vi "SR Service.vi"() -> ()   [LabVIEW 2012]
uses:
  user.lib/SpectralRadar.llb/Probe.lvclass
  user.lib/SpectralRadar.llb/Processing.lvclass
  user.lib/SpectralRadar.llb/Colored Data.lvclass
  user.lib/SpectralRadar.llb/Data.lvclass
  user.lib/SpectralRadar.llb/Scan Pattern.lvclass
  <vilib>/Math Plots/3D Math Plots/3D Surface/3D Surface XCtrl/3D Surface.xctl
  user.lib/SpectralRadar.llb/Device Property Int Selection.ctl
  user.lib/SpectralRadar.llb/Device Property Float Selection.ctl
  user.lib/SpectralRadar.llb/Colorscheme Selection.ctl
  user.lib/SpectralRadar.llb/Processing Flag Selection.ctl
  user.lib/SpectralRadar.llb/Coloring Byteorder.ctl
  <vilib>/Utility/error.llb/DialogType.ctl
  user.lib/SpectralRadar.llb/Probe Parameter Float Selection.ctl
  user.lib/SpectralRadar.llb/Calibration Selection.ctl
  user.lib/SpectralRadar.llb/Processing Parameter Int Selection.ctl
  user.lib/SpectralRadar.llb/Normal Direction Selection.ctl
  user.lib/SpectralRadar.llb/Data Analyzation Selection.ctl
  user.lib/SpectralRadar.llb/A-Scan Analysis Selection.ctl
  user.lib/SpectralRadar.llb/display Data 1D.vi
  user.lib/SpectralRadar.llb/set Scan Output.vi
  user.lib/SpectralRadar.llb/set Apodized Spectrum Output.vi
  user.lib/SpectralRadar.llb/display Data 2D as Surface.vi
  <vilib>/Utility/config.llb/Write Key (Double).vi
  user.lib/SpectralRadar.llb/set Spectrum Output.vi
  user.lib/SpectralRadar.llb/set Offset Corrected Spectrum Output.vi
  <vilib>/Analysis/baseanly.llb/Mean (DBL).vi
  <vilib>/Analysis/5stat.llb/RMS (DBL).vi
  user.lib/SpectralRadar.llb/LabVIEW Helper.lvlib
  user.lib/SpectralRadar.llb/OCT Device.lvclass
  user.lib/SpectralRadar.llb/Raw Data.lvclass
  <vilib>/Utility/config.llb/NI_LVConfig.lvlib
  user.lib/SpectralRadar.llb/ImageField.lvclass
  <vilib>/Analysis/NI_AALPro.lvlib
  user.lib/SpectralRadar.llb/Coloring.lvclass
  user.lib/SpectralRadar.llb/FullRange.lvclass
  <vilib>/Analysis/NI_AALBase.lvlib
panel:
  out "Scan Pattern":refnum<class "Scan Pattern.lvclass">
  out "Camera Image":refnum<class "Colored Data.lvclass">
  out "En face":refnum<class "Data.lvclass">
  out "Volume":refnum<class "Data.lvclass">
  out "Tmp":bool
  out "Colored Data":refnum<class "Colored Data.lvclass">
  out "Processing":refnum<class "Processing.lvclass">
  out "Probe":refnum<class "Probe.lvclass">
  in  "QuitApp":bool
  in  "SLD":bool
  out "SLDIndicator":bool
  in  "Tab Control":T1(tab)
  in  "Camera #":i32 min=0 max=1 step=1
  out "Selected Wavelength [nm]":dbl format="%#.1f"
  in  "Remove DC Spectrum":enum8{"False", "True", "Mixed"}(c332)=enum."True"
  in  "Filter Undersampl.":bool
  in  "Save Dispersion":bool
  in  "Dispersion Comp.":bool
  in  "Dispersion":bool
  in  "Options":bool
  in  "Zero Padding":i32=1 min=1 max=5000
  in  "Binning":i32=1 min=1 max=5000
  in  "SaveSpacingZ":bool
  out "Spacing Z [mm]":dbl format="%#_4g"
  out "Max Intensity":sgl=54929.0 format="%_3p"
  out "Min Intensity":sgl=54929.0 format="%_3p"
  in  "Extended":bool=TRUE
  in  "Dechirp":bool=TRUE
  in  "Apodization":bool=TRUE
  in  "Offset Error":bool=TRUE
  out "-40 dB [µm]":dbl=1600.0880126953125 format="%_3f"
  out "-20 dB [µm]":dbl=1569.837158203125 format="%_3f"
  out "-6 dB [µm]":dbl=1465.10693359375 format="%_3f"
  in  "Thickness Sample":dbl=1.0
  in  "z-Calibration":bool
  out "Noise [dB]":dbl=49.84672927856445 format="%_3f"
  out "Noise [e]":dbl=4474.02978515625 format="%_3p"
  out "Peak Pos. [Pixel]":dbl=474.0 format="%#_5g"
  out "Peak [dB]":dbl=61.309532165527344 format="%#_3g"
  in  "Power in Spectrometer [µW]":dbl=4.6 format="%.2p"
  out "Quantum eff. [%]":dbl=69.93751525878906 format="%.1f"
  out "RMS":dbl=1982809.125 format="%_3p"
  out "Min Contrast [%]":sgl=0.02587428 format="%.1g"
  out "Mean Contrast [%]":dbl=0.08312544226646423 format="%.1g"
  in  "LambdaToKLab":bool
  in  "Apodization":bool
  in  "OffsetErrors":bool
  out "Contrast":sgl[](graph)
  in  "Start Measurement":bool
  out "Meas. Indicator":bool
  out "SpectrumWithOffsetRemoved":dbl[](graph) caption="Spectrum with Offsets Removed"
  out "Apodized Spectrum":dbl[](graph)
  out "Spectrum":dbl[](graph)
  out "AScan":dbl[](graph) caption="A-Scan"
  in  "Window":T2(ring)
  in  "Save Dechirp":bool
  in  "Averaging":i32=1 min=1 max=5000
  in  "Center Wavelength [nm]":dbl=930.0 format="%.2p"
  in  "FullRange":bool
  in  "Log Button":bool
  in  "Clear All":bool
  in  "Select ADC 3":u16(ring) caption="Select ADC" items=["SLD 1 Current", "SLD 1 Peltier", "SLD 1 Power", "SLD 2 Current", "SLD 2 Peltier", "SLD 2 Power"]
  in  "Select ADC 2":u16(ring) caption="Select ADC" items=["SLD 1 Current", "SLD 1 Peltier", "SLD 1 Power", "SLD 2 Current", "SLD 2 Peltier", "SLD 2 Power"]
  in  "Select ADC 1":u16(ring) caption="Select ADC" items=["SLD 1 Current", "SLD 1 Peltier", "SLD 1 Power", "SLD 2 Current", "SLD 2 Peltier", "SLD 2 Power"]
  out "ADC 1":dbl(graph)
  out "ADC 3":dbl(graph)
  out "ADC 2":dbl(graph) caption="SLD1 Power"
  in  "Expansion Time [s]":dbl format="%#_6p"
  in  "Rotation Time [s]":dbl format="%#_6p"
  in  "Flyback Time [s]":dbl format="%#_6p"
  out "Y":dbl[][](graph)=[[-0.12456591788733773, -0.12456591788733773, -0.12456591788733773, -0.12488812549431395, -0.12392150267402412, -0.12424371028057446, -0.12424371028057446, -0.12424371028057446, -0.12456591788733773, -0.12488812549431395, -0.12392150267402412, -0.12359929506768669, -0.12488812549431395, -0.12456591788733773, -0.12392150267402412, -0.12456591788733773, -0.12424371028057446, -0.12392150267402412, -0.12488812549431395, -0.12424371028057446, -0.12424371028057446, -0.12521033310150315, -0.12424371028057446, -0.12392150267402412, -0.12488812549431395, -0.12295487985565048, -0.12424371028057446, -0.12392150267402412, -0.12424371028057446, -0.12488812549431395, -0.12392150267402412, -0.12392150267402412, -0.12456591788733773, -0.12424371028057446, -0.12424371028057446, -0.12392150267402412, -0.12424371028057446, -0.12521033310150315, -0.12392150267402412, -0.12359929506768669, -0.12392150267402412, -0.12424371028057446, -0.12424371028057446, -0.12424371028057446, -0.12392150267402412, -0.12488812549431395, -0.12392150267402412, -0.12424371028057446, -0.12392150267402412, -0.12456591788733773, -0.12456591788733773, -0.12359929506768669, -0.12424371028057446, -0.12456591788733773, -0.12424371028057446, -0.12424371028057446, -0.12488812549431395, -0.12424371028057446, -0.12392150267402412, -0.12392150267402412, -0.12424371028057446, -0.12392150267402412, -0.12553254070890535, -0.12392150267402412, -0.12392150267402412, -0.12488812549431395, -0.12392150267402412, -0.12392150267402412, -0.12392150267402412, -0.12424371028057446, -0.12359929506768669, -0.12392150267402412, -0.12392150267402412, -0.12521033310150315, -0.12359929506768669, -0.12424371028057446, -0.12456591788733773, -0.12424371028057446, -0.12392150267402412, -0.12359929506768669, -0.12424371028057446, -0.12456591788733773, -0.12456591788733773, -0.12392150267402412, -0.12456591788733773, -0.12392150267402412, -0.12392150267402412, -0.12392150267402412, -0.12456591788733773, -0.12456591788733773, -0.12424371028057446, -0.12392150267402412, -0.12456591788733773, -0.12424371028057446, -0.12456591788733773, -0.12359929506768669, -0.12456591788733773, -0.12456591788733773, -0.12392150267402412, -0.12488812549431395, -0.12456591788733773, -0.12456591788733773, -0.12392150267402412, -0.12456591788733773, -0.12456591788733773, -0.12359929506768669, -0.12424371028057446, -0.12359929506768669, -0.12424371028057446, -0.12424371028057446, -0.12424371028057446, -0.12392150267402412, -0.12456591788733773, -0.12488812549431395, -0.12295487985565048, -0.12392150267402412, -0.12456591788733773, -0.12456591788733773, -0.12392150267402412, -0.12424371028057446, -0.12488812549431395, -0.12327708746156214, -0.12456591788733773, -0.12424371028057446, -0.12424371028057446, -0.12424371028057446, -0.12424371028057446, -0.12392150267402412, -0.12392150267402412, -0.12392150267402412, -0.12392150267402412, -0.12392150267402412, -0.12456591788733773, -0.12456591788733773, -0.12392150267402412, -0.12392150267402412, -0.12456591788733773, -0.12359929506768669, -0.12488812549431395, -0.12456591788733773, -0.12295487985565048, -0.12359929506768669, -0.12424371028057446, -0.12392150267402412, -0.12488812549431395, -0.12456591788733773, -0.12392150267402412, -0.12424371028057446, -0.12424371028057446, -0.12392150267402412, -0.12456591788733773, -0.12392150267402412, -0.12488812549431395, -0.12392150267402412, -0.12521033310150315, -0.12424371028057446, -0.12521033310150315, -0.12456591788733773, -0.12392150267402412, -0.12521033310150315, -0.12424371028057446, -0.12424371028057446, -0.12456591788733773, -0.12424371028057446, -0.12456591788733773, -0.12456591788733773, -0.12359929506768669, -0.12488812549431395, -0.12456591788733773, -0.12456591788733773, -0.12424371028057446, -0.12456591788733773, -0.12359929506768669, -0.12424371028057446, -0.12424371028057446, -0.12392150267402412, -0.12456591788733773, -0.12359929506768669, -0.12392150267402412, -0.12521033310150315, -0.12424371028057446, -0.12521033310150315, -0.12456591788733773, -0.12521033310150315, -0.12392150267402412, -0.12488812549431395, -0.12392150267402412, -0.12488812549431395, -0.12456591788733773, -0.12359929506768669, -0.12424371028057446, -0.12456591788733773, -0.12488812549431395, -0.12392150267402412, -0.12456591788733773, -0.12521033310150315, -0.12327708746156214, -0.12456591788733773, -0.12359929506768669, -0.12488812549431395, -0.12392150267402412, -0.12456591788733773, -0.12392150267402412, -0.12456591788733773, -0.12424371028057446, -0.12424371028057446, -0.12424371028057446, -0.12456591788733773, -0.12392150267402412, -0.12392150267402412, -0.12359929506768669, -0.12488812549431395, -0.12456591788733773, -0.12359929506768669, -0.12424371028057446, -0.12392150267402412, -0.12359929506768669, -0.12424371028057446, -0.12392150267402412, -0.12424371028057446, -0.12424371028057446, -0.12424371028057446, -0.12488812549431395, -0.12456591788733773, -0.12424371028057446, -0.12392150267402412, -0.12392150267402412, -0.12456591788733773, -0.12456591788733773, -0.12456591788733773, -0.12456591788733773, -0.12424371028057446, -0.12424371028057446, -0.12359929506768669, -0.12424371028057446, -0.12456591788733773, -0.12327708746156214, -0.12456591788733773, -0.12424371028057446, -0.12456591788733773, -0.12456591788733773, -0.12392150267402412, -0.12424371028057446, -0.12488812549431395, -0.12456591788733773, -0.12359929506768669, -0.12521033310150315, -0.12424371028057446, -0.12327708746156214, -0.12424371028057446, -0.12456591788733773, -0.12392150267402412, -0.12488812549431395, -0.12392150267402412, -0.12392150267402412, -0.12488812549431395, -0.12424371028057446, -0.12392150267402412, -0.12488812549431395, -0.12521033310150315, -0.12456591788733773, -0.12424371028057446, -0.12456591788733773, -0.12424371028057446, -0.12392150267402412, -0.12424371028057446, -0.12359929506768669, -0.12456591788733773, -0.12424371028057446, -0.12424371028057446, -0.12456591788733773, -0.12424371028057446, -0.12392150267402412, -0.12488812549431395, -0.12392150267402412, -0.12392150267402412, -0.12424371028057446, -0.12359929506768669, -0.12521033310150315, -0.12424371028057446, -0.12392150267402412, -0.12424371028057446, -0.12456591788733773, -0.12424371028057446, -0.12521033310150315, -0.12392150267402412, -0.12488812549431395, -0.12521033310150315, -0.12359929506768669, -0.12424371028057446, -0.12488812549431395, -0.12456591788733773, -0.12424371028057446, -0.12424371028057446, -0.12488812549431395, -0.12359929506768669, -0.12327708746156214, -0.12488812549431395, -0.12456591788733773, -0.12424371028057446, -0.12456591788733773, -0.12456591788733773, -0.12456591788733773, -0.12392150267402412, -0.12392150267402412, -0.12392150267402412, -0.12488812549431395, -0.12392150267402412, -0.12424371028057446, -0.12424371028057446, -0.12424371028057446, -0.12424371028057446, -0.12424371028057446, -0.12488812549431395, -0.12392150267402412, -0.12424371028057446, -0.12392150267402412, -0.12424371028057446, -0.12392150267402412, -0.12424371028057446, -0.12392150267402412, -0.12392150267402412, -0.12456591788733773, -0.12424371028057446, -0.12327708746156214, -0.12521033310150315, -0.12392150267402412, -0.12392150267402412, -0.12392150267402412, -0.12456591788733773, -0.12359929506768669, -0.12456591788733773, -0.12424371028057446, -0.12424371028057446, -0.12456591788733773, -0.12392150267402412, -0.12424371028057446, -0.12359929506768669, -0.12456591788733773, -0.12456591788733773, -0.12392150267402412, -0.12424371028057446, -0.12456591788733773, -0.12359929506768669, -0.12488812549431395, -0.12456591788733773, -0.12424371028057446, -0.12424371028057446, -0.12456591788733773, -0.12424371028057446, -0.12424371028057446, -0.12456591788733773, -0.12327708746156214, -0.12392150267402412, -0.12392150267402412, -0.12424371028057446, -0.12359929506768669, -0.12488812549431395, -0.12424371028057446, -0.12424371028057446, -0.12392150267402412, -0.12456591788733773, -0.12424371028057446, -0.12359929506768669, -0.12359929506768669, -0.12456591788733773, -0.12456591788733773, -0.12456591788733773, -0.12392150267402412, -0.12488812549431395, -0.12392150267402412, -0.12424371028057446, -0.12359929506768669, -0.12456591788733773, -0.12424371028057446, -0.12424371028057446, -0.12456591788733773, -0.12424371028057446, -0.12359929506768669, -0.12392150267402412, -0.12456591788733773, -0.12521033310150315, -0.12327708746156214, -0.12392150267402412, -0.12424371028057446, -0.12488812549431395, -0.12424371028057446, -0.12359929506768669, -0.12392150267402412, -0.12488812549431395, -0.12392150267402412, -0.12424371028057446, -0.12392150267402412, -0.12456591788733773, -0.12359929506768669, -0.12424371028057446, -0.12392150267402412, -0.12424371028057446, -0.12456591788733773, -0.12456591788733773, -0.12424371028057446, -0.12456591788733773, -0.12392150267402412, -0.12392150267402412, -0.12424371028057446, -0.12392150267402412, -0.12392150267402412, -0.12424371028057446, -0.12424371028057446, -0.12424371028057446, -0.12424371028057446, -0.12488812549431395, -0.12424371028057446, -0.12392150267402412, -0.12456591788733773, -0.12359929506768669, -0.12488812549431395, -0.12424371028057446, -0.12424371028057446, -0.12521033310150315, -0.12488812549431395, -0.12424371028057446, -0.12456591788733773, -0.12488812549431395, -0.12456591788733773, -0.12488812549431395, -0.12488812549431395, -0.12424371028057446, -0.12424371028057446, -0.12392150267402412, -0.12392150267402412, -0.12392150267402412, -0.12488812549431395, -0.12327708746156214, -0.12553254070890535, -0.12359929506768669, -0.12456591788733773, -0.12456591788733773, -0.12327708746156214, -0.12424371028057446, -0.12456591788733773, -0.12359929506768669, -0.12392150267402412, -0.12424371028057446, -0.12488812549431395, -0.12585474831652058, -0.12359929506768669, -0.12424371028057446, -0.12521033310150315, -0.12327708746156214, -0.12424371028057446, -0.12424371028057446, -0.12392150267402412, -0.12488812549431395, -0.12359929506768669, -0.12456591788733773, -0.12424371028057446, -0.12359929506768669, -0.12456591788733773, -0.12488812549431395, -0.12488812549431395, -0.12456591788733773, -0.12392150267402412, -0.12424371028057446, -0.12392150267402412, -0.12488812549431395, -0.12456591788733773, -0.12392150267402412, -0.12456591788733773, -0.12424371028057446, -0.12392150267402412, -0.12456591788733773, -0.12392150267402412, -0.12327708746156214, -0.12521033310150315, -0.12424371028057446, -0.12424371028057446, -0.12392150267402412, -0.12456591788733773, -0.12392150267402412, -0.12456591788733773, -0.12456591788733773, -0.12327708746156214, -0.12456591788733773, -0.12424371028057446, -0.12392150267402412, -0.12424371028057446, -0.12424371028057446, -0.12424371028057446, -0.12392150267402412, -0.12327708746156214, -0.12456591788733773, -0.12456591788733773, -0.12359929506768669, -0.12456591788733773, -0.12392150267402412, -0.12392150267402412, -0.12488812549431395, -0.12456591788733773, -0.12424371028057446, -0.12488812549431395, -0.12327708746156214, -0.12456591788733773, -0.12456591788733773, -0.12424371028057446, -0.12359929506768669, -0.12392150267402412, -0.12456591788733773, -0.12424371028057446, -0.12392150267402412, -0.12392150267402412, -0.12424371028057446, -0.12456591788733773, -0.12359929506768669, -0.12424371028057446, -0.12521033310150315, -0.12359929506768669, -0.12424371028057446, -0.12359929506768669, -0.12359929506768669, -0.12424371028057446, -0.12424371028057446, -0.12456591788733773, -0.12456591788733773, -0.12456591788733773, -0.12424371028057446, -0.12392150267402412, -0.12488812549431395, -0.12424371028057446, -0.12456591788733773, -0.12424371028057446, -0.12521033310150315, -0.12456591788733773, -0.12456591788733773, -0.12521033310150315, -0.12488812549431395, -0.12456591788733773, -0.12359929506768669, -0.12521033310150315, -0.12456591788733773, -0.12392150267402412, -0.12456591788733773, -0.12359929506768669, -0.12424371028057446, -0.12488812549431395, -0.12392150267402412, -0.12392150267402412, -0.12456591788733773, -0.12456591788733773, -0.12488812549431395, -0.12392150267402412, -0.12424371028057446, -0.12424371028057446, -0.12359929506768669, -0.12392150267402412, -0.12424371028057446, -0.12424371028057446, -0.12456591788733773, -0.12488812549431395, -0.12488812549431395, -0.12456591788733773, -0.12424371028057446, -0.12392150267402412, -0.12456591788733773, -0.12392150267402412, -0.12392150267402412, -0.12488812549431395, -0.12488812549431395, -0.12359929506768669, -0.12424371028057446, -0.12424371028057446, -0.12392150267402412, -0.12456591788733773, -0.12424371028057446, -0.12488812549431395, -0.12521033310150315, -0.12424371028057446, -0.12359929506768669, -0.12456591788733773, -0.12456591788733773, -0.12424371028057446, -0.12424371028057446, -0.12456591788733773, -0.12359929506768669, -0.12424371028057446, -0.12424371028057446, -0.12424371028057446, -0.12456591788733773, -0.12456591788733773, -0.12392150267402412, -0.12456591788733773, -0.12456591788733773, -0.12424371028057446, -0.12359929506768669, -0.12553254070890535, -0.12456591788733773, -0.12456591788733773, -0.12456591788733773, -0.12456591788733773, -0.12392150267402412, -0.12424371028057446, -0.12424371028057446, -0.12488812549431395, -0.12424371028057446, -0.12488812549431395, -0.12392150267402412, -0.12456591788733773, -0.12456591788733773, -0.12456591788733773, -0.12392150267402412, -0.12488812549431395, -0.12392150267402412, -0.12392150267402412, -0.12456591788733773, -0.12424371028057446, -0.12456591788733773, -0.12327708746156214, -0.12488812549431395, -0.12392150267402412, -0.12359929506768669, -0.12488812549431395, -0.12392150267402412, -0.12424371028057446, -0.12456591788733773, -0.12456591788733773, -0.12359929506768669, -0.12488812549431395, -0.12424371028057446, -0.12359929506768669, -0.12456591788733773, -0.12521033310150315, -0.12359929506768669, -0.12456591788733773, -0.12392150267402412, -0.12488812549431395, -0.12327708746156214, -0.12456591788733773, -0.12456591788733773, -0.12392150267402412, -0.12488812549431395, -0.12392150267402412, -0.12456591788733773, -0.12424371028057446, -0.12392150267402412, -0.12359929506768669, -0.12553254070890535, -0.12392150267402412, -0.12424371028057446, -0.12392150267402412, -0.12456591788733773, -0.12424371028057446, -0.12424371028057446, -0.12424371028057446, -0.12456591788733773, -0.12424371028057446, -0.12456591788733773, -0.12424371028057446, -0.12424371028057446, -0.12359929506768669, -0.12392150267402412, -0.12456591788733773, -0.12456591788733773, -0.12488812549431395, -0.12359929506768669, -0.12424371028057446, -0.12456591788733773, -0.12424371028057446, -0.12359929506768669, -0.12327708746156214, -0.12392150267402412, -0.12456591788733773, -0.12392150267402412, -0.12488812549431395, -0.12456591788733773, -0.12392150267402412, -0.12424371028057446, -0.12359929506768669, -0.12456591788733773, -0.12424371028057446, -0.12456591788733773, -0.12392150267402412, -0.12456591788733773, -0.12456591788733773, -0.12424371028057446, -0.12392150267402412, -0.12424371028057446, -0.12359929506768669, -0.12456591788733773, -0.12424371028057446, -0.12488812549431395, -0.12488812549431395, -0.12392150267402412, -0.12424371028057446, -0.12521033310150315, -0.12359929506768669, -0.12327708746156214, -0.12424371028057446, -0.12456591788733773, -0.12456591788733773, -0.12424371028057446, -0.12392150267402412, -0.12521033310150315, -0.12392150267402412, -0.12456591788733773, -0.12424371028057446, -0.12392150267402412, -0.12424371028057446, -0.12488812549431395, -0.12295487985565048, -0.12521033310150315, -0.12424371028057446, -0.12424371028057446, -0.12456591788733773, -0.12456591788733773, -0.12359929506768669, -0.12456591788733773, -0.12424371028057446, -0.12456591788733773, -0.12424371028057446, -0.12327708746156214, -0.12488812549431395, -0.12424371028057446, -0.12392150267402412, -0.12456591788733773, -0.12424371028057446, -0.12424371028057446, -0.12424371028057446, -0.12456591788733773, -0.12424371028057446, -0.12456591788733773, -0.12424371028057446, -0.12359929506768669, -0.12424371028057446, -0.12392150267402412, -0.12392150267402412, -0.12424371028057446, -0.12456591788733773, -0.12392150267402412, -0.12424371028057446, -0.12392150267402412, -0.12424371028057446, -0.12456591788733773, -0.12424371028057446, -0.12456591788733773, -0.12392150267402412, -0.12456591788733773, -0.12521033310150315, -0.12392150267402412, -0.12456591788733773, -0.12488812549431395, -0.12424371028057446, -0.12424371028057446, -0.12392150267402412, -0.12424371028057446, -0.12392150267402412, -0.12424371028057446, -0.12392150267402412, -0.12424371028057446, -0.12424371028057446, -0.12456591788733773, -0.12424371028057446, -0.12359929506768669, -0.12456591788733773, -0.12359929506768669, -0.12456591788733773, -0.12424371028057446, -0.12424371028057446, -0.12359929506768669, -0.12456591788733773, -0.12424371028057446, -0.12392150267402412, -0.12424371028057446, -0.12392150267402412, -0.12392150267402412, -0.12359929506768669, -0.12424371028057446, -0.12456591788733773, -0.12392150267402412, -0.12456591788733773, -0.12392150267402412, -0.12392150267402412, -0.12424371028057446, -0.12456591788733773, -0.12424371028057446, -0.12456591788733773, -0.12392150267402412, -0.12521033310150315, -0.12359929506768669, -0.12456591788733773, -0.12359929506768669, -0.12392150267402412, -0.12488812549431395, -0.12488812549431395, -0.12424371028057446, -0.12456591788733773, -0.12424371028057446, -0.12424371028057446, -0.12424371028057446, -0.12359929506768669, -0.12424371028057446, -0.12456591788733773, -0.12456591788733773, -0.12327708746156214, -0.12424371028057446, -0.12456591788733773, -0.12521033310150315, -0.12424371028057446, -0.12424371028057446, -0.12424371028057446, -0.12456591788733773, -0.12424371028057446, -0.12456591788733773, -0.12456591788733773, -0.12521033310150315, -0.12456591788733773, -0.12392150267402412, -0.12392150267402412, -0.12424371028057446, -0.12327708746156214, -0.12424371028057446, -0.12456591788733773, -0.12424371028057446, -0.12392150267402412, -0.12392150267402412, -0.12424371028057446, -0.12392150267402412, -0.12456591788733773, -0.12488812549431395, -0.12359929506768669, -0.12456591788733773, -0.12424371028057446, -0.12456591788733773, -0.12392150267402412, -0.12456591788733773, -0.12359929506768669, -0.12392150267402412, -0.12456591788733773, -0.12424371028057446, -0.12392150267402412, -0.12456591788733773, -0.12488812549431395, -0.12424371028057446, -0.12359929506768669, -0.12488812549431395, -0.12392150267402412, -0.12424371028057446, -0.12424371028057446, -0.12359929506768669, -0.12456591788733773, -0.12392150267402412, -0.12424371028057446, -0.12488812549431395, -0.12456591788733773, -0.12392150267402412, -0.12488812549431395, -0.12488812549431395, -0.12392150267402412, -0.12424371028057446, -0.12392150267402412, -0.12488812549431395, -0.12392150267402412, -0.12424371028057446, -0.12392150267402412, -0.12488812549431395, -0.12424371028057446, -0.12424371028057446, -0.12456591788733773, -0.12456591788733773, -0.12359929506768669, -0.12521033310150315, -0.12359929506768669, -0.12521033310150315, -0.12424371028057446, -0.12392150267402412, -0.12424371028057446, -0.12456591788733773, -0.12456591788733773, -0.12456591788733773, -0.12359929506768669, -0.12488812549431395, -0.12424371028057446, -0.12392150267402412, -0.12392150267402412, -0.12456591788733773, -0.12424371028057446, -0.12392150267402412, -0.12424371028057446, -0.12521033310150315, -0.12327708746156214, -0.12424371028057446, -0.12359929506768669, -0.12359929506768669, -0.12359929506768669, -0.12424371028057446, -0.12327708746156214, -0.12585474831652058, -0.12456591788733773, -0.12424371028057446, -0.12456591788733773, -0.12392150267402412, -0.12424371028057446, -0.12456591788733773, -0.12392150267402412, -0.12456591788733773, -0.12456591788733773, -0.12327708746156214, -0.12488812549431395, -0.12521033310150315, -0.12392150267402412, -0.12456591788733773, -0.12359929506768669, -0.12521033310150315, -0.12424371028057446, -0.12392150267402412, -0.12424371028057446, -0.12456591788733773, -0.12392150267402412, -0.12521033310150315, -0.12392150267402412, -0.12424371028057446, -0.12424371028057446, -0.12424371028057446, -0.12456591788733773, -0.12424371028057446, -0.12327708746156214, -0.12424371028057446, -0.12424371028057446, -0.12456591788733773, -0.12456591788733773, -0.12392150267402412, -0.12488812549431395, -0.12392150267402412, -0.12392150267402412, -0.12392150267402412, -0.12488812549431395, -0.12488812549431395, -0.12359929506768669, -0.12456591788733773, -0.12424371028057446, -0.12392150267402412, -0.12456591788733773, -0.12456591788733773, -0.12424371028057446, -0.12456591788733773, -0.12424371028057446, -0.12359929506768669, -0.12424371028057446, -0.12456591788733773, -0.12424371028057446, -0.12392150267402412, -0.12488812549431395, -0.12456591788733773, -0.12359929506768669, -0.12456591788733773, -0.12456591788733773, -0.12456591788733773, -0.12392150267402412, -0.12359929506768669, -0.12456591788733773, -0.12424371028057446, -0.12424371028057446, -0.12392150267402412, -0.12456591788733773, -0.12424371028057446, -0.12424371028057446, -0.12424371028057446, -0.12392150267402412, -0.12456591788733773, -0.12424371028057446, -0.12392150267402412, -0.12424371028057446, -0.12392150267402412, -0.12327708746156214, -0.12359929506768669, -0.12424371028057446, -0.12392150267402412, -0.12424371028057446, -0.12488812549431395, -0.12424371028057446, -0.12392150267402412, -0.12456591788733773, -0.12392150267402412, -0.12521033310150315, -0.12392150267402412, -0.12424371028057446, -0.12359929506768669, -0.12456591788733773, -0.12359929506768669, -0.12424371028057446, -0.12392150267402412, -0.12456591788733773, -0.12424371028057446, -0.12359929506768669, -0.12424371028057446, -0.12456591788733773, -0.12424371028057446, -0.12424371028057446, -0.12424371028057446, -0.12488812549431395, -0.12456591788733773, -0.12424371028057446, -0.12456591788733773, -0.12359929506768669, -0.12456591788733773, -0.12456591788733773, -0.12456591788733773, -0.12456591788733773, -0.12359929506768669, -0.12424371028057446, -0.12359929506768669, -0.12327708746156214, -0.12424371028057446, -0.12392150267402412, -0.12488812549431395, -0.12488812549431395, -0.12359929506768669, -0.12456591788733773, -0.12488812549431395, -0.12488812549431395, -0.12392150267402412, -0.12424371028057446, -0.12456591788733773, -0.12424371028057446, -0.12424371028057446, -0.12392150267402412, -0.12617695592434883, -0.12424371028057446, -0.12392150267402412, -0.12359929506768669, -0.12553254070890535, -0.12392150267402412, -0.12424371028057446, -0.12424371028057446, -0.12456591788733773, -0.12392150267402412, -0.12488812549431395, -0.12456591788733773, -0.12424371028057446, -0.12392150267402412, -0.12521033310150315, -0.12359929506768669, -0.12488812549431395, -0.12392150267402412, -0.12456591788733773, -0.12424371028057446, -0.12488812549431395, -0.12456591788733773, -0.12359929506768669, -0.12424371028057446, -0.12521033310150315, -0.12424371028057446, -0.12359929506768669, -0.12392150267402412, -0.12488812549431395, -0.12327708746156214, -0.12456591788733773, -0.12424371028057446, -0.12456591788733773, -0.12456591788733773, -0.12359929506768669, -0.12392150267402412, -0.12456591788733773, -0.12359929506768669, -0.12359929506768669, -0.12456591788733773, -0.12488812549431395, -0.12553254070890535, -0.12456591788733773, -0.12392150267402412, -0.12424371028057446, -0.12327708746156214, -0.12456591788733773, -0.12392150267402412, -0.12424371028057446, -0.12392150267402412, -0.12424371028057446, -0.12424371028057446, -0.12392150267402412, -0.12359929506768669, -0.12456591788733773, -0.12456591788733773, -0.12424371028057446, -0.12392150267402412, -0.12392150267402412, -0.12392150267402412, -0.12424371028057446, -0.12392150267402412, -0.12392150267402412, -0.12488812549431395, -0.12456591788733773, -0.12392150267402412, -0.12456591788733773, -0.12359929506768669, -0.12456591788733773, -0.12359929506768669, -0.12392150267402412, -0.12488812549431395, -0.12456591788733773, -0.12359929506768669, -0.12424371028057446, -0.12392150267402412, -0.12488812549431395, -0.12424371028057446, -0.12488812549431395, -0.12392150267402412, -0.12488812549431395, -0.12488812549431395, -0.12392150267402412, -0.12521033310150315, -0.12424371028057446, -0.12359929506768669, -0.12456591788733773, -0.12456591788733773, -0.12359929506768669, -0.12392150267402412, -0.12392150267402412, -0.12456591788733773, -0.12488812549431395, -0.12295487985565048, -0.12424371028057446, -0.12392150267402412, -0.12359929506768669, -0.12456591788733773, -0.12424371028057446, -0.12456591788733773, -0.12456591788733773, -0.12392150267402412, -0.12392150267402412, -0.12488812549431395, -0.12359929506768669, -0.12456591788733773, -0.12392150267402412, -0.12456591788733773, -0.12488812549431395, -0.12424371028057446, -0.12424371028057446, -0.12424371028057446, -0.12392150267402412, -0.12424371028057446, -0.12424371028057446, -0.12359929506768669, -0.12392150267402412, -0.12392150267402412, -0.12488812549431395, -0.12456591788733773, -0.12424371028057446, -0.12456591788733773, -0.12392150267402412, -0.12456591788733773, -0.12359929506768669, -0.12392150267402412, -0.12392150267402412, -0.12424371028057446, -0.12424371028057446, -0.12488812549431395, -0.12424371028057446, -0.12456591788733773, -0.12392150267402412, -0.12456591788733773, -0.12359929506768669, -0.12424371028057446, -0.12456591788733773, -0.12359929506768669, -0.12456591788733773, -0.12424371028057446, -0.12392150267402412, -0.12456591788733773, -0.12424371028057446, -0.12488812549431395, -0.12359929506768669, -0.12392150267402412, -0.12456591788733773, -0.12456591788733773, -0.12295487985565048, -0.12488812549431395, -0.12456591788733773, -0.12521033310150315, -0.12424371028057446, -0.12392150267402412, -0.12424371028057446, -0.12456591788733773, -0.12456591788733773, -0.12392150267402412, -0.12424371028057446, -0.12488812549431395, -0.12359929506768669, -0.12359929506768669, -0.12456591788733773, -0.12424371028057446, -0.12359929506768669, -0.12359929506768669, -0.12488812549431395, -0.12424371028057446, -0.12456591788733773, -0.12359929506768669, -0.12456591788733773, -0.12521033310150315, -0.12456591788733773, -0.12424371028057446, -0.12456591788733773, -0.12392150267402412, -0.12392150267402412, -0.12392150267402412, -0.12424371028057446, -0.12488812549431395, -0.12392150267402412, -0.12456591788733773, -0.12392150267402412, -0.12424371028057446, -0.12424371028057446, -0.12392150267402412, -0.12392150267402412, -0.12424371028057446, -0.12456591788733773, -0.12456591788733773, -0.12456591788733773, -0.12488812549431395, -0.12424371028057446, -0.12359929506768669, -0.12488812549431395, -0.12424371028057446, -0.12392150267402412, -0.12521033310150315, -0.12424371028057446, -0.12392150267402412, -0.12392150267402412, -0.12456591788733773, -0.12488812549431395, -0.12424371028057446, -0.12424371028057446, -0.12392150267402412, -0.12424371028057446, -0.12456591788733773, -0.12456591788733773, -0.12456591788733773, -0.12424371028057446, -0.12521033310150315, -0.12295487985565048, -0.12456591788733773, -0.12424371028057446, -0.12424371028057446, -0.12392150267402412, -0.12488812549431395], [0.0, 0.0, 0.0, 0.0, 0.0, 0.0, 0.0, 0.0, 0.0, 0.0, 0.0, 0.0, 0.0, 0.0, 0.0, 0.0, 0.0, 0.0, 0.0, 0.0, 0.0, 0.0, 0.0, 0.0, 0.0, 0.0, 0.0, 0.0, 0.0, 0.0, 0.0, 0.0, 0.0, 0.0, 0.0, 0.0, 0.0, 0.0, 0.0, 0.0, 0.0, 0.0, 0.0, 0.0, 0.0, 0.0, 0.0, 0.0, 0.0, 0.0, 0.0, 0.0, 0.0, 0.0, 0.0, 0.0, 0.0, 0.0, 0.0, 0.0, 0.0, 0.0, 0.0, 0.0, 0.0, 0.0, 0.0, 0.0, 0.0, 0.0, 0.0, 0.0, 0.0, 0.0, 0.0, 0.0, 0.0, 0.0, 0.0, 0.0, 0.0, 0.0, 0.0, 0.0, 0.0, 0.0, 0.0, 0.0, 0.0, 0.0, 0.0, 0.0, 0.0, 0.0, 0.0, 0.0, 0.0, 0.0, 0.0, 0.0, 0.0, 0.0, 0.0, 0.0, 0.0, 0.0, 0.0, 0.0, 0.0, 0.0, 0.0, 0.0, 0.0, 0.0, 0.0, 0.0, 0.0, 0.0, 0.0, 0.0, 0.0, 0.0, 0.0, 0.0, 0.0, 0.0, 0.0, 0.0, 0.0, 0.0, 0.0, 0.0, 0.0, 0.0, 0.0, 0.0, 0.0, 0.0, 0.0, 0.0, 0.0, 0.0, 0.0, 0.0, 0.0, 0.0, 0.0, 0.0, 0.0, 0.0, 0.0, 0.0, 0.0, 0.0, 0.0, 0.0, 0.0, 0.0, 0.0, 0.0, 0.0, 0.0, 0.0, 0.0, 0.0, 0.0, 0.0, 0.0, 0.0, 0.0, 0.0, 0.0, 0.0, 0.0, 0.0, 0.0, 0.0, 0.0, 0.0, 0.0, 0.0, 0.0, 0.0, 0.0, 0.0, 0.0, 0.0, 0.0, 0.0, 0.0, 0.0, 0.0, 0.0, 0.0, 0.0, 0.0, 0.0, 0.0, 0.0, 0.0, 0.0, 0.0, 0.0, 0.0, 0.0, 0.0, 0.0, 0.0, 0.0, 0.0, 0.0, 0.0, 0.0, 0.0, 0.0, 0.0, 0.0, 0.0, 0.0, 0.0, 0.0, 0.0, 0.0, 0.0, 0.0, 0.0, 0.0, 0.0, 0.0, 0.0, 0.0, 0.0, 0.0, 0.0, 0.0, 0.0, 0.0, 0.0, 0.0, 0.0, 0.0, 0.0, 0.0, 0.0, 0.0, 0.0, 0.0, 0.0, 0.0, 0.0, 0.0, 0.0, 0.0, 0.0, 0.0, 0.0, 0.0, 0.0, 0.0, 0.0, 0.0, 0.0, 0.0, 0.0, 0.0, 0.0, 0.0, 0.0, 0.0, 0.0, 0.0, 0.0, 0.0, 0.0, 0.0, 0.0, 0.0, 0.0, 0.0, 0.0, 0.0, 0.0, 0.0, 0.0, 0.0, 0.0, 0.0, 0.0, 0.0, 0.0, 0.0, 0.0, 0.0, 0.0, 0.0, 0.0, 0.0, 0.0, 0.0, 0.0, 0.0, 0.0, 0.0, 0.0, 0.0, 0.0, 0.0, 0.0, 0.0, 0.0, 0.0, 0.0, 0.0, 0.0, 0.0, 0.0, 0.0, 0.0, 0.0, 0.0, 0.0, 0.0, 0.0, 0.0, 0.0, 0.0, 0.0, 0.0, 0.0, 0.0, 0.0, 0.0, 0.0, 0.0, 0.0, 0.0, 0.0, 0.0, 0.0, 0.0, 0.0, 0.0, 0.0, 0.0, 0.0, 0.0, 0.0, 0.0, 0.0, 0.0, 0.0, 0.0, 0.0, 0.0, 0.0, 0.0, 0.0, 0.0, 0.0, 0.0, 0.0, 0.0, 0.0, 0.0, 0.0, 0.0, 0.0, 0.0, 0.0, 0.0, 0.0, 0.0, 0.0, 0.0, 0.0, 0.0, 0.0, 0.0, 0.0, 0.0, 0.0, 0.0, 0.0, 0.0, 0.0, 0.0, 0.0, 0.0, 0.0, 0.0, 0.0, 0.0, 0.0, 0.0, 0.0, 0.0, 0.0, 0.0, 0.0, 0.0, 0.0, 0.0, 0.0, 0.0, 0.0, 0.0, 0.0, 0.0, 0.0, 0.0, 0.0, 0.0, 0.0, 0.0, 0.0, 0.0, 0.0, 0.0, 0.0, 0.0, 0.0, 0.0, 0.0, 0.0, 0.0, 0.0, 0.0, 0.0, 0.0, 0.0, 0.0, 0.0, 0.0, 0.0, 0.0, 0.0, 0.0, 0.0, 0.0, 0.0, 0.0, 0.0, 0.0, 0.0, 0.0, 0.0, 0.0, 0.0, 0.0, 0.0, 0.0, 0.0, 0.0, 0.0, 0.0, 0.0, 0.0, 0.0, 0.0, 0.0, 0.0, 0.0, 0.0, 0.0, 0.0, 0.0, 0.0, 0.0, 0.0, 0.0, 0.0, 0.0, 0.0, 0.0, 0.0, 0.0, 0.0, 0.0, 0.0, 0.0, 0.0, 0.0, 0.0, 0.0, 0.0, 0.0, 0.0, 0.0, 0.0, 0.0, 0.0, 0.0, 0.0, 0.0, 0.0, 0.0, 0.0, 0.0, 0.0, 0.0, 0.0, 0.0, 0.0, 0.0, 0.0, 0.0, 0.0, 0.0, 0.0, 0.0, 0.0, 0.0, 0.0, 0.0, 0.0, 0.0, 0.0, 0.0, 0.0, 0.0, 0.0, 0.0, 0.0, 0.0, 0.0, 0.0, 0.0, 0.0, 0.0, 0.0, 0.0, 0.0, 0.0, 0.0, 0.0, 0.0, 0.0, 0.0, 0.0, 0.0, 0.0, 0.0, 0.0, 0.0, 0.0, 0.0, 0.0, 0.0, 0.0, 0.0, 0.0, 0.0, 0.0, 0.0, 0.0, 0.0, 0.0, 0.0, 0.0, 0.0, 0.0, 0.0, 0.0, 0.0, 0.0, 0.0, 0.0, 0.0, 0.0, 0.0, 0.0, 0.0, 0.0, 0.0, 0.0, 0.0, 0.0, 0.0, 0.0, 0.0, 0.0, 0.0, 0.0, 0.0, 0.0, 0.0, 0.0, 0.0, 0.0, 0.0, 0.0, 0.0, 0.0, 0.0, 0.0, 0.0, 0.0, 0.0, 0.0, 0.0, 0.0, 0.0, 0.0, 0.0, 0.0, 0.0, 0.0, 0.0, 0.0, 0.0, 0.0, 0.0, 0.0, 0.0, 0.0, 0.0, 0.0, 0.0, 0.0, 0.0, 0.0, 0.0, 0.0, 0.0, 0.0, 0.0, 0.0, 0.0, 0.0, 0.0, 0.0, 0.0, 0.0, 0.0, 0.0, 0.0, 0.0, 0.0, 0.0, 0.0, 0.0, 0.0, 0.0, 0.0, 0.0, 0.0, 0.0, 0.0, 0.0, 0.0, 0.0, 0.0, 0.0, 0.0, 0.0, 0.0, 0.0, 0.0, 0.0, 0.0, 0.0, 0.0, 0.0, 0.0, 0.0, 0.0, 0.0, 0.0, 0.0, 0.0, 0.0, 0.0, 0.0, 0.0, 0.0, 0.0, 0.0, 0.0, 0.0, 0.0, 0.0, 0.0, 0.0, 0.0, 0.0, 0.0, 0.0, 0.0, 0.0, 0.0, 0.0, 0.0, 0.0, 0.0, 0.0, 0.0, 0.0, 0.0, 0.0, 0.0, 0.0, 0.0, 0.0, 0.0, 0.0, 0.0, 0.0, 0.0, 0.0, 0.0, 0.0, 0.0, 0.0, 0.0, 0.0, 0.0, 0.0, 0.0, 0.0, 0.0, 0.0, 0.0, 0.0, 0.0, 0.0, 0.0, 0.0, 0.0, 0.0, 0.0, 0.0, 0.0, 0.0, 0.0, 0.0, 0.0, 0.0, 0.0, 0.0, 0.0, 0.0, 0.0, 0.0, 0.0, 0.0, 0.0, 0.0, 0.0, 0.0, 0.0, 0.0, 0.0, 0.0, 0.0, 0.0, 0.0, 0.0, 0.0, 0.0, 0.0, 0.0, 0.0, 0.0, 0.0, 0.0, 0.0, 0.0, 0.0, 0.0, 0.0, 0.0, 0.0, 0.0, 0.0, 0.0, 0.0, 0.0, 0.0, 0.0, 0.0, 0.0, 0.0, 0.0, 0.0, 0.0, 0.0, 0.0, 0.0, 0.0, 0.0, 0.0, 0.0, 0.0, 0.0, 0.0, 0.0, 0.0, 0.0, 0.0, 0.0, 0.0, 0.0, 0.0, 0.0, 0.0, 0.0, 0.0, 0.0, 0.0, 0.0, 0.0, 0.0, 0.0, 0.0, 0.0, 0.0, 0.0, 0.0, 0.0, 0.0, 0.0, 0.0, 0.0, 0.0, 0.0, 0.0, 0.0, 0.0, 0.0, 0.0, 0.0, 0.0, 0.0, 0.0, 0.0, 0.0, 0.0, 0.0, 0.0, 0.0, 0.0, 0.0, 0.0, 0.0, 0.0, 0.0, 0.0, 0.0, 0.0, 0.0, 0.0, 0.0, 0.0, 0.0, 0.0, 0.0, 0.0, 0.0, 0.0, 0.0, 0.0, 0.0, 0.0, 0.0, 0.0, 0.0, 0.0, 0.0, 0.0, 0.0, 0.0, 0.0, 0.0, 0.0, 0.0, 0.0, 0.0, 0.0, 0.0, 0.0, 0.0, 0.0, 0.0, 0.0, 0.0, 0.0, 0.0, 0.0, 0.0, 0.0, 0.0, 0.0, 0.0, 0.0, 0.0, 0.0, 0.0, 0.0, 0.0, 0.0, 0.0, 0.0, 0.0, 0.0, 0.0, 0.0, 0.0, 0.0, 0.0, 0.0, 0.0, 0.0, 0.0, 0.0, 0.0, 0.0, 0.0, 0.0, 0.0, 0.0, 0.0, 0.0, 0.0, 0.0, 0.0, 0.0, 0.0, 0.0, 0.0, 0.0, 0.0, 0.0, 0.0, 0.0, 0.0, 0.0, 0.0, 0.0, 0.0, 0.0, 0.0, 0.0, 0.0, 0.0, 0.0, 0.0, 0.0, 0.0, 0.0, 0.0, 0.0, 0.0, 0.0, 0.0, 0.0, 0.0, 0.0, 0.0, 0.0, 0.0, 0.0, 0.0, 0.0, 0.0, 0.0, 0.0, 0.0, 0.0, 0.0, 0.0, 0.0, 0.0, 0.0, 0.0, 0.0, 0.0, 0.0, 0.0, 0.0, 0.0, 0.0, 0.0, 0.0, 0.0, 0.0, 0.0, 0.0, 0.0, 0.0, 0.0, 0.0, 0.0, 0.0, 0.0, 0.0, 0.0, 0.0, 0.0, 0.0, 0.0, 0.0, 0.0, 0.0, 0.0, 0.0, 0.0, 0.0, 0.0, 0.0, 0.0, 0.0, 0.0, 0.0, 0.0, 0.0, 0.0, 0.0, 0.0, 0.0, 0.0, 0.0, 0.0, 0.0, 0.0, 0.0, 0.0, 0.0, 0.0, 0.0, 0.0, 0.0, 0.0, 0.0, 0.0, 0.0, 0.0, 0.0, 0.0, 0.0, 0.0, 0.0, 0.0, 0.0, 0.0, 0.0, 0.0, 0.0, 0.0, 0.0, 0.0, 0.0, 0.0, 0.0, 0.0, 0.0, 0.0, 0.0, 0.0, 0.0, 0.0, 0.0, 0.0, 0.0, 0.0, 0.0, 0.0, 0.0, 0.0, 0.0, 0.0, 0.0, 0.0, 0.0, 0.0, 0.0, 0.0, 0.0, 0.0, 0.0, 0.0, 0.0, 0.0, 0.0, 0.0, 0.0, 0.0, 0.0, 0.0, 0.0, 0.0, 0.0, 0.0, 0.0, 0.0, 0.0, 0.0, 0.0, 0.0, 0.0, 0.0, 0.0, 0.0, 0.0, 0.0, 0.0, 0.0, 0.0, 0.0, 0.0, 0.0, 0.0, 0.0, 0.0, 0.0, 0.0, 0.0, 0.0, 0.0, 0.0, 0.0, 0.0, 0.0, 0.0, 0.0, 0.0, 0.0, 0.0, 0.0, 0.0, 0.0, 0.0, 0.0, 0.0, 0.0, 0.0, 0.0, 0.0, 0.0, 0.0, 0.0, 0.0, 0.0, 0.0, 0.0, 0.0, 0.0, 0.0, 0.0, 0.0, 0.0, 0.0, 0.0, 0.0, 0.0, 0.0, 0.0, 0.0, 0.0, 0.0, 0.0, 0.0, 0.0, 0.0, 0.0, 0.0, 0.0, 0.0, 0.0, 0.0, 0.0, 0.0, 0.0, 0.0, 0.0, 0.0, 0.0, 0.0, 0.0, 0.0, 0.0, 0.0, 0.0, 0.0, 0.0, 0.0, 0.0, 0.0, 0.0, 0.0, 0.0, 0.0, 0.0, 0.0, 0.0, 0.0, 0.0, 0.0, 0.0, 0.0, 0.0, 0.0, 0.0, 0.0, 0.0, 0.0, 0.0, 0.0, 0.0, 0.0, 0.0, 0.0, 0.0, 0.0, 0.0, 0.0, 0.0, 0.0, 0.0, 0.0, 0.0, 0.0, 0.0, 0.0, 0.0, 0.0, 0.0, 0.0, 0.0, 0.0, 0.0, 0.0, 0.0, 0.0, 0.0, 0.0, 0.0, 0.0, 0.0, 0.0, 0.0, 0.0, 0.0, 0.0], [nan, nan, nan, nan, nan, nan, nan, nan, nan, nan, nan, nan, nan, nan, nan, nan, nan, nan, nan, nan, nan, nan, nan, nan, nan, nan, nan, nan, nan, nan, nan, nan, nan, nan, nan, nan, nan, nan, nan, nan, nan, nan, nan, nan, nan, nan, nan, nan, nan, nan, nan, nan, nan, nan, nan, nan, nan, nan, nan, nan, nan, nan, nan, nan, nan, nan, nan, nan, nan, nan, nan, nan, nan, nan, nan, nan, nan, nan, nan, nan, nan, nan, nan, nan, nan, nan, nan, nan, nan, nan, nan, nan, nan, nan, nan, nan, nan, 0.0, 0.0, 0.0, 0.0, 0.0, 0.0, 0.0, 0.0, 0.0, 0.0, 0.0, 0.0, 0.0, 0.0, 0.0, 0.0, 0.0, 0.0, 0.0, 0.0, 0.0, 0.0, 0.0, 0.0, 0.0, nan, nan, nan, nan, nan, nan, nan, nan, nan, nan, nan, nan, nan, nan, nan, nan, nan, nan, nan, nan, nan, nan, nan, nan, nan, nan, nan, nan, nan, nan, nan, nan, nan, nan, nan, nan, nan, nan, nan, nan, nan, nan, nan, nan, nan, nan, nan, nan, nan, nan, nan, nan, nan, nan, nan, nan, nan, nan, nan, nan, nan, nan, nan, nan, nan, nan, nan, nan, nan, nan, nan, nan, nan, nan, nan, nan, nan, nan, nan, nan, nan, nan, nan, nan, nan, nan, nan, nan, nan, nan, nan, nan, nan, nan, nan, nan, nan, 0.0, 0.0, 0.0, 0.0, 0.0, 0.0, 0.0, 0.0, 0.0, 0.0, 0.0, 0.0, 0.0, 0.0, 0.0, 0.0, 0.0, 0.0, 0.0, 0.0, 0.0, 0.0, 0.0, 0.0, 0.0, 0.0, 0.0, 0.0, 0.0, 0.0, 0.0, 0.0, 0.0, 0.0, 0.0, 0.0, 0.0, 0.0, 0.0, 0.0, 0.0, 0.0, 0.0, 0.0, 0.0, 0.0, 0.0, 0.0, 0.0, 0.0, 0.0, 0.0, 0.0, 0.0, 0.0, 0.0, 0.0, 0.0, 0.0, 0.0, 0.0, 0.0, 0.0, 0.0, 0.0, 0.0, 0.0, 0.0, 0.0, 0.0, 0.0, 0.0, 0.0, 0.0, 0.0, 0.0, 0.0, 0.0, 0.0, 0.0, 0.0, 0.0, 0.0, 0.0, 0.0, 0.0, 0.0, 0.0, 0.0, 0.0, 0.0, 0.0, 0.0, 0.0, 0.0, 0.0, 0.0, 0.0, 0.0, 0.0, 0.0, 0.0, 0.0, 0.0, 0.0, 0.0, 0.0, 0.0, 0.0, 0.0, 0.0, 0.0, 0.0, 0.0, 0.0, 0.0, 0.0, 0.0, 0.0, 0.0, 0.0, 0.0, 0.0, 0.0, 0.0, 0.0, 0.0, 0.0, 0.0, 0.0, 0.0, 0.0, 0.0, 0.0, 0.0, 0.0, 0.0, 0.0, 0.0, 0.0, 0.0, 0.0, 0.0, 0.0, 0.0, 0.0, 0.0, 0.0, 0.0, 0.0, 0.0, 0.0, 0.0, 0.0, 0.0, 0.0, 0.0, 0.0, 0.0, 0.0, 0.0, 0.0, 0.0, 0.0, 0.0, 0.0, 0.0, 0.0, 0.0, 0.0, 0.0, 0.0, 0.0, 0.0, 0.0, 0.0, 0.0, 0.0, 0.0, 0.0, 0.0, 0.0, 0.0, 0.0, 0.0, 0.0, 0.0, 0.0, 0.0, 0.0, 0.0, 0.0, 0.0, 0.0, 0.0, 0.0, 0.0, 0.0, 0.0, 0.0, 0.0, 0.0, 0.0, 0.0, 0.0, 0.0, 0.0, 0.0, 0.0, 0.0, 0.0, 0.0, 0.0, 0.0, 0.0, 0.0, 0.0, 0.0, 0.0, 0.0, 0.0, 0.0, 0.0, 0.0, 0.0, 0.0, 0.0, 0.0, 0.0, 0.0, 0.0, 0.0, 0.0, 0.0, 0.0, 0.0, 0.0, 0.0, 0.0, 0.0, 0.0, 0.0, 0.0, 0.0, 0.0, 0.0, 0.0, 0.0, 0.0, 0.0, 0.0, 0.0, 0.0, 0.0, 0.0, 0.0, 0.0, 0.0, 0.0, 0.0, 0.0, 0.0, 0.0, 0.0, 0.0, 0.0, 0.0, 0.0, 0.0, 0.0, 0.0, 0.0, 0.0, 0.0, 0.0, 0.0, 0.0, 0.0, 0.0, 0.0, 0.0, 0.0, 0.0, 0.0, 0.0, 0.0, 0.0, 0.0, 0.0, 0.0, 0.0, 0.0, 0.0, 0.0, 0.0, 0.0, 0.0, 0.0, 0.0, 0.0, 0.0, 0.0, 0.0, 0.0, 0.0, 0.0, 0.0, 0.0, 0.0, 0.0, 0.0, 0.0, 0.0, 0.0, 0.0, 0.0, 0.0, 0.0, 0.0, 0.0, 0.0, 0.0, 0.0, 0.0, 0.0, 0.0, 0.0, 0.0, 0.0, 0.0, 0.0, 0.0, 0.0, 0.0, 0.0, 0.0, 0.0, 0.0, 0.0, 0.0, 0.0, 0.0, 0.0, 0.0, 0.0, 0.0, 0.0, 0.0, 0.0, 0.0, 0.0, 0.0, 0.0, 0.0, 0.0, 0.0, 0.0, 0.0, 0.0, 0.0, 0.0, 0.0, 0.0, 0.0, 0.0, 0.0, 0.0, 0.0, 0.0, 0.0, 0.0, 0.0, 0.0, 0.0, 0.0, 0.0, 0.0, 0.0, 0.0, 0.0, 0.0, 0.0, 0.0, 0.0, 0.0, 0.0, 0.0, 0.0, 0.0, 0.0, 0.0, 0.0, 0.0, 0.0, 0.0, 0.0, 0.0, 0.0, 0.0, 0.0, 0.0, 0.0, 0.0, 0.0, 0.0, 0.0, 0.0, 0.0, 0.0, 0.0, 0.0, 0.0, 0.0, 0.0, 0.0, 0.0, 0.0, 0.0, 0.0, 0.0, 0.0, 0.0, 0.0, 0.0, 0.0, 0.0, 0.0, 0.0, 0.0, 0.0, 0.0, 0.0, 0.0, 0.0, 0.0, 0.0, 0.0, 0.0, 0.0, 0.0, 0.0, 0.0, 0.0, 0.0, 0.0, 0.0, 0.0, 0.0, 0.0, 0.0, 0.0, 0.0, 0.0, 0.0, 0.0, 0.0, 0.0, 0.0, 0.0, 0.0, 0.0, 0.0, 0.0, 0.0, 0.0, 0.0, 0.0, 0.0, 0.0, 0.0, 0.0, 0.0, 0.0, 0.0, 0.0, 0.0, 0.0, 0.0, 0.0, 0.0, 0.0, 0.0, 0.0, 0.0, 0.0, 0.0, 0.0, 0.0, 0.0, 0.0, 0.0, 0.0, 0.0, 0.0, 0.0, 0.0, 0.0, 0.0, 0.0, 0.0, 0.0, 0.0, 0.0, 0.0, 0.0, 0.0, 0.0, 0.0, 0.0, 0.0, 0.0, 0.0, 0.0, 0.0, 0.0, 0.0, 0.0, 0.0, 0.0, 0.0, 0.0, 0.0, 0.0, 0.0, 0.0, 0.0, 0.0, 0.0, 0.0, 0.0, 0.0, 0.0, 0.0, 0.0, 0.0, 0.0, 0.0, 0.0, 0.0, 0.0, 0.0, 0.0, 0.0, 0.0, 0.0, 0.0, 0.0, 0.0, 0.0, 0.0, 0.0, 0.0, 0.0, 0.0, 0.0, 0.0, 0.0, 0.0, 0.0, 0.0, 0.0, 0.0, 0.0, 0.0, 0.0, 0.0, 0.0, 0.0, 0.0, 0.0, 0.0, 0.0, 0.0, 0.0, 0.0, 0.0, 0.0, 0.0, 0.0, 0.0, 0.0, 0.0, 0.0, 0.0, 0.0, 0.0, 0.0, 0.0, 0.0, 0.0, 0.0, 0.0, 0.0, 0.0, 0.0, 0.0, 0.0, 0.0, 0.0, 0.0, 0.0, 0.0, 0.0, 0.0, 0.0, 0.0, 0.0, 0.0, 0.0, 0.0, 0.0, 0.0, 0.0, 0.0, 0.0, 0.0, 0.0, 0.0, 0.0, 0.0, 0.0, 0.0, 0.0, 0.0, 0.0, 0.0, 0.0, 0.0, 0.0, 0.0, 0.0, 0.0, 0.0, 0.0, 0.0, 0.0, 0.0, 0.0, 0.0, 0.0, 0.0, 0.0, 0.0, 0.0, 0.0, 0.0, 0.0, 0.0, 0.0, 0.0, 0.0, 0.0, 0.0, 0.0, 0.0, 0.0, 0.0, 0.0, 0.0, 0.0, 0.0, 0.0, 0.0, 0.0, 0.0, 0.0, 0.0, 0.0, 0.0, 0.0, 0.0, 0.0, 0.0, 0.0, 0.0, 0.0, 0.0, 0.0, 0.0, 0.0, 0.0, 0.0, 0.0, 0.0, 0.0, 0.0, 0.0, 0.0, 0.0, 0.0, 0.0, 0.0, 0.0, 0.0, 0.0, 0.0, 0.0, 0.0, 0.0, 0.0, 0.0, 0.0, 0.0, 0.0, 0.0, 0.0, 0.0, 0.0, 0.0, 0.0, 0.0, 0.0, 0.0, 0.0, 0.0, 0.0, 0.0, 0.0, 0.0, 0.0, 0.0, 0.0, 0.0, 0.0, 0.0, 0.0, 0.0, 0.0, 0.0, 0.0, 0.0, 0.0, 0.0, 0.0, 0.0, 0.0, 0.0, 0.0, 0.0, 0.0, 0.0, 0.0, 0.0, 0.0, 0.0, 0.0, 0.0, 0.0, 0.0, 0.0, 0.0, 0.0, 0.0, 0.0, 0.0, 0.0, 0.0, 0.0, 0.0, 0.0, 0.0, 0.0, 0.0, 0.0, 0.0, 0.0, 0.0, 0.0, 0.0, 0.0, 0.0, 0.0, 0.0, 0.0, 0.0, 0.0, 0.0, 0.0, 0.0, 0.0, 0.0, 0.0, 0.0, 0.0, 0.0, 0.0, 0.0, 0.0, 0.0, 0.0, 0.0, 0.0, 0.0, 0.0, 0.0, 0.0, 0.0, 0.0, 0.0, 0.0, 0.0, 0.0, 0.0, 0.0, 0.0, 0.0, 0.0, 0.0, 0.0, 0.0, 0.0, 0.0, 0.0, 0.0, 0.0, 0.0, 0.0, 0.0, 0.0, 0.0, 0.0, 0.0, 0.0, 0.0, 0.0, 0.0, 0.0, 0.0, 0.0, 0.0, 0.0, 0.0, 0.0, 0.0, 0.0, 0.0, 0.0, 0.0, 0.0, 0.0, 0.0, 0.0, 0.0, 0.0, 0.0, 0.0, 0.0, 0.0, 0.0, 0.0, 0.0, 0.0, 0.0, 0.0, 0.0, 0.0, 0.0, 0.0, 0.0, 0.0, 0.0, 0.0, 0.0, 0.0, 0.0, 0.0, 0.0, 0.0, 0.0, 0.0, 0.0, 0.0, 0.0, 0.0, 0.0, 0.0, 0.0, 0.0, 0.0, 0.0, 0.0, 0.0, 0.0, 0.0, 0.0, 0.0, 0.0, 0.0, 0.0, 0.0, 0.0, 0.0, 0.0, 0.0, 0.0, 0.0, 0.0, 0.0, 0.0, 0.0, 0.0, 0.0, 0.0, 0.0, 0.0, 0.0, 0.0, 0.0, 0.0, 0.0, 0.0, 0.0, 0.0, 0.0, 0.0, 0.0, 0.0, 0.0, 0.0, 0.0, 0.0, 0.0, 0.0, 0.0, 0.0, 0.0, 0.0, 0.0, 0.0, 0.0, 0.0, 0.0, 0.0, 0.0, 0.0, 0.0, 0.0, 0.0, 0.0, 0.0, 0.0, 0.0, 0.0, 0.0, 0.0, 0.0, 0.0, 0.0, 0.0, 0.0, 0.0, 0.0, 0.0, 0.0, 0.0, 0.0, 0.0, 0.0, 0.0, 0.0, 0.0, 0.0, 0.0, 0.0, 0.0, 0.0, 0.0, 0.0, 0.0, 0.0, 0.0, 0.0, 0.0, 0.0, 0.0, 0.0, 0.0, 0.0, 0.0, 0.0, 0.0, 0.0, 0.0, 0.0, 0.0, 0.0, 0.0, 0.0, 0.0, 0.0, 0.0, 0.0, 0.0, 0.0, 0.0, 0.0, 0.0, 0.0, 0.0, 0.0, 0.0, 0.0, 0.0, 0.0, 0.0, 0.0, 0.0, 0.0, 0.0, 0.0, 0.0, 0.0, 0.0, 0.0, 0.0, 0.0, 0.0, 0.0, 0.0, 0.0, 0.0, 0.0, 0.0, 0.0]]
  out "X":dbl[][](graph)=[[-0.026292607596389385, -0.023070532177615996, -0.024037154801081463, -0.023392739718564877, -0.02435936234264921, -0.023392739718564877, -0.023714947259720027, -0.023070532177615996, -0.02435936234264921, -0.023392739718564877, -0.02435936234264921, -0.023070532177615996, -0.024681569884423285, -0.023392739718564877, -0.02435936234264921, -0.023070532177615996, -0.02532598496859052, -0.023392739718564877, -0.024037154801081463, -0.023070532177615996, -0.024681569884423285, -0.023392739718564877, -0.02435936234264921, -0.023392739718564877, -0.025648192510983717, -0.024037154801081463, -0.023714947259720027, -0.02242611709633695, -0.024681569884423285, -0.023714947259720027, -0.02435936234264921, -0.02274832463687336, -0.02532598496859052, -0.023070532177615996, -0.024037154801081463, -0.023070532177615996, -0.025003777426403716, -0.02274832463687336, -0.025003777426403716, -0.021781702015882715, -0.025003777426403716, -0.023070532177615996, -0.023714947259720027, -0.023070532177615996, -0.025003777426403716, -0.023070532177615996, -0.02435936234264921, -0.02274832463687336, -0.02532598496859052, -0.023070532177615996, -0.02532598496859052, -0.023070532177615996, -0.024681569884423285, -0.023392739718564877, -0.023714947259720027, -0.023070532177615996, -0.025003777426403716, -0.02242611709633695, -0.024681569884423285, -0.023392739718564877, -0.024681569884423285, -0.02435936234264921, -0.023714947259720027, -0.023392739718564877, -0.02532598496859052, -0.02274832463687336, -0.025003777426403716, -0.023392739718564877, -0.02435936234264921, -0.023392739718564877, -0.02435936234264921, -0.02274832463687336, -0.024681569884423285, -0.02274832463687336, -0.024037154801081463, -0.023714947259720027, -0.02435936234264921, -0.02274832463687336, -0.025003777426403716, -0.02274832463687336, -0.025003777426403716, -0.02274832463687336, -0.024681569884423285, -0.023714947259720027, -0.02435936234264921, -0.023070532177615996, -0.025003777426403716, -0.022103909556006742, -0.024681569884423285, -0.023070532177615996, -0.024681569884423285, -0.024037154801081463, -0.02435936234264921, -0.023392739718564877, -0.024037154801081463, -0.023714947259720027, -0.02435936234264921, -0.023392739718564877, -0.02435936234264921, -0.02274832463687336, -0.02435936234264921, -0.023714947259720027, -0.023714947259720027, -0.023714947259720027, -0.024681569884423285, -0.023392739718564877, -0.023714947259720027, -0.023392739718564877, -0.025003777426403716, -0.02274832463687336, -0.024037154801081463, -0.023714947259720027, -0.02435936234264921, -0.02274832463687336, -0.02435936234264921, -0.023392739718564877, -0.02435936234264921, -0.023070532177615996, -0.024037154801081463, -0.023714947259720027, -0.02435936234264921, -0.023070532177615996, -0.024681569884423285, -0.024037154801081463, -0.024681569884423285, -0.023392739718564877, -0.024681569884423285, -0.02435936234264921, -0.025003777426403716, -0.023070532177615996, -0.024037154801081463, -0.02435936234264921, -0.024037154801081463, -0.02242611709633695, -0.02435936234264921, -0.02274832463687336, -0.02435936234264921, -0.023392739718564877, -0.024681569884423285, -0.023392739718564877, -0.024681569884423285, -0.021781702015882715, -0.023392739718564877, -0.023714947259720027, -0.023392739718564877, -0.022103909556006742, -0.023714947259720027, -0.023070532177615996, -0.023392739718564877, -0.02242611709633695, -0.023392739718564877, -0.023392739718564877, -0.024681569884423285, -0.02274832463687336, -0.02532598496859052, -0.023392739718564877, -0.024037154801081463, -0.02274832463687336, -0.024037154801081463, -0.023714947259720027, -0.024037154801081463, -0.023392739718564877, -0.024681569884423285, -0.023392739718564877, -0.02435936234264921, -0.023070532177615996, -0.02532598496859052, -0.023392739718564877, -0.023714947259720027, -0.023392739718564877, -0.024681569884423285, -0.023070532177615996, -0.02435936234264921, -0.023070532177615996, -0.02532598496859052, -0.023392739718564877, -0.024681569884423285, -0.02242611709633695, -0.024681569884423285, -0.023714947259720027, -0.023714947259720027, -0.02274832463687336, -0.025003777426403716, -0.023070532177615996, -0.024037154801081463, -0.02274832463687336, -0.02435936234264921, -0.024037154801081463, -0.023714947259720027, -0.023392739718564877, -0.024681569884423285, -0.023070532177615996, -0.024037154801081463, -0.023070532177615996, -0.025003777426403716, -0.024037154801081463, -0.024681569884423285, -0.023070532177615996, -0.024681569884423285, -0.023714947259720027, -0.02435936234264921, -0.02242611709633695, -0.025003777426403716, -0.023392739718564877, -0.02435936234264921, -0.023392739718564877, -0.02532598496859052, -0.02274832463687336, -0.02435936234264921, -0.023392739718564877, -0.02435936234264921, -0.023392739718564877, -0.024681569884423285, -0.023714947259720027, -0.02435936234264921, -0.02274832463687336, -0.02435936234264921, -0.02274832463687336, -0.024681569884423285, -0.023070532177615996, -0.023714947259720027, -0.023392739718564877, -0.025003777426403716, -0.023070532177615996, -0.024681569884423285, -0.02274832463687336, -0.025003777426403716, -0.023392739718564877, -0.02435936234264921, -0.023392739718564877, -0.024681569884423285, -0.023070532177615996, -0.02435936234264921, -0.023070532177615996, -0.025003777426403716, -0.023070532177615996, -0.023392739718564877, -0.023070532177615996, -0.024681569884423285, -0.023070532177615996, -0.025003777426403716, -0.02242611709633695, -0.024681569884423285, -0.02274832463687336, -0.024037154801081463, -0.023392739718564877, -0.024681569884423285, -0.02274832463687336, -0.025003777426403716, -0.023070532177615996, -0.02435936234264921, -0.023070532177615996, -0.024037154801081463, -0.02274832463687336, -0.02435936234264921, -0.023392739718564877, -0.02435936234264921, -0.023714947259720027, -0.02435936234264921, -0.023070532177615996, -0.024037154801081463, -0.023714947259720027, -0.024037154801081463, -0.023392739718564877, -0.024037154801081463, -0.023392739718564877, -0.024681569884423285, -0.023070532177615996, -0.024681569884423285, -0.023392739718564877, -0.025003777426403716, -0.02242611709633695, -0.025003777426403716, -0.023070532177615996, -0.02435936234264921, -0.023392739718564877, -0.024037154801081463, -0.023392739718564877, -0.024681569884423285, -0.023070532177615996, -0.02435936234264921, -0.023392739718564877, -0.02435936234264921, -0.023392739718564877, -0.024681569884423285, -0.024037154801081463, -0.025003777426403716, -0.023392739718564877, -0.023392739718564877, -0.024037154801081463, -0.02435936234264921, -0.023070532177615996, -0.02435936234264921, -0.023392739718564877, -0.024037154801081463, -0.02274832463687336, -0.02435936234264921, -0.023392739718564877, -0.024037154801081463, -0.02242611709633695, -0.024037154801081463, -0.023714947259720027, -0.024681569884423285, -0.02242611709633695, -0.025003777426403716, -0.023392739718564877, -0.02435936234264921, -0.023070532177615996, -0.024681569884423285, -0.023392739718564877, -0.02532598496859052, -0.02242611709633695, -0.02435936234264921, -0.023714947259720027, -0.023714947259720027, -0.023392739718564877, -0.024681569884423285, -0.023714947259720027, -0.024037154801081463, -0.023070532177615996, -0.024037154801081463, -0.023714947259720027, -0.02435936234264921, -0.023070532177615996, -0.024037154801081463, -0.02274832463687336, -0.023392739718564877, -0.023070532177615996, -0.02435936234264921, -0.023714947259720027, -0.024037154801081463, -0.02274832463687336, -0.024681569884423285, -0.023714947259720027, -0.023714947259720027, -0.023070532177615996, -0.025003777426403716, -0.023070532177615996, -0.024037154801081463, -0.02242611709633695, -0.02532598496859052, -0.023392739718564877, -0.02435936234264921, -0.023392739718564877, -0.024037154801081463, -0.024037154801081463, -0.023714947259720027, -0.023070532177615996, -0.024681569884423285, -0.023714947259720027, -0.023714947259720027, -0.023070532177615996, -0.025003777426403716, -0.023714947259720027, -0.023070532177615996, -0.023714947259720027, -0.024681569884423285, -0.023714947259720027, -0.02435936234264921, -0.02274832463687336, -0.024681569884423285, -0.023392739718564877, -0.024037154801081463, -0.023392739718564877, -0.02435936234264921, -0.023070532177615996, -0.02532598496859052, -0.02274832463687336, -0.025003777426403716, -0.02274832463687336, -0.023714947259720027, -0.023070532177615996, -0.02532598496859052, -0.023392739718564877, -0.024037154801081463, -0.023392739718564877, -0.025003777426403716, -0.023392739718564877, -0.023714947259720027, -0.023070532177615996, -0.02532598496859052, -0.023392739718564877, -0.024037154801081463, -0.023070532177615996, -0.024681569884423285, -0.023714947259720027, -0.02435936234264921, -0.02274832463687336, -0.024681569884423285, -0.02242611709633695, -0.02435936234264921, -0.023070532177615996, -0.024681569884423285, -0.023070532177615996, -0.024681569884423285, -0.02274832463687336, -0.02435936234264921, -0.023070532177615996, -0.02435936234264921, -0.023070532177615996, -0.025003777426403716, -0.02274832463687336, -0.024037154801081463, -0.023070532177615996, -0.024681569884423285, -0.023392739718564877, -0.024681569884423285, -0.023070532177615996, -0.025003777426403716, -0.023714947259720027, -0.023714947259720027, -0.024037154801081463, -0.025003777426403716, -0.02242611709633695, -0.023714947259720027, -0.023070532177615996, -0.024037154801081463, -0.023070532177615996, -0.024037154801081463, -0.023070532177615996, -0.024681569884423285, -0.023392739718564877, -0.023714947259720027, -0.023392739718564877, -0.02532598496859052, -0.023392739718564877, -0.02532598496859052, -0.023714947259720027, -0.024681569884423285, -0.023070532177615996, -0.02435936234264921, -0.023070532177615996, -0.02532598496859052, -0.022103909556006742, -0.023714947259720027, -0.023392739718564877, -0.024681569884423285, -0.022103909556006742, -0.024681569884423285, -0.023714947259720027, -0.023714947259720027, -0.023392739718564877, -0.02435936234264921, -0.023070532177615996, -0.02435936234264921, -0.023070532177615996, -0.023392739718564877, -0.024681569884423285, -0.02435936234264921, -0.023070532177615996, -0.02435936234264921, -0.023070532177615996, -0.02435936234264921, -0.023392739718564877, -0.02435936234264921, -0.023070532177615996, -0.024681569884423285, -0.022103909556006742, -0.024037154801081463, -0.02435936234264921, -0.024681569884423285, -0.02274832463687336, -0.025003777426403716, -0.02274832463687336, -0.024681569884423285, -0.02274832463687336, -0.024037154801081463, -0.024037154801081463, -0.02435936234264921, -0.023070532177615996, -0.023392739718564877, -0.023714947259720027, -0.02435936234264921, -0.023392739718564877, -0.024037154801081463, -0.023714947259720027, -0.024681569884423285, -0.023392739718564877, -0.023392739718564877, -0.024681569884423285, -0.024037154801081463, -0.02242611709633695, -0.02435936234264921, -0.023070532177615996, -0.023392739718564877, -0.023714947259720027, -0.024037154801081463, -0.023392739718564877, -0.025003777426403716, -0.02274832463687336, -0.024681569884423285, -0.023714947259720027, -0.024037154801081463, -0.02274832463687336, -0.025003777426403716, -0.02274832463687336, -0.025003777426403716, -0.02274832463687336, -0.024681569884423285, -0.023714947259720027, -0.024037154801081463, -0.022103909556006742, -0.024681569884423285, -0.023714947259720027, -0.02435936234264921, -0.023070532177615996, -0.024037154801081463, -0.024681569884423285, -0.023714947259720027, -0.023392739718564877, -0.02532598496859052, -0.023070532177615996, -0.024037154801081463, -0.023070532177615996, -0.024037154801081463, -0.023392739718564877, -0.02435936234264921, -0.023070532177615996, -0.025003777426403716, -0.02242611709633695, -0.025970400053583333, -0.02242611709633695, -0.02532598496859052, -0.024037154801081463, -0.02435936234264921, -0.023070532177615996, -0.025003777426403716, -0.023070532177615996, -0.024037154801081463, -0.02274832463687336, -0.02435936234264921, -0.023392739718564877, -0.02435936234264921, -0.023070532177615996, -0.02435936234264921, -0.023392739718564877, -0.024681569884423285, -0.023070532177615996, -0.025003777426403716, -0.023070532177615996, -0.02435936234264921, -0.02274832463687336, -0.02435936234264921, -0.023714947259720027, -0.023714947259720027, -0.023392739718564877, -0.024681569884423285, -0.023392739718564877, -0.023392739718564877, -0.023070532177615996, -0.025003777426403716, -0.02274832463687336, -0.024681569884423285, -0.02274832463687336, -0.025003777426403716, -0.023070532177615996, -0.024681569884423285, -0.02274832463687336, -0.02532598496859052, -0.02274832463687336, -0.02435936234264921, -0.02274832463687336, -0.02532598496859052, -0.021781702015882715, -0.024037154801081463, -0.02274832463687336, -0.02435936234264921, -0.023392739718564877, -0.024037154801081463, -0.023070532177615996, -0.024681569884423285, -0.023392739718564877, -0.02435936234264921, -0.023714947259720027, -0.024037154801081463, -0.023714947259720027, -0.024037154801081463, -0.023714947259720027, -0.024037154801081463, -0.023070532177615996, -0.023714947259720027, -0.024037154801081463, -0.024681569884423285, -0.023070532177615996, -0.02435936234264921, -0.023392739718564877, -0.02532598496859052, -0.023392739718564877, -0.025003777426403716, -0.023070532177615996, -0.024681569884423285, -0.02242611709633695, -0.02532598496859052, -0.023392739718564877, -0.024681569884423285, -0.02242611709633695, -0.024681569884423285, -0.02242611709633695, -0.024681569884423285, -0.023392739718564877, -0.024037154801081463, -0.023392739718564877, -0.024681569884423285, -0.02274832463687336, -0.023070532177615996, -0.023714947259720027, -0.02435936234264921, -0.023070532177615996, -0.024681569884423285, -0.024037154801081463, -0.025003777426403716, -0.023070532177615996, -0.02435936234264921, -0.024037154801081463, -0.02435936234264921, -0.023392739718564877, -0.02435936234264921, -0.023714947259720027, -0.024681569884423285, -0.023714947259720027, -0.024037154801081463, -0.023714947259720027, -0.025003777426403716, -0.02242611709633695, -0.02435936234264921, -0.023714947259720027, -0.02435936234264921, -0.02242611709633695, -0.02435936234264921, -0.024037154801081463, -0.023392739718564877, -0.023070532177615996, -0.024681569884423285, -0.023392739718564877, -0.024681569884423285, -0.023070532177615996, -0.02435936234264921, -0.024037154801081463, -0.024681569884423285, -0.02274832463687336, -0.02435936234264921, -0.023714947259720027, -0.023392739718564877, -0.023070532177615996, -0.024037154801081463, -0.023392739718564877, -0.02435936234264921, -0.023070532177615996, -0.02435936234264921, -0.02435936234264921, -0.023392739718564877, -0.023070532177615996, -0.024681569884423285, -0.023392739718564877, -0.024681569884423285, -0.023070532177615996, -0.023392739718564877, -0.023070532177615996, -0.024037154801081463, -0.022103909556006742, -0.02532598496859052, -0.02274832463687336, -0.023714947259720027, -0.023070532177615996, -0.02435936234264921, -0.023070532177615996, -0.024037154801081463, -0.02274832463687336, -0.025003777426403716, -0.023714947259720027, -0.02435936234264921, -0.023392739718564877, -0.02435936234264921, -0.023392739718564877, -0.023392739718564877, -0.023070532177615996, -0.024681569884423285, -0.023392739718564877, -0.02435936234264921, -0.02274832463687336, -0.024037154801081463, -0.023714947259720027, -0.02274832463687336, -0.023070532177615996, -0.024681569884423285, -0.023070532177615996, -0.025003777426403716, -0.02274832463687336, -0.024681569884423285, -0.023070532177615996, -0.024037154801081463, -0.023070532177615996, -0.024681569884423285, -0.02274832463687336, -0.02435936234264921, -0.02274832463687336, -0.02532598496859052, -0.023714947259720027, -0.02435936234264921, -0.02242611709633695, -0.02435936234264921, -0.023070532177615996, -0.023714947259720027, -0.02274832463687336, -0.024681569884423285, -0.023392739718564877, -0.023392739718564877, -0.023392739718564877, -0.024681569884423285, -0.02274832463687336, -0.024037154801081463, -0.02274832463687336, -0.02435936234264921, -0.023392739718564877, -0.02435936234264921, -0.02274832463687336, -0.025648192510983717, -0.02242611709633695, -0.02435936234264921, -0.02435936234264921, -0.025003777426403716, -0.02274832463687336, -0.02532598496859052, -0.02242611709633695, -0.02532598496859052, -0.023070532177615996, -0.02435936234264921, -0.023070532177615996, -0.024681569884423285, -0.023070532177615996, -0.025003777426403716, -0.023392739718564877, -0.024681569884423285, -0.023070532177615996, -0.025003777426403716, -0.023070532177615996, -0.024681569884423285, -0.023070532177615996, -0.024037154801081463, -0.023070532177615996, -0.02435936234264921, -0.023070532177615996, -0.02435936234264921, -0.023070532177615996, -0.02435936234264921, -0.022103909556006742, -0.024681569884423285, -0.02274832463687336, -0.024681569884423285, -0.022103909556006742, -0.024037154801081463, -0.023070532177615996, -0.024681569884423285, -0.02274832463687336, -0.024037154801081463, -0.023392739718564877, -0.02435936234264921, -0.023070532177615996, -0.024037154801081463, -0.023392739718564877, -0.02532598496859052, -0.02242611709633695, -0.02435936234264921, -0.023714947259720027, -0.02435936234264921, -0.023392739718564877, -0.024037154801081463, -0.02242611709633695, -0.024037154801081463, -0.02274832463687336, -0.02435936234264921, -0.023392739718564877, -0.025003777426403716, -0.02274832463687336, -0.02435936234264921, -0.024037154801081463, -0.02435936234264921, -0.023070532177615996, -0.024037154801081463, -0.023070532177615996, -0.02435936234264921, -0.02242611709633695, -0.024037154801081463, -0.023392739718564877, -0.025003777426403716, -0.02274832463687336, -0.02532598496859052, -0.023392739718564877, -0.025003777426403716, -0.023070532177615996, -0.023392739718564877, -0.023392739718564877, -0.02435936234264921, -0.023070532177615996, -0.023714947259720027, -0.023714947259720027, -0.024037154801081463, -0.02274832463687336, -0.023714947259720027, -0.023392739718564877, -0.02435936234264921, -0.023392739718564877, -0.024037154801081463, -0.02435936234264921, -0.024037154801081463, -0.023714947259720027, -0.024681569884423285, -0.02435936234264921, -0.02435936234264921, -0.023392739718564877, -0.024037154801081463, -0.023070532177615996, -0.024681569884423285, -0.02242611709633695, -0.02435936234264921, -0.023392739718564877, -0.023714947259720027, -0.023070532177615996, -0.02435936234264921, -0.023392739718564877, -0.023714947259720027, -0.02274832463687336, -0.023714947259720027, -0.023714947259720027, -0.024681569884423285, -0.02274832463687336, -0.02435936234264921, -0.023714947259720027, -0.02435936234264921, -0.02274832463687336, -0.024037154801081463, -0.02435936234264921, -0.02435936234264921, -0.023392739718564877, -0.02435936234264921, -0.024037154801081463, -0.024037154801081463, -0.023714947259720027, -0.025648192510983717, -0.023714947259720027, -0.023714947259720027, -0.023392739718564877, -0.024037154801081463, -0.023070532177615996, -0.023714947259720027, -0.023070532177615996, -0.024037154801081463, -0.023392739718564877, -0.024681569884423285, -0.02242611709633695, -0.025003777426403716, -0.023070532177615996, -0.024037154801081463, -0.023070532177615996, -0.024037154801081463, -0.023392739718564877, -0.025003777426403716, -0.022103909556006742, -0.024681569884423285, -0.023392739718564877, -0.023392739718564877, -0.023070532177615996, -0.025003777426403716, -0.023714947259720027, -0.024037154801081463, -0.023070532177615996, -0.02435936234264921, -0.02274832463687336, -0.023392739718564877, -0.02242611709633695, -0.024681569884423285, -0.023070532177615996, -0.02435936234264921, -0.02274832463687336, -0.025003777426403716, -0.024037154801081463, -0.024037154801081463, -0.023070532177615996, -0.025003777426403716, -0.022103909556006742, -0.025003777426403716, -0.02274832463687336, -0.025003777426403716, -0.023392739718564877, -0.025003777426403716, -0.023392739718564877, -0.02435936234264921, -0.02274832463687336, -0.024037154801081463, -0.023070532177615996, -0.025003777426403716, -0.023392739718564877, -0.023714947259720027, -0.023070532177615996, -0.025003777426403716, -0.02274832463687336, -0.023714947259720027, -0.023714947259720027, -0.02435936234264921, -0.023070532177615996, -0.025003777426403716, -0.023070532177615996, -0.025003777426403716, -0.02274832463687336, -0.024681569884423285, -0.023070532177615996, -0.025003777426403716, -0.023070532177615996, -0.024037154801081463, -0.022103909556006742, -0.025003777426403716, -0.02242611709633695, -0.02532598496859052, -0.023070532177615996, -0.025003777426403716, -0.023070532177615996, -0.023714947259720027, -0.023070532177615996, -0.024681569884423285, -0.023070532177615996, -0.023714947259720027, -0.023070532177615996, -0.024681569884423285, -0.023392739718564877, -0.025003777426403716, -0.02274832463687336, -0.024681569884423285, -0.024037154801081463, -0.023392739718564877, -0.023714947259720027, -0.02532598496859052, -0.022103909556006742, -0.025003777426403716, -0.023392739718564877, -0.02435936234264921, -0.023070532177615996, -0.02435936234264921, -0.023392739718564877, -0.024681569884423285, -0.023714947259720027, -0.02435936234264921, -0.023070532177615996, -0.025003777426403716, -0.02274832463687336, -0.024037154801081463, -0.023070532177615996, -0.024681569884423285, -0.02274832463687336, -0.02435936234264921, -0.023714947259720027, -0.024681569884423285, -0.023070532177615996, -0.02435936234264921, -0.023392739718564877, -0.024037154801081463, -0.02242611709633695, -0.024681569884423285, -0.02274832463687336, -0.024037154801081463, -0.02274832463687336, -0.024037154801081463, -0.023070532177615996, -0.02435936234264921, -0.023070532177615996, -0.02435936234264921, -0.023714947259720027, -0.02435936234264921, -0.023070532177615996, -0.02435936234264921, -0.023714947259720027, -0.024681569884423285, -0.023070532177615996, -0.02532598496859052, -0.024037154801081463, -0.025003777426403716, -0.023392739718564877, -0.023714947259720027, -0.023392739718564877, -0.02435936234264921, -0.02242611709633695, -0.024681569884423285, -0.023392739718564877, -0.02435936234264921, -0.02274832463687336, -0.02435936234264921, -0.023392739718564877, -0.02435936234264921, -0.02274832463687336, -0.02435936234264921, -0.024037154801081463, -0.024681569884423285, -0.023070532177615996, -0.024681569884423285, -0.024037154801081463, -0.024037154801081463, -0.023070532177615996, -0.02435936234264921, -0.024037154801081463, -0.02532598496859052, -0.023070532177615996, -0.02435936234264921, -0.023392739718564877, -0.02435936234264921, -0.023392739718564877, -0.025003777426403716, -0.023392739718564877, -0.02435936234264921, -0.02274832463687336, -0.024681569884423285, -0.023070532177615996, -0.024681569884423285, -0.023070532177615996, -0.024681569884423285, -0.023714947259720027, -0.02435936234264921, -0.023070532177615996, -0.023714947259720027, -0.023714947259720027, -0.024037154801081463, -0.023070532177615996, -0.024681569884423285, -0.02274832463687336, -0.023714947259720027, -0.023392739718564877, -0.023714947259720027, -0.023070532177615996, -0.024037154801081463, -0.023070532177615996, -0.023714947259720027, -0.023392739718564877, -0.023714947259720027, -0.023714947259720027, -0.02435936234264921, -0.023392739718564877, -0.024037154801081463, -0.023070532177615996, -0.025003777426403716, -0.023392739718564877, -0.024681569884423285, -0.023070532177615996, -0.02532598496859052, -0.023714947259720027, -0.023392739718564877, -0.023714947259720027, -0.025003777426403716, -0.023070532177615996, -0.024037154801081463, -0.02274832463687336, -0.024681569884423285, -0.023070532177615996, -0.02435936234264921, -0.022103909556006742, -0.025003777426403716, -0.023714947259720027, -0.023070532177615996, -0.023392739718564877, -0.024681569884423285, -0.023714947259720027, -0.023714947259720027, -0.023070532177615996, -0.025003777426403716, -0.023392739718564877, -0.024037154801081463, -0.02274832463687336, -0.025003777426403716, -0.023392739718564877, -0.024681569884423285, -0.023392739718564877, -0.025970400053583333, -0.02242611709633695, -0.024681569884423285, -0.022103909556006742, -0.02532598496859052, -0.023392739718564877, -0.024037154801081463, -0.023070532177615996, -0.025003777426403716, -0.02242611709633695, -0.02435936234264921, -0.02274832463687336, -0.02435936234264921, -0.023714947259720027, -0.024037154801081463, -0.02274832463687336, -0.02532598496859052, -0.023392739718564877, -0.02435936234264921, -0.023714947259720027, -0.024037154801081463, -0.023392739718564877, -0.023392739718564877, -0.023392739718564877, -0.02435936234264921, -0.023070532177615996, -0.024037154801081463, -0.023392739718564877, -0.024681569884423285, -0.02242611709633695, -0.02435936234264921, -0.023392739718564877, -0.024681569884423285, -0.02274832463687336, -0.024681569884423285, -0.02242611709633695, -0.02532598496859052, -0.023714947259720027, -0.023392739718564877, -0.023392739718564877, -0.025003777426403716, -0.02274832463687336, -0.024681569884423285, -0.023392739718564877, -0.024681569884423285, -0.023070532177615996, -0.023714947259720027, -0.024037154801081463, -0.025003777426403716, -0.022103909556006742, -0.024037154801081463, -0.024037154801081463, -0.024037154801081463, -0.023392739718564877, -0.024037154801081463, -0.023392739718564877, -0.024681569884423285, -0.02242611709633695, -0.024681569884423285, -0.023392739718564877, -0.024037154801081463, -0.023070532177615996, -0.02435936234264921, -0.023070532177615996, -0.025003777426403716, -0.023070532177615996, -0.024681569884423285, -0.023714947259720027, -0.02435936234264921, -0.02274832463687336, -0.023392739718564877, -0.023392739718564877, -0.02435936234264921, -0.023070532177615996, -0.023714947259720027, -0.02435936234264921, -0.024037154801081463, -0.023392739718564877, -0.023714947259720027, -0.023714947259720027, -0.02435936234264921, -0.023070532177615996, -0.023714947259720027, -0.024037154801081463, -0.02435936234264921, -0.02274832463687336, -0.024037154801081463, -0.023714947259720027, -0.025003777426403716, -0.023070532177615996, -0.025003777426403716, -0.023714947259720027, -0.02435936234264921, -0.023070532177615996, -0.02435936234264921, -0.024037154801081463, -0.02435936234264921, -0.022103909556006742, -0.024681569884423285, -0.023392739718564877, -0.02435936234264921, -0.023714947259720027, -0.024037154801081463, -0.023070532177615996, -0.024037154801081463, -0.02274832463687336, -0.024681569884423285, -0.024037154801081463, -0.025003777426403716, -0.023070532177615996, -0.02435936234264921, -0.023070532177615996, -0.024037154801081463, -0.023070532177615996, -0.024037154801081463, -0.023392739718564877, -0.023392739718564877, -0.02274832463687336, -0.024037154801081463, -0.023070532177615996, -0.024681569884423285, -0.023070532177615996, -0.02435936234264921, -0.023392739718564877, -0.02435936234264921, -0.02274832463687336, -0.024681569884423285, -0.02274832463687336, -0.024037154801081463, -0.02274832463687336, -0.024681569884423285, -0.023392739718564877, -0.02435936234264921, -0.02242611709633695, -0.02435936234264921, -0.023070532177615996, -0.02435936234264921, -0.023392739718564877, -0.025003777426403716, -0.023392739718564877, -0.023714947259720027, -0.023392739718564877, -0.023714947259720027, -0.023714947259720027, -0.02435936234264921, -0.023070532177615996, -0.025003777426403716, -0.023392739718564877, -0.024037154801081463, -0.023070532177615996, -0.025003777426403716, -0.023392739718564877, -0.024037154801081463, -0.023070532177615996, -0.025003777426403716, -0.023392739718564877, -0.024037154801081463, -0.02242611709633695, -0.02435936234264921, -0.02435936234264921, -0.025003777426403716, -0.022103909556006742, -0.025648192510983717, -0.023070532177615996, -0.02435936234264921, -0.023070532177615996, -0.025003777426403716, -0.023392739718564877, -0.025648192510983717, -0.023070532177615996, -0.025003777426403716, -0.023070532177615996, -0.02532598496859052, -0.02274832463687336, -0.024681569884423285], [2.6768613724892623, 3.3942120501732074, 4.041293404695572, 4.624988788830939, 5.151507284658128, 5.626449752909397, 6.054868412341723, 6.441320582907965, 6.78991716442299, 7.104366366418435, 7.388013154364089, 7.6438748318666185, 7.8746731373526355, 8.0828631966658, 8.27065963956232, 8.440060157920097, 8.592866756262833, 8.730704920652407, 8.855040909859317, 8.967197352746703, 9.068367317785691, 9.159627004367115, 9.241947190913885, 9.316203561573767, 9.38318602134316, 9.443607098711844, 9.498109525212168, 9.547273072500436, 9.59162071970017, 9.631624216612632, 9.667709101973475, 9.700259230137382, 9.729620854343525, 9.756106309997696, 9.77999733715219, 9.801548077526444, 9.820987777949332, 9.838523228981126, 9.854340964656025, 9.868609246745109, 9.881479854647399, 9.89308969994904, 9.903562282825575, 9.913009005779784, 9.921530358690113, 9.929216987775597, 9.936150659848517, 9.94240513211199, 9.948046936755066, 9.953136088691437, 9.95772672397039, 9.961867675651114, 9.965602993266238, 9.968972411400435, 9.972011772368583, 9.974753407489779, 9.977226481012979, 9.97945730035282, 9.981469595935755, 9.983284773633375, 9.984922142468193, 9.98639912001411, 9.987731417676525, 9.98893320782302, 9.990017274542463, 9.990995149636237, 9.99187723528823, 9.992672914718463, 9.993390651997451, 9.99403808208308, 9.994622092037764, 9.995148894289839, 9.995624092718506, 9.99605274226531, 9.996439402706276, 9.996788187156705, 9.997102805824591, 9.997386605478104, 9.997642605046963, 9.99787352773642, 9.998081829995456, 9.99826972764736, 9.998439219460622, 9.99859210841092, 9.998730020860334, 9.99885442385785, 9.998966640745131, 9.99906786523363, 9.999159174102731, 9.999241538654038, 9.999315835043634, 9.999382853602214, 9.999443307242272, 9.999497839041727, 9.999547029084692, 10.0, 10.0, 10.0, 10.0, 10.0, 10.0, 10.0, 10.0, 10.0, 10.0, 10.0, 10.0, 10.0, 10.0, 10.0, 10.0, 10.0, 10.0, 10.0, 10.0, 10.0, 10.0, 10.0, 10.0, 10.0, 10.0, 8.905679619058906, 7.918746600615565, 7.028681630318472, 6.225995831400689, 5.502129826388611, 4.849362686395167, 4.260729799442091, 3.729948784132363, 3.2513526605766856, 2.819829567677141, 2.4307683855083266, 2.080009684351947, 1.7638014786033587, 1.4787593148805112, 1.2218302697710426, 0.9902604742421666, 0.7815658192530053, 0.5935055309492128, 0.42405833434498974, 0.2714009519327494, 0.13388870849856516, 0.010038035826386293, -0.10148930881587881, -0.2019004782848436, -0.2922843766965466, -0.37362324268583114, -0.44680309800756546, -0.5126231726271101, -0.5718044065597878, -0.6249971188979974, -0.6727879256055523, -0.7157059796675375, -0.7542285999755214, -0.7887863488256073, -0.8197676120414052, -0.8475227304431537, -0.8723677266116586, -0.8945876665906404, -0.9144396922877284, -0.9321557568313847, -0.9479450919812223, -0.961996433838887, -0.9744800305355918, -0.9855494532531561, -0.995343229843352, -1.0039863184232516, -1.0115914366219996, -1.0182602606189237, -1.0240845067278006, -1.0291469070326675, -1.0335220894535455, -1.0372773716038066, -1.0404734768838728, -1.0431651804287212, -1.0454018917804877, -1.0472281804843706, -1.0486842501988785, -1.0498063663637947, -1.0506272419751856, -1.0511763855711533, -1.0514804151300439, -1.051563341220215, -1.0514468224133786, -1.0511503956784916, -1.0506916842070118, -1.050086584880276, -1.049349437373185, -1.048493176693047, -1.0475294707762144, -1.0464688446062054, -1.045320792173621, -1.0440938774688338, -1.042795825581766, -1.0414336048778292, -1.04001350112418, -1.0385411843548091, -1.0370217691857464, -1.0354598692219847, -1.0338596461348812, -1.0322248539320953, -1.0305588788909903, -1.0288647755802882, -1.027145299353163, -1.0254029356574141, -1.023639926474515, -1.021858294168776, -1.0200598630003217, -1.0182462785307302, -1.0164190251277558, -1.014579441755349, -1.0127287362169364, -1.010867998003476, -1.0089982098829604, -1.007120258354647, -1.00523494307923, -1.0033429853852605, -1.0, -0.998046875, -0.99609375, -0.994140625, -0.9921875, -0.990234375, -0.98828125, -0.986328125, -0.984375, -0.982421875, -0.98046875, -0.978515625, -0.9765625, -0.974609375, -0.97265625, -0.970703125, -0.96875, -0.966796875, -0.96484375, -0.962890625, -0.9609375, -0.958984375, -0.95703125, -0.955078125, -0.953125, -0.951171875, -0.94921875, -0.947265625, -0.9453125, -0.943359375, -0.94140625, -0.939453125, -0.9375, -0.935546875, -0.93359375, -0.931640625, -0.9296875, -0.927734375, -0.92578125, -0.923828125, -0.921875, -0.919921875, -0.91796875, -0.916015625, -0.9140625, -0.912109375, -0.91015625, -0.908203125, -0.90625, -0.904296875, -0.90234375, -0.900390625, -0.8984375, -0.896484375, -0.89453125, -0.892578125, -0.890625, -0.888671875, -0.88671875, -0.884765625, -0.8828125, -0.880859375, -0.87890625, -0.876953125, -0.875, -0.873046875, -0.87109375, -0.869140625, -0.8671875, -0.865234375, -0.86328125, -0.861328125, -0.859375, -0.857421875, -0.85546875, -0.853515625, -0.8515625, -0.849609375, -0.84765625, -0.845703125, -0.84375, -0.841796875, -0.83984375, -0.837890625, -0.8359375, -0.833984375, -0.83203125, -0.830078125, -0.828125, -0.826171875, -0.82421875, -0.822265625, -0.8203125, -0.818359375, -0.81640625, -0.814453125, -0.8125, -0.810546875, -0.80859375, -0.806640625, -0.8046875, -0.802734375, -0.80078125, -0.798828125, -0.796875, -0.794921875, -0.79296875, -0.791015625, -0.7890625, -0.787109375, -0.78515625, -0.783203125, -0.78125, -0.779296875, -0.77734375, -0.775390625, -0.7734375, -0.771484375, -0.76953125, -0.767578125, -0.765625, -0.763671875, -0.76171875, -0.759765625, -0.7578125, -0.755859375, -0.75390625, -0.751953125, -0.75, -0.748046875, -0.74609375, -0.744140625, -0.7421875, -0.740234375, -0.73828125, -0.736328125, -0.734375, -0.732421875, -0.73046875, -0.728515625, -0.7265625, -0.724609375, -0.72265625, -0.720703125, -0.71875, -0.716796875, -0.71484375, -0.712890625, -0.7109375, -0.708984375, -0.70703125, -0.705078125, -0.703125, -0.701171875, -0.69921875, -0.697265625, -0.6953125, -0.693359375, -0.69140625, -0.689453125, -0.6875, -0.685546875, -0.68359375, -0.681640625, -0.6796875, -0.677734375, -0.67578125, -0.673828125, -0.671875, -0.669921875, -0.66796875, -0.666015625, -0.6640625, -0.662109375, -0.66015625, -0.658203125, -0.65625, -0.654296875, -0.65234375, -0.650390625, -0.6484375, -0.646484375, -0.64453125, -0.642578125, -0.640625, -0.638671875, -0.63671875, -0.634765625, -0.6328125, -0.630859375, -0.62890625, -0.626953125, -0.625, -0.623046875, -0.62109375, -0.619140625, -0.6171875, -0.615234375, -0.61328125, -0.611328125, -0.609375, -0.607421875, -0.60546875, -0.603515625, -0.6015625, -0.599609375, -0.59765625, -0.595703125, -0.59375, -0.591796875, -0.58984375, -0.587890625, -0.5859375, -0.583984375, -0.58203125, -0.580078125, -0.578125, -0.576171875, -0.57421875, -0.572265625, -0.5703125, -0.568359375, -0.56640625, -0.564453125, -0.5625, -0.560546875, -0.55859375, -0.556640625, -0.5546875, -0.552734375, -0.55078125, -0.548828125, -0.546875, -0.544921875, -0.54296875, -0.541015625, -0.5390625, -0.537109375, -0.53515625, -0.533203125, -0.53125, -0.529296875, -0.52734375, -0.525390625, -0.5234375, -0.521484375, -0.51953125, -0.517578125, -0.515625, -0.513671875, -0.51171875, -0.509765625, -0.5078125, -0.505859375, -0.50390625, -0.501953125, -0.5, -0.498046875, -0.49609375, -0.494140625, -0.4921875, -0.490234375, -0.48828125, -0.486328125, -0.484375, -0.482421875, -0.48046875, -0.478515625, -0.4765625, -0.474609375, -0.47265625, -0.470703125, -0.46875, -0.466796875, -0.46484375, -0.462890625, -0.4609375, -0.458984375, -0.45703125, -0.455078125, -0.453125, -0.451171875, -0.44921875, -0.447265625, -0.4453125, -0.443359375, -0.44140625, -0.439453125, -0.4375, -0.435546875, -0.43359375, -0.431640625, -0.4296875, -0.427734375, -0.42578125, -0.423828125, -0.421875, -0.419921875, -0.41796875, -0.416015625, -0.4140625, -0.412109375, -0.41015625, -0.408203125, -0.40625, -0.404296875, -0.40234375, -0.400390625, -0.3984375, -0.396484375, -0.39453125, -0.392578125, -0.390625, -0.388671875, -0.38671875, -0.384765625, -0.3828125, -0.380859375, -0.37890625, -0.376953125, -0.375, -0.373046875, -0.37109375, -0.369140625, -0.3671875, -0.365234375, -0.36328125, -0.361328125, -0.359375, -0.357421875, -0.35546875, -0.353515625, -0.3515625, -0.349609375, -0.34765625, -0.345703125, -0.34375, -0.341796875, -0.33984375, -0.337890625, -0.3359375, -0.333984375, -0.33203125, -0.330078125, -0.328125, -0.326171875, -0.32421875, -0.322265625, -0.3203125, -0.318359375, -0.31640625, -0.314453125, -0.3125, -0.310546875, -0.30859375, -0.306640625, -0.3046875, -0.302734375, -0.30078125, -0.298828125, -0.296875, -0.294921875, -0.29296875, -0.291015625, -0.2890625, -0.287109375, -0.28515625, -0.283203125, -0.28125, -0.279296875, -0.27734375, -0.275390625, -0.2734375, -0.271484375, -0.26953125, -0.267578125, -0.265625, -0.263671875, -0.26171875, -0.259765625, -0.2578125, -0.255859375, -0.25390625, -0.251953125, -0.25, -0.248046875, -0.24609375, -0.244140625, -0.2421875, -0.240234375, -0.23828125, -0.236328125, -0.234375, -0.232421875, -0.23046875, -0.228515625, -0.2265625, -0.224609375, -0.22265625, -0.220703125, -0.21875, -0.216796875, -0.21484375, -0.212890625, -0.2109375, -0.208984375, -0.20703125, -0.205078125, -0.203125, -0.201171875, -0.19921875, -0.197265625, -0.1953125, -0.193359375, -0.19140625, -0.189453125, -0.1875, -0.185546875, -0.18359375, -0.181640625, -0.1796875, -0.177734375, -0.17578125, -0.173828125, -0.171875, -0.169921875, -0.16796875, -0.166015625, -0.1640625, -0.162109375, -0.16015625, -0.158203125, -0.15625, -0.154296875, -0.15234375, -0.150390625, -0.1484375, -0.146484375, -0.14453125, -0.142578125, -0.140625, -0.138671875, -0.13671875, -0.134765625, -0.1328125, -0.130859375, -0.12890625, -0.126953125, -0.125, -0.123046875, -0.12109375, -0.119140625, -0.1171875, -0.115234375, -0.11328125, -0.111328125, -0.109375, -0.107421875, -0.10546875, -0.103515625, -0.1015625, -0.099609375, -0.09765625, -0.095703125, -0.09375, -0.091796875, -0.08984375, -0.087890625, -0.0859375, -0.083984375, -0.08203125, -0.080078125, -0.078125, -0.076171875, -0.07421875, -0.072265625, -0.0703125, -0.068359375, -0.06640625, -0.064453125, -0.0625, -0.060546875, -0.05859375, -0.056640625, -0.0546875, -0.052734375, -0.05078125, -0.048828125, -0.046875, -0.044921875, -0.04296875, -0.041015625, -0.0390625, -0.037109375, -0.03515625, -0.033203125, -0.03125, -0.029296875, -0.02734375, -0.025390625, -0.0234375, -0.021484375, -0.01953125, -0.017578125, -0.015625, -0.013671875, -0.01171875, -0.009765625, -0.0078125, -0.005859375, -0.00390625, -0.001953125, 0.0, 0.001953125, 0.00390625, 0.005859375, 0.0078125, 0.009765625, 0.01171875, 0.013671875, 0.015625, 0.017578125, 0.01953125, 0.021484375, 0.0234375, 0.025390625, 0.02734375, 0.029296875, 0.03125, 0.033203125, 0.03515625, 0.037109375, 0.0390625, 0.041015625, 0.04296875, 0.044921875, 0.046875, 0.048828125, 0.05078125, 0.052734375, 0.0546875, 0.056640625, 0.05859375, 0.060546875, 0.0625, 0.064453125, 0.06640625, 0.068359375, 0.0703125, 0.072265625, 0.07421875, 0.076171875, 0.078125, 0.080078125, 0.08203125, 0.083984375, 0.0859375, 0.087890625, 0.08984375, 0.091796875, 0.09375, 0.095703125, 0.09765625, 0.099609375, 0.1015625, 0.103515625, 0.10546875, 0.107421875, 0.109375, 0.111328125, 0.11328125, 0.115234375, 0.1171875, 0.119140625, 0.12109375, 0.123046875, 0.125, 0.126953125, 0.12890625, 0.130859375, 0.1328125, 0.134765625, 0.13671875, 0.138671875, 0.140625, 0.142578125, 0.14453125, 0.146484375, 0.1484375, 0.150390625, 0.15234375, 0.154296875, 0.15625, 0.158203125, 0.16015625, 0.162109375, 0.1640625, 0.166015625, 0.16796875, 0.169921875, 0.171875, 0.173828125, 0.17578125, 0.177734375, 0.1796875, 0.181640625, 0.18359375, 0.185546875, 0.1875, 0.189453125, 0.19140625, 0.193359375, 0.1953125, 0.197265625, 0.19921875, 0.201171875, 0.203125, 0.205078125, 0.20703125, 0.208984375, 0.2109375, 0.212890625, 0.21484375, 0.216796875, 0.21875, 0.220703125, 0.22265625, 0.224609375, 0.2265625, 0.228515625, 0.23046875, 0.232421875, 0.234375, 0.236328125, 0.23828125, 0.240234375, 0.2421875, 0.244140625, 0.24609375, 0.248046875, 0.25, 0.251953125, 0.25390625, 0.255859375, 0.2578125, 0.259765625, 0.26171875, 0.263671875, 0.265625, 0.267578125, 0.26953125, 0.271484375, 0.2734375, 0.275390625, 0.27734375, 0.279296875, 0.28125, 0.283203125, 0.28515625, 0.287109375, 0.2890625, 0.291015625, 0.29296875, 0.294921875, 0.296875, 0.298828125, 0.30078125, 0.302734375, 0.3046875, 0.306640625, 0.30859375, 0.310546875, 0.3125, 0.314453125, 0.31640625, 0.318359375, 0.3203125, 0.322265625, 0.32421875, 0.326171875, 0.328125, 0.330078125, 0.33203125, 0.333984375, 0.3359375, 0.337890625, 0.33984375, 0.341796875, 0.34375, 0.345703125, 0.34765625, 0.349609375, 0.3515625, 0.353515625, 0.35546875, 0.357421875, 0.359375, 0.361328125, 0.36328125, 0.365234375, 0.3671875, 0.369140625, 0.37109375, 0.373046875, 0.375, 0.376953125, 0.37890625, 0.380859375, 0.3828125, 0.384765625, 0.38671875, 0.388671875, 0.390625, 0.392578125, 0.39453125, 0.396484375, 0.3984375, 0.400390625, 0.40234375, 0.404296875, 0.40625, 0.408203125, 0.41015625, 0.412109375, 0.4140625, 0.416015625, 0.41796875, 0.419921875, 0.421875, 0.423828125, 0.42578125, 0.427734375, 0.4296875, 0.431640625, 0.43359375, 0.435546875, 0.4375, 0.439453125, 0.44140625, 0.443359375, 0.4453125, 0.447265625, 0.44921875, 0.451171875, 0.453125, 0.455078125, 0.45703125, 0.458984375, 0.4609375, 0.462890625, 0.46484375, 0.466796875, 0.46875, 0.470703125, 0.47265625, 0.474609375, 0.4765625, 0.478515625, 0.48046875, 0.482421875, 0.484375, 0.486328125, 0.48828125, 0.490234375, 0.4921875, 0.494140625, 0.49609375, 0.498046875, 0.5, 0.501953125, 0.50390625, 0.505859375, 0.5078125, 0.509765625, 0.51171875, 0.513671875, 0.515625, 0.517578125, 0.51953125, 0.521484375, 0.5234375, 0.525390625, 0.52734375, 0.529296875, 0.53125, 0.533203125, 0.53515625, 0.537109375, 0.5390625, 0.541015625, 0.54296875, 0.544921875, 0.546875, 0.548828125, 0.55078125, 0.552734375, 0.5546875, 0.556640625, 0.55859375, 0.560546875, 0.5625, 0.564453125, 0.56640625, 0.568359375, 0.5703125, 0.572265625, 0.57421875, 0.576171875, 0.578125, 0.580078125, 0.58203125, 0.583984375, 0.5859375, 0.587890625, 0.58984375, 0.591796875, 0.59375, 0.595703125, 0.59765625, 0.599609375, 0.6015625, 0.603515625, 0.60546875, 0.607421875, 0.609375, 0.611328125, 0.61328125, 0.615234375, 0.6171875, 0.619140625, 0.62109375, 0.623046875, 0.625, 0.626953125, 0.62890625, 0.630859375, 0.6328125, 0.634765625, 0.63671875, 0.638671875, 0.640625, 0.642578125, 0.64453125, 0.646484375, 0.6484375, 0.650390625, 0.65234375, 0.654296875, 0.65625, 0.658203125, 0.66015625, 0.662109375, 0.6640625, 0.666015625, 0.66796875, 0.669921875, 0.671875, 0.673828125, 0.67578125, 0.677734375, 0.6796875, 0.681640625, 0.68359375, 0.685546875, 0.6875, 0.689453125, 0.69140625, 0.693359375, 0.6953125, 0.697265625, 0.69921875, 0.701171875, 0.703125, 0.705078125, 0.70703125, 0.708984375, 0.7109375, 0.712890625, 0.71484375, 0.716796875, 0.71875, 0.720703125, 0.72265625, 0.724609375, 0.7265625, 0.728515625, 0.73046875, 0.732421875, 0.734375, 0.736328125, 0.73828125, 0.740234375, 0.7421875, 0.744140625, 0.74609375, 0.748046875, 0.75, 0.751953125, 0.75390625, 0.755859375, 0.7578125, 0.759765625, 0.76171875, 0.763671875, 0.765625, 0.767578125, 0.76953125, 0.771484375, 0.7734375, 0.775390625, 0.77734375, 0.779296875, 0.78125, 0.783203125, 0.78515625, 0.787109375, 0.7890625, 0.791015625, 0.79296875, 0.794921875, 0.796875, 0.798828125, 0.80078125, 0.802734375, 0.8046875, 0.806640625, 0.80859375, 0.810546875, 0.8125, 0.814453125, 0.81640625, 0.818359375, 0.8203125, 0.822265625, 0.82421875, 0.826171875, 0.828125, 0.830078125, 0.83203125, 0.833984375, 0.8359375, 0.837890625, 0.83984375, 0.841796875, 0.84375, 0.845703125, 0.84765625, 0.849609375, 0.8515625, 0.853515625, 0.85546875, 0.857421875, 0.859375, 0.861328125, 0.86328125, 0.865234375, 0.8671875, 0.869140625, 0.87109375, 0.873046875, 0.875, 0.876953125, 0.87890625, 0.880859375, 0.8828125, 0.884765625, 0.88671875, 0.888671875, 0.890625, 0.892578125, 0.89453125, 0.896484375, 0.8984375, 0.900390625, 0.90234375, 0.904296875, 0.90625, 0.908203125, 0.91015625, 0.912109375, 0.9140625, 0.916015625, 0.91796875, 0.919921875, 0.921875, 0.923828125, 0.92578125, 0.927734375, 0.9296875, 0.931640625, 0.93359375, 0.935546875, 0.9375, 0.939453125, 0.94140625, 0.943359375, 0.9453125, 0.947265625, 0.94921875, 0.951171875, 0.953125, 0.955078125, 0.95703125, 0.958984375, 0.9609375, 0.962890625, 0.96484375, 0.966796875, 0.96875, 0.970703125, 0.97265625, 0.974609375, 0.9765625, 0.978515625, 0.98046875, 0.982421875, 0.984375, 0.986328125, 0.98828125, 0.990234375, 0.9921875, 0.994140625, 0.99609375, 0.998046875, 1.0, 1.881610526243728], [nan, nan, nan, nan, nan, nan, nan, nan, nan, nan, nan, nan, nan, nan, nan, nan, nan, nan, nan, nan, nan, nan, nan, nan, nan, nan, nan, nan, nan, nan, nan, nan, nan, nan, nan, nan, nan, nan, nan, nan, nan, nan, nan, nan, nan, nan, nan, nan, nan, nan, nan, nan, nan, nan, nan, nan, nan, nan, nan, nan, nan, nan, nan, nan, nan, nan, nan, nan, nan, nan, nan, nan, nan, nan, nan, nan, nan, nan, nan, nan, nan, nan, nan, nan, nan, nan, nan, nan, nan, nan, nan, nan, nan, nan, nan, nan, nan, 10.0, 10.0, 10.0, 10.0, 10.0, 10.0, 10.0, 10.0, 10.0, 10.0, 10.0, 10.0, 10.0, 10.0, 10.0, 10.0, 10.0, 10.0, 10.0, 10.0, 10.0, 10.0, 10.0, 10.0, 10.0, nan, nan, nan, nan, nan, nan, nan, nan, nan, nan, nan, nan, nan, nan, nan, nan, nan, nan, nan, nan, nan, nan, nan, nan, nan, nan, nan, nan, nan, nan, nan, nan, nan, nan, nan, nan, nan, nan, nan, nan, nan, nan, nan, nan, nan, nan, nan, nan, nan, nan, nan, nan, nan, nan, nan, nan, nan, nan, nan, nan, nan, nan, nan, nan, nan, nan, nan, nan, nan, nan, nan, nan, nan, nan, nan, nan, nan, nan, nan, nan, nan, nan, nan, nan, nan, nan, nan, nan, nan, nan, nan, nan, nan, nan, nan, nan, nan, -1.0, -0.998046875, -0.99609375, -0.994140625, -0.9921875, -0.990234375, -0.98828125, -0.986328125, -0.984375, -0.982421875, -0.98046875, -0.978515625, -0.9765625, -0.974609375, -0.97265625, -0.970703125, -0.96875, -0.966796875, -0.96484375, -0.962890625, -0.9609375, -0.958984375, -0.95703125, -0.955078125, -0.953125, -0.951171875, -0.94921875, -0.947265625, -0.9453125, -0.943359375, -0.94140625, -0.939453125, -0.9375, -0.935546875, -0.93359375, -0.931640625, -0.9296875, -0.927734375, -0.92578125, -0.923828125, -0.921875, -0.919921875, -0.91796875, -0.916015625, -0.9140625, -0.912109375, -0.91015625, -0.908203125, -0.90625, -0.904296875, -0.90234375, -0.900390625, -0.8984375, -0.896484375, -0.89453125, -0.892578125, -0.890625, -0.888671875, -0.88671875, -0.884765625, -0.8828125, -0.880859375, -0.87890625, -0.876953125, -0.875, -0.873046875, -0.87109375, -0.869140625, -0.8671875, -0.865234375, -0.86328125, -0.861328125, -0.859375, -0.857421875, -0.85546875, -0.853515625, -0.8515625, -0.849609375, -0.84765625, -0.845703125, -0.84375, -0.841796875, -0.83984375, -0.837890625, -0.8359375, -0.833984375, -0.83203125, -0.830078125, -0.828125, -0.826171875, -0.82421875, -0.822265625, -0.8203125, -0.818359375, -0.81640625, -0.814453125, -0.8125, -0.810546875, -0.80859375, -0.806640625, -0.8046875, -0.802734375, -0.80078125, -0.798828125, -0.796875, -0.794921875, -0.79296875, -0.791015625, -0.7890625, -0.787109375, -0.78515625, -0.783203125, -0.78125, -0.779296875, -0.77734375, -0.775390625, -0.7734375, -0.771484375, -0.76953125, -0.767578125, -0.765625, -0.763671875, -0.76171875, -0.759765625, -0.7578125, -0.755859375, -0.75390625, -0.751953125, -0.75, -0.748046875, -0.74609375, -0.744140625, -0.7421875, -0.740234375, -0.73828125, -0.736328125, -0.734375, -0.732421875, -0.73046875, -0.728515625, -0.7265625, -0.724609375, -0.72265625, -0.720703125, -0.71875, -0.716796875, -0.71484375, -0.712890625, -0.7109375, -0.708984375, -0.70703125, -0.705078125, -0.703125, -0.701171875, -0.69921875, -0.697265625, -0.6953125, -0.693359375, -0.69140625, -0.689453125, -0.6875, -0.685546875, -0.68359375, -0.681640625, -0.6796875, -0.677734375, -0.67578125, -0.673828125, -0.671875, -0.669921875, -0.66796875, -0.666015625, -0.6640625, -0.662109375, -0.66015625, -0.658203125, -0.65625, -0.654296875, -0.65234375, -0.650390625, -0.6484375, -0.646484375, -0.64453125, -0.642578125, -0.640625, -0.638671875, -0.63671875, -0.634765625, -0.6328125, -0.630859375, -0.62890625, -0.626953125, -0.625, -0.623046875, -0.62109375, -0.619140625, -0.6171875, -0.615234375, -0.61328125, -0.611328125, -0.609375, -0.607421875, -0.60546875, -0.603515625, -0.6015625, -0.599609375, -0.59765625, -0.595703125, -0.59375, -0.591796875, -0.58984375, -0.587890625, -0.5859375, -0.583984375, -0.58203125, -0.580078125, -0.578125, -0.576171875, -0.57421875, -0.572265625, -0.5703125, -0.568359375, -0.56640625, -0.564453125, -0.5625, -0.560546875, -0.55859375, -0.556640625, -0.5546875, -0.552734375, -0.55078125, -0.548828125, -0.546875, -0.544921875, -0.54296875, -0.541015625, -0.5390625, -0.537109375, -0.53515625, -0.533203125, -0.53125, -0.529296875, -0.52734375, -0.525390625, -0.5234375, -0.521484375, -0.51953125, -0.517578125, -0.515625, -0.513671875, -0.51171875, -0.509765625, -0.5078125, -0.505859375, -0.50390625, -0.501953125, -0.5, -0.498046875, -0.49609375, -0.494140625, -0.4921875, -0.490234375, -0.48828125, -0.486328125, -0.484375, -0.482421875, -0.48046875, -0.478515625, -0.4765625, -0.474609375, -0.47265625, -0.470703125, -0.46875, -0.466796875, -0.46484375, -0.462890625, -0.4609375, -0.458984375, -0.45703125, -0.455078125, -0.453125, -0.451171875, -0.44921875, -0.447265625, -0.4453125, -0.443359375, -0.44140625, -0.439453125, -0.4375, -0.435546875, -0.43359375, -0.431640625, -0.4296875, -0.427734375, -0.42578125, -0.423828125, -0.421875, -0.419921875, -0.41796875, -0.416015625, -0.4140625, -0.412109375, -0.41015625, -0.408203125, -0.40625, -0.404296875, -0.40234375, -0.400390625, -0.3984375, -0.396484375, -0.39453125, -0.392578125, -0.390625, -0.388671875, -0.38671875, -0.384765625, -0.3828125, -0.380859375, -0.37890625, -0.376953125, -0.375, -0.373046875, -0.37109375, -0.369140625, -0.3671875, -0.365234375, -0.36328125, -0.361328125, -0.359375, -0.357421875, -0.35546875, -0.353515625, -0.3515625, -0.349609375, -0.34765625, -0.345703125, -0.34375, -0.341796875, -0.33984375, -0.337890625, -0.3359375, -0.333984375, -0.33203125, -0.330078125, -0.328125, -0.326171875, -0.32421875, -0.322265625, -0.3203125, -0.318359375, -0.31640625, -0.314453125, -0.3125, -0.310546875, -0.30859375, -0.306640625, -0.3046875, -0.302734375, -0.30078125, -0.298828125, -0.296875, -0.294921875, -0.29296875, -0.291015625, -0.2890625, -0.287109375, -0.28515625, -0.283203125, -0.28125, -0.279296875, -0.27734375, -0.275390625, -0.2734375, -0.271484375, -0.26953125, -0.267578125, -0.265625, -0.263671875, -0.26171875, -0.259765625, -0.2578125, -0.255859375, -0.25390625, -0.251953125, -0.25, -0.248046875, -0.24609375, -0.244140625, -0.2421875, -0.240234375, -0.23828125, -0.236328125, -0.234375, -0.232421875, -0.23046875, -0.228515625, -0.2265625, -0.224609375, -0.22265625, -0.220703125, -0.21875, -0.216796875, -0.21484375, -0.212890625, -0.2109375, -0.208984375, -0.20703125, -0.205078125, -0.203125, -0.201171875, -0.19921875, -0.197265625, -0.1953125, -0.193359375, -0.19140625, -0.189453125, -0.1875, -0.185546875, -0.18359375, -0.181640625, -0.1796875, -0.177734375, -0.17578125, -0.173828125, -0.171875, -0.169921875, -0.16796875, -0.166015625, -0.1640625, -0.162109375, -0.16015625, -0.158203125, -0.15625, -0.154296875, -0.15234375, -0.150390625, -0.1484375, -0.146484375, -0.14453125, -0.142578125, -0.140625, -0.138671875, -0.13671875, -0.134765625, -0.1328125, -0.130859375, -0.12890625, -0.126953125, -0.125, -0.123046875, -0.12109375, -0.119140625, -0.1171875, -0.115234375, -0.11328125, -0.111328125, -0.109375, -0.107421875, -0.10546875, -0.103515625, -0.1015625, -0.099609375, -0.09765625, -0.095703125, -0.09375, -0.091796875, -0.08984375, -0.087890625, -0.0859375, -0.083984375, -0.08203125, -0.080078125, -0.078125, -0.076171875, -0.07421875, -0.072265625, -0.0703125, -0.068359375, -0.06640625, -0.064453125, -0.0625, -0.060546875, -0.05859375, -0.056640625, -0.0546875, -0.052734375, -0.05078125, -0.048828125, -0.046875, -0.044921875, -0.04296875, -0.041015625, -0.0390625, -0.037109375, -0.03515625, -0.033203125, -0.03125, -0.029296875, -0.02734375, -0.025390625, -0.0234375, -0.021484375, -0.01953125, -0.017578125, -0.015625, -0.013671875, -0.01171875, -0.009765625, -0.0078125, -0.005859375, -0.00390625, -0.001953125, 0.0, 0.001953125, 0.00390625, 0.005859375, 0.0078125, 0.009765625, 0.01171875, 0.013671875, 0.015625, 0.017578125, 0.01953125, 0.021484375, 0.0234375, 0.025390625, 0.02734375, 0.029296875, 0.03125, 0.033203125, 0.03515625, 0.037109375, 0.0390625, 0.041015625, 0.04296875, 0.044921875, 0.046875, 0.048828125, 0.05078125, 0.052734375, 0.0546875, 0.056640625, 0.05859375, 0.060546875, 0.0625, 0.064453125, 0.06640625, 0.068359375, 0.0703125, 0.072265625, 0.07421875, 0.076171875, 0.078125, 0.080078125, 0.08203125, 0.083984375, 0.0859375, 0.087890625, 0.08984375, 0.091796875, 0.09375, 0.095703125, 0.09765625, 0.099609375, 0.1015625, 0.103515625, 0.10546875, 0.107421875, 0.109375, 0.111328125, 0.11328125, 0.115234375, 0.1171875, 0.119140625, 0.12109375, 0.123046875, 0.125, 0.126953125, 0.12890625, 0.130859375, 0.1328125, 0.134765625, 0.13671875, 0.138671875, 0.140625, 0.142578125, 0.14453125, 0.146484375, 0.1484375, 0.150390625, 0.15234375, 0.154296875, 0.15625, 0.158203125, 0.16015625, 0.162109375, 0.1640625, 0.166015625, 0.16796875, 0.169921875, 0.171875, 0.173828125, 0.17578125, 0.177734375, 0.1796875, 0.181640625, 0.18359375, 0.185546875, 0.1875, 0.189453125, 0.19140625, 0.193359375, 0.1953125, 0.197265625, 0.19921875, 0.201171875, 0.203125, 0.205078125, 0.20703125, 0.208984375, 0.2109375, 0.212890625, 0.21484375, 0.216796875, 0.21875, 0.220703125, 0.22265625, 0.224609375, 0.2265625, 0.228515625, 0.23046875, 0.232421875, 0.234375, 0.236328125, 0.23828125, 0.240234375, 0.2421875, 0.244140625, 0.24609375, 0.248046875, 0.25, 0.251953125, 0.25390625, 0.255859375, 0.2578125, 0.259765625, 0.26171875, 0.263671875, 0.265625, 0.267578125, 0.26953125, 0.271484375, 0.2734375, 0.275390625, 0.27734375, 0.279296875, 0.28125, 0.283203125, 0.28515625, 0.287109375, 0.2890625, 0.291015625, 0.29296875, 0.294921875, 0.296875, 0.298828125, 0.30078125, 0.302734375, 0.3046875, 0.306640625, 0.30859375, 0.310546875, 0.3125, 0.314453125, 0.31640625, 0.318359375, 0.3203125, 0.322265625, 0.32421875, 0.326171875, 0.328125, 0.330078125, 0.33203125, 0.333984375, 0.3359375, 0.337890625, 0.33984375, 0.341796875, 0.34375, 0.345703125, 0.34765625, 0.349609375, 0.3515625, 0.353515625, 0.35546875, 0.357421875, 0.359375, 0.361328125, 0.36328125, 0.365234375, 0.3671875, 0.369140625, 0.37109375, 0.373046875, 0.375, 0.376953125, 0.37890625, 0.380859375, 0.3828125, 0.384765625, 0.38671875, 0.388671875, 0.390625, 0.392578125, 0.39453125, 0.396484375, 0.3984375, 0.400390625, 0.40234375, 0.404296875, 0.40625, 0.408203125, 0.41015625, 0.412109375, 0.4140625, 0.416015625, 0.41796875, 0.419921875, 0.421875, 0.423828125, 0.42578125, 0.427734375, 0.4296875, 0.431640625, 0.43359375, 0.435546875, 0.4375, 0.439453125, 0.44140625, 0.443359375, 0.4453125, 0.447265625, 0.44921875, 0.451171875, 0.453125, 0.455078125, 0.45703125, 0.458984375, 0.4609375, 0.462890625, 0.46484375, 0.466796875, 0.46875, 0.470703125, 0.47265625, 0.474609375, 0.4765625, 0.478515625, 0.48046875, 0.482421875, 0.484375, 0.486328125, 0.48828125, 0.490234375, 0.4921875, 0.494140625, 0.49609375, 0.498046875, 0.5, 0.501953125, 0.50390625, 0.505859375, 0.5078125, 0.509765625, 0.51171875, 0.513671875, 0.515625, 0.517578125, 0.51953125, 0.521484375, 0.5234375, 0.525390625, 0.52734375, 0.529296875, 0.53125, 0.533203125, 0.53515625, 0.537109375, 0.5390625, 0.541015625, 0.54296875, 0.544921875, 0.546875, 0.548828125, 0.55078125, 0.552734375, 0.5546875, 0.556640625, 0.55859375, 0.560546875, 0.5625, 0.564453125, 0.56640625, 0.568359375, 0.5703125, 0.572265625, 0.57421875, 0.576171875, 0.578125, 0.580078125, 0.58203125, 0.583984375, 0.5859375, 0.587890625, 0.58984375, 0.591796875, 0.59375, 0.595703125, 0.59765625, 0.599609375, 0.6015625, 0.603515625, 0.60546875, 0.607421875, 0.609375, 0.611328125, 0.61328125, 0.615234375, 0.6171875, 0.619140625, 0.62109375, 0.623046875, 0.625, 0.626953125, 0.62890625, 0.630859375, 0.6328125, 0.634765625, 0.63671875, 0.638671875, 0.640625, 0.642578125, 0.64453125, 0.646484375, 0.6484375, 0.650390625, 0.65234375, 0.654296875, 0.65625, 0.658203125, 0.66015625, 0.662109375, 0.6640625, 0.666015625, 0.66796875, 0.669921875, 0.671875, 0.673828125, 0.67578125, 0.677734375, 0.6796875, 0.681640625, 0.68359375, 0.685546875, 0.6875, 0.689453125, 0.69140625, 0.693359375, 0.6953125, 0.697265625, 0.69921875, 0.701171875, 0.703125, 0.705078125, 0.70703125, 0.708984375, 0.7109375, 0.712890625, 0.71484375, 0.716796875, 0.71875, 0.720703125, 0.72265625, 0.724609375, 0.7265625, 0.728515625, 0.73046875, 0.732421875, 0.734375, 0.736328125, 0.73828125, 0.740234375, 0.7421875, 0.744140625, 0.74609375, 0.748046875, 0.75, 0.751953125, 0.75390625, 0.755859375, 0.7578125, 0.759765625, 0.76171875, 0.763671875, 0.765625, 0.767578125, 0.76953125, 0.771484375, 0.7734375, 0.775390625, 0.77734375, 0.779296875, 0.78125, 0.783203125, 0.78515625, 0.787109375, 0.7890625, 0.791015625, 0.79296875, 0.794921875, 0.796875, 0.798828125, 0.80078125, 0.802734375, 0.8046875, 0.806640625, 0.80859375, 0.810546875, 0.8125, 0.814453125, 0.81640625, 0.818359375, 0.8203125, 0.822265625, 0.82421875, 0.826171875, 0.828125, 0.830078125, 0.83203125, 0.833984375, 0.8359375, 0.837890625, 0.83984375, 0.841796875, 0.84375, 0.845703125, 0.84765625, 0.849609375, 0.8515625, 0.853515625, 0.85546875, 0.857421875, 0.859375, 0.861328125, 0.86328125, 0.865234375, 0.8671875, 0.869140625, 0.87109375, 0.873046875, 0.875, 0.876953125, 0.87890625, 0.880859375, 0.8828125, 0.884765625, 0.88671875, 0.888671875, 0.890625, 0.892578125, 0.89453125, 0.896484375, 0.8984375, 0.900390625, 0.90234375, 0.904296875, 0.90625, 0.908203125, 0.91015625, 0.912109375, 0.9140625, 0.916015625, 0.91796875, 0.919921875, 0.921875, 0.923828125, 0.92578125, 0.927734375, 0.9296875, 0.931640625, 0.93359375, 0.935546875, 0.9375, 0.939453125, 0.94140625, 0.943359375, 0.9453125, 0.947265625, 0.94921875, 0.951171875, 0.953125, 0.955078125, 0.95703125, 0.958984375, 0.9609375, 0.962890625, 0.96484375, 0.966796875, 0.96875, 0.970703125, 0.97265625, 0.974609375, 0.9765625, 0.978515625, 0.98046875, 0.982421875, 0.984375, 0.986328125, 0.98828125, 0.990234375, 0.9921875, 0.994140625, 0.99609375, 0.998046875]]
  in  "Scan Benchmark":bool
  in  "Offset Y [V]":dbl format="%.2f"
  in  "Calibration Factor Y [V/mm]":dbl=1.0 format="%.2f"
  in  "Set Position Y [mm]":dbl(slide) min=-10.0 max=10.0 step=0.1 scale=-10.0..10.0
  in  "Load.ini":bool
  in  "Offset X [V]":dbl format="%.2f"
  in  "Calibration Factor X [V/mm]":dbl=1.0 format="%.2f"
  in  "Set Position X [mm]":dbl(slide) min=-10.0 max=10.0 step=0.1 scale=-10.0..10.0
  in  "System":enum16{"Probe", "Handheld", "Microscope"}(ring)
  in  "Scan Rate [Hz]":dbl=1000.0 min=1000.0 max=300000.0 step=10000.0 format="%#_6p"
  in  "Angle [°]":dbl min=0.0 max=360.0 step=45.0
  in  "Write Config":bool
  out "Dispersion":sgl[](graph)
  in  "Repeated LambdaToK":bool
  out "Chirp":sgl[](graph)
  out "Image":T3(plugin-control)
  in  "Intensity Ring Light":i32(slide) scale=0.0..100.0
  in  "LambdaToKMisc":bool
  out "OverlayImage 2":T3(plugin-control)
  in  "Probe":enum16{"Probe", "Handheld", "Microscope"}(ring)
  in  "Calibrate Surface":bool
  in  "RangeY [mm]":dbl=10.0
  in  "Number Scans Y":i32=100
  in  "RangeX [mm]":dbl=10.0
  in  "Number Scans X":i32=100 min=25 step=25
  in  "Range X [mm]":dbl=2.5 min=0.5 max=10.0 step=0.10000000149011612 format="%_2f"
  in  "Scans Y":i32=200 min=50 max=300
  in  "Range Y [mm]":dbl=2.5 min=0.5 max=10.0 format="%_2f"
  in  "Scans X":i32=320 min=50 max=300
  in  "Scan":bool
  in  "dB":cluster{sgl, sgl}(slide)={44.599304, 80.13937} caption="Boundries 2" scale=-20.0..150.0
  out "OverlayImage":T3(plugin-control)
  in  "Offset X":i32(slide) min=0 max=640 step=1 scale=0.0..640.0
  in  "Offset Y":i32(slide)=200 min=0 max=480 step=1
  in  "Scan Contrast":sgl(knob) caption="Scan" min=0 max=1 scale=0.0..1.0
  in  "Rotation [deg]":sgl(slide) step=0.01 scale=-180.0..270.0
  in  "Scaling [px/mm]":sgl(slide)=1.0 min=-200 max=200 step=0.01 scale=-200.0..200.0
  in  "Show Scan":bool
  in  "Save Handheld":bool
  out "3D Surface":refnum<class "3D Plot Datatype.lvclass">[](xcontrol)
  in  "Reset":bool
  in  "Save WB":bool
  in  "Save calibration":bool
  out "OffsetX":sgl
  out "OffsetY":sgl
  out "FactorX":sgl=1.0
  out "FactorY":sgl=1.0
  out "Camera Scaling X":sgl
  out "Camera Scaling Y":sgl
  out "Camera Offset X":sgl
  out "Camera Offset Y":sgl
  out "Camera Angle":sgl
  in  "Ring Light Intensity [%]":dbl(slide)=10.0 scale=0.0..100.0
  out "Calibration Image":T3(plugin-control)
  # "Maximum"
  # "Peak"
  # "Noise"
  # "Z-Calibration"
  # "Version 5.0"
  # "White Balance Settings"
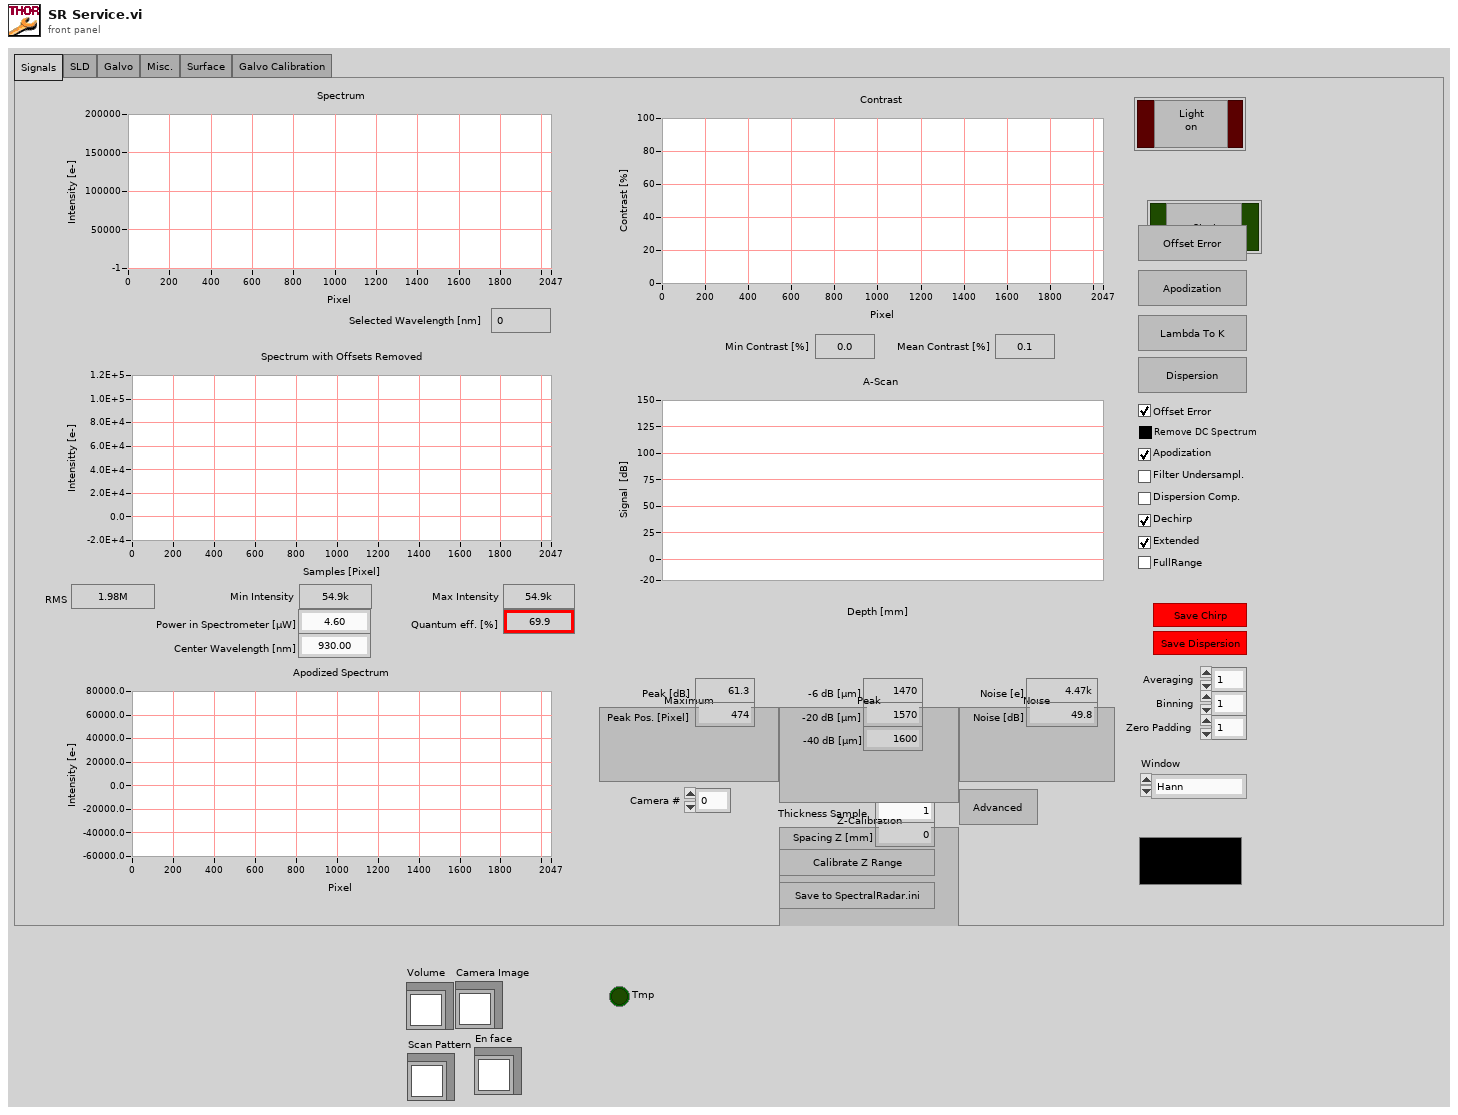
[diagram p1: front panel]
types:
  T1 = enum32{"Signals", "SLD", "Galvo", "Misc.", "Surface", "Galvo Calibration"}
  T2 = enum16{"Hann", "Hamming", "Gauss", "Tapered Cosine", "Blackman", "4 Term B-Harris"}
  T3 = typedef "IMAQ Image.ctl" = refnum<image>
  T4 = enum32{"Signals", "SLD", "Galvo", "Misc.", "Surface"}
  T5 = enum16{"isOn", "Camera Available", "SLD Available", "SLD Status", "Laser Diode Status", "Camera Show Scan Pattern"}
  T6 = typedef "Coloring.lvclass/Coloring Byteorder.ctl" = enum16{"RGBA32", "BGRA32", "ARGB32", ""}
  T7 = typedef "Processing.lvclass/Processing Flag Selection.ctl" = enum16{"Use Offset Errors", "Remove DC Spectrum", "Remove Advanced DC Spectrum", "Use Apodization", "Use Scan For Apodization", "Filter Undersampled Signals", "Use Dispersion Compensation", "Use Dechirp", "Use Extended Adjust", "Full Range Output", "Filter DC", "Autocorrelation Compensation", "DEFR", "Only Windowing", "Remove Fixed Pattern"}
  T8 = enum16{"Full Well Capacity", "z Spacing", "z Range", "Dynamc Range Min [dB]", "Dynamic Range Low [dB]", "Dynamic Range High [dB]", "Dynamic Range Max [dB]"}
  T9 = typedef "Coloring.lvclass/Colorscheme Selection.ctl" = enum16{"Black And White", "Inverted Black And White", "Color", "Black and Orange", "Black and Red", "Doppler Phase Coloring"}
  T10 = typedef "OCT Device.lvclass/Device Property Float Selection.ctl" = enum16{"Full Well Capacity", "z Spacing", "z Range", "Dynamc Range Min [dB]", "Dynamic Range Low [dB]", "Dynamic Range High [dB]", "Dynamic Range Max [dB]", "Binary-To-Electron Scaling Factor", "Device Temperature [°C]", "SLD online time [s]", "Central Wavelength [nm]", "Spectral Width [nm]"}
  T11 = typedef "OCT Device.lvclass/Device Property Int Selection.ctl" = enum16{"Spectrum Elements", "Bytes per Spectrometer Element", "Max Live Volume Rendering Scans", "Device Bit Depth", "Number of Cameras", "Revision Number"}
  T12 = typedef "Probe.lvclass/Probe Parameter Float Selection.ctl" = enum16{"Factor X", "Offset X", "Factor Y", "Offset Y", "Flyback Time [s]", "Expansion Time [s]", "Rotation Time [s]", "Expected Scan Rate [Hz]", "Camera Scaling X", "Camera Offset X", "Camera Scaling Y", "Camera Offset Y", "Angle", "White Balance Red", "White Balance Green", "White Balance Blue", "Max. Range X", "Max. Range Y", "Max. Slope XY", "Speckle Size"}
  T13 = typedef "Processing.lvclass/Calibration Selection.ctl" = enum16{"Offset Errors", "Apodization Spectrum", "Apodization Vector", "Dispersion", "Chirp", "Extended Adjust", "Fixed Pattern"}
  T14 = enum32{"Signals", "SLD", "Galvo", "Wellness", "Misc.", "Surface"}
  T15 = typedef "Processing.lvclass/Processing Parameter Int Selection.ctl" = enum32{"Spectrum Averaging", "A-Scan Averaging", "B-Scan Averaging", "Zero Padding", "Number of Threads", "Fourier Averaging"}
  T16 = enum16{"Asynchronous Continuous", "Asynchronous Finite", "Synchronous"}
  T17 = typedef "Data.lvclass/Normal Direction Selection.ctl" = enum16{"Direction 1", "Direction 2", "Direction 3"}
  T18 = typedef "Data.lvclass/Data Analyzation Selection.ctl" = enum16{"Min", "Mean", "Max"}
  T19 = enum32{"Lab Version", "SLD", "Galvo", "Wellness", "Misc.", "Surface"}
  T20 = typedef "Data.lvclass/A-Scan Analysis Selection.ctl" = enum16{"Noise [dB]", "Noise [e-]", "Peak Pos [Pixel]", "Peak Pos [mm]", "Peak Height [dB]", "Peak Width -6dB [Pixel]", "Peak Width -20dB [Pixel]", "Peak Width -40 dB [Pixel]", "Peak Phase"}
  T21 = typedef "Image Type" = u32
  T22 = typedef "Processing.lvclass/Apodization Window Selection.ctl" = enum16{"Hann", "Hamming", "Gauss", "Tapered Cosine", "Blackman", "4 Term B-Harris", "Light Source Based"}
  T23 = typedef "DialogType.ctl" = u16
  T24 = enum8{"Enabled", "Disabled", "Disabled and Grayed Out"}
  T25 = cluster{"Property Value":dbl, "Property Value":dbl}
  T26 = typedef "NI_LVConfig.lvlib/Config Data RefNum.ctl" = refnum<k1>
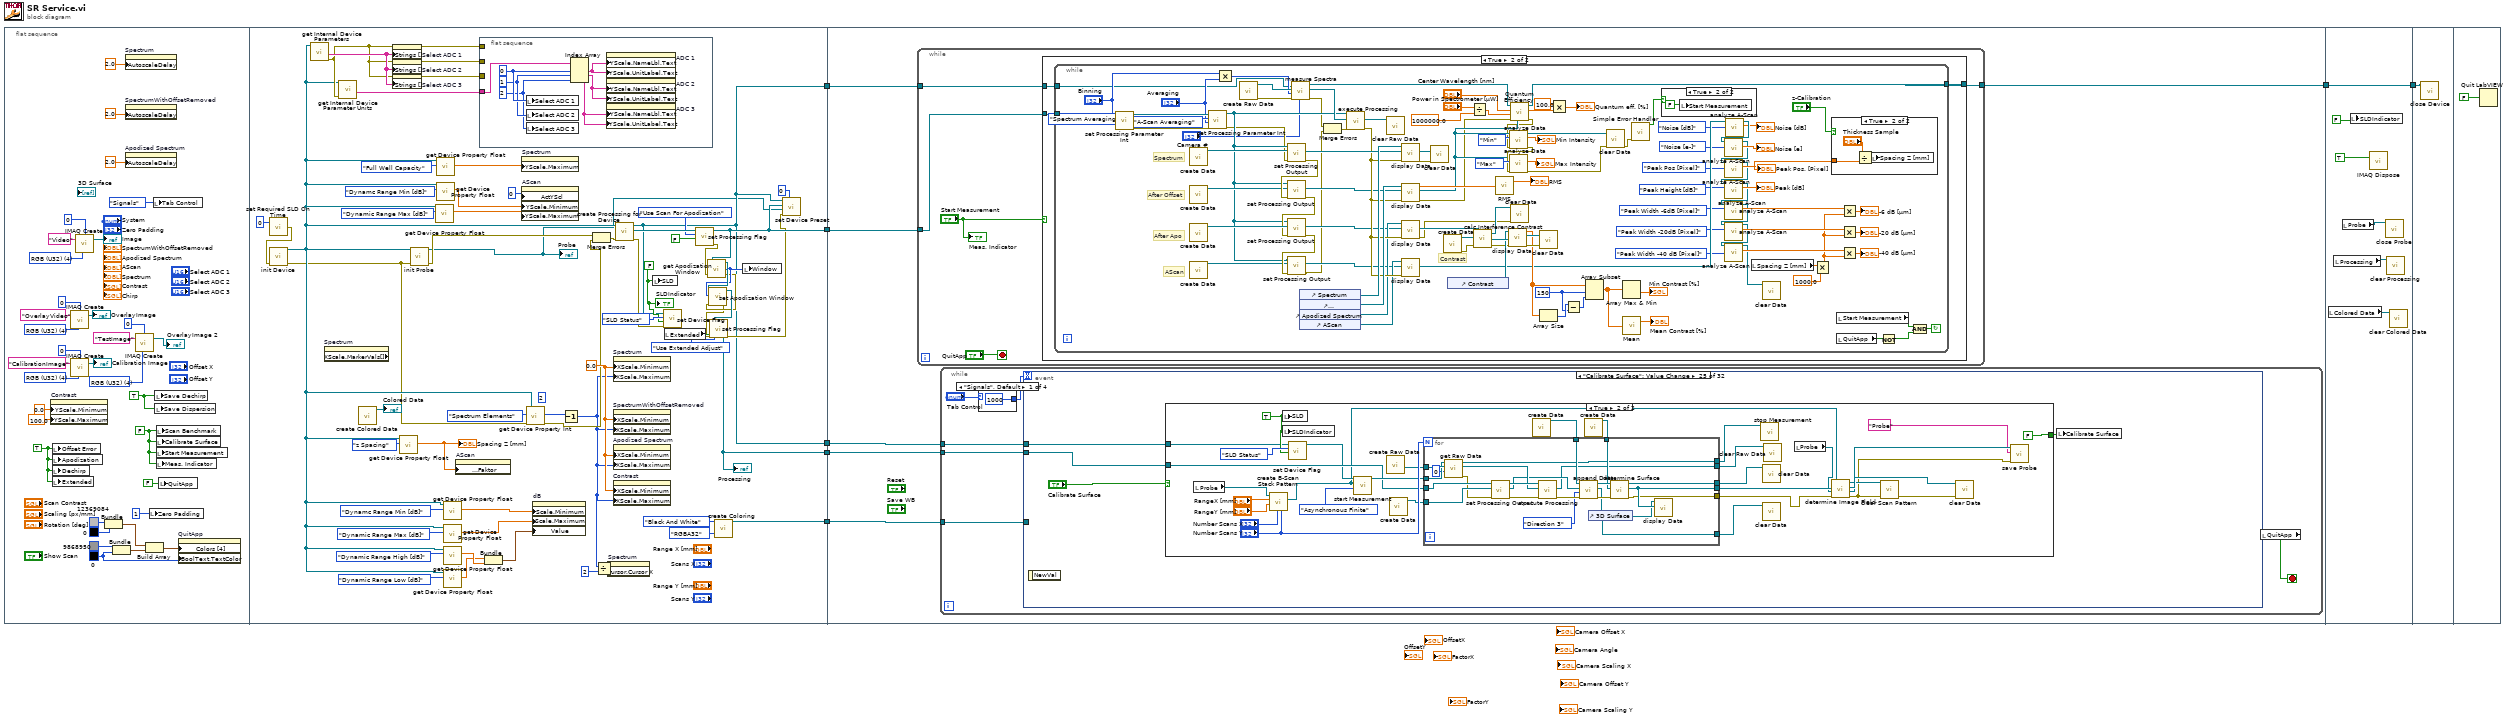
[diagram p0: block diagram]
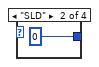
[diagram p2: hidden frame]
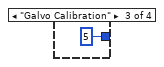
[diagram p3: hidden frame]
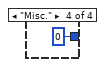
[diagram p4: hidden frame]
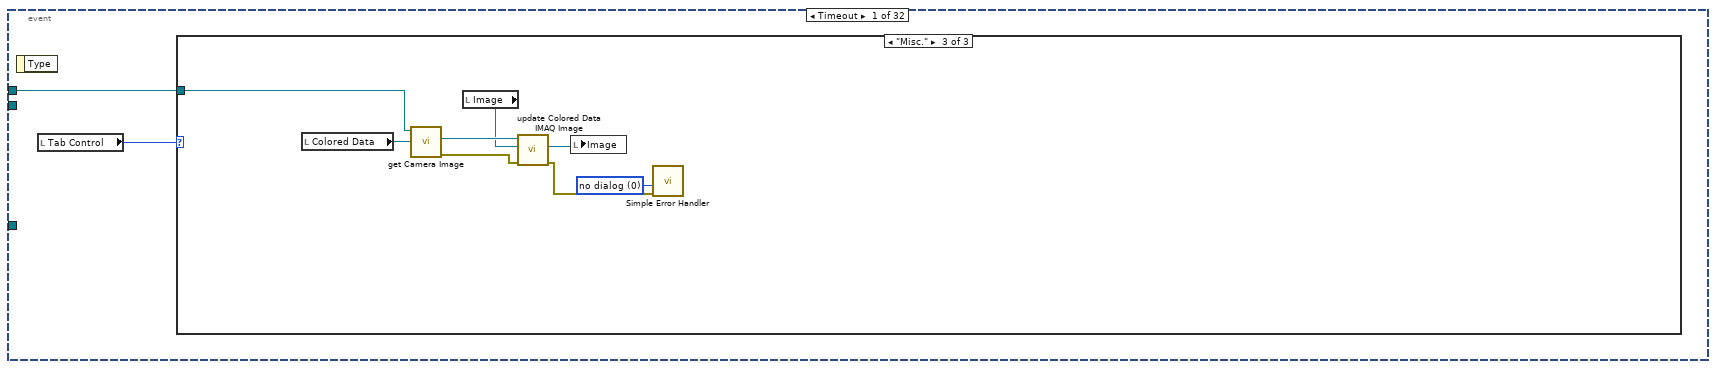
[diagram p5: hidden frame]
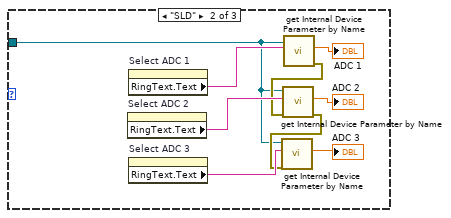
[diagram p7: hidden frame]
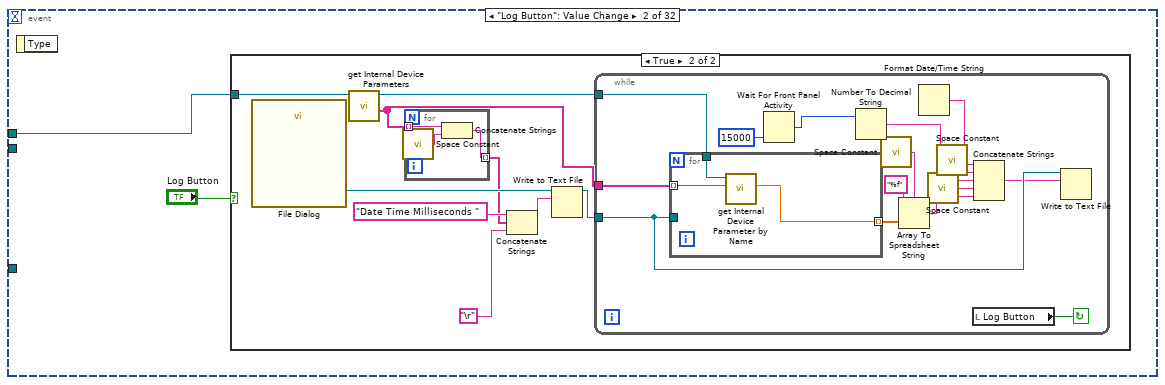
[diagram p8: hidden frame]
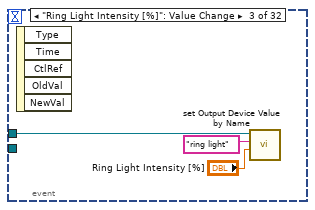
[diagram p10: hidden frame]
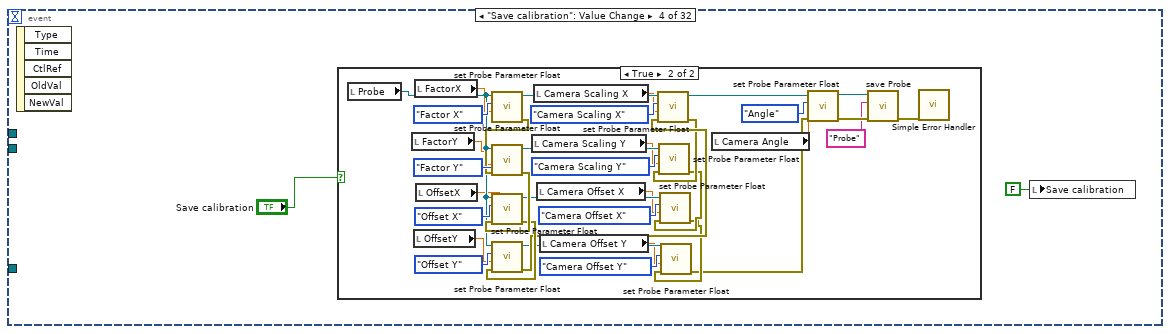
[diagram p11: hidden frame]
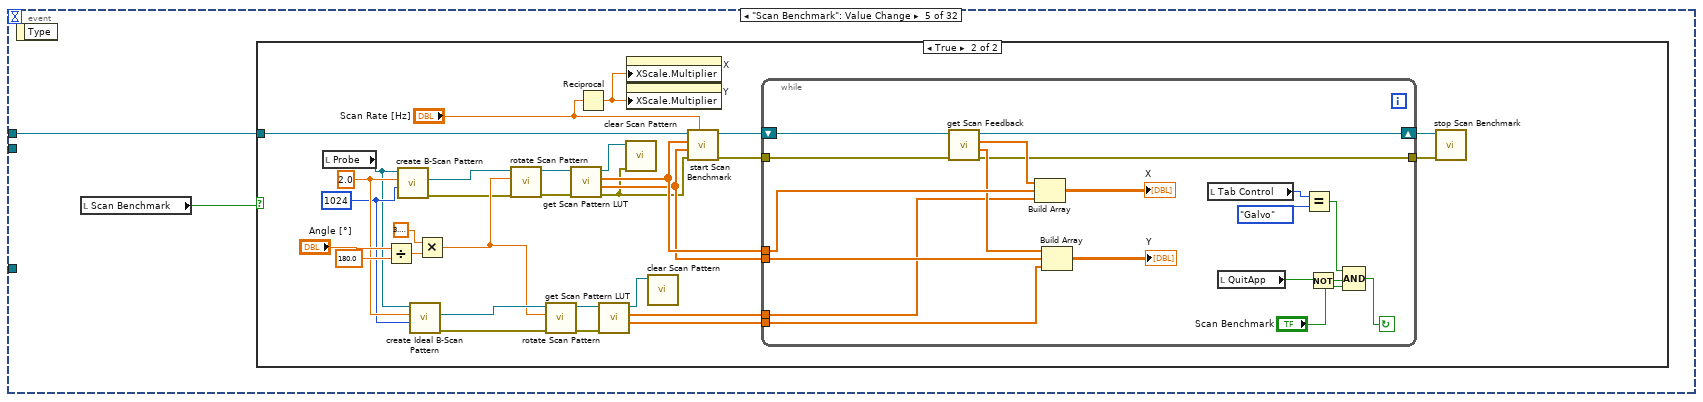
[diagram p13: hidden frame]
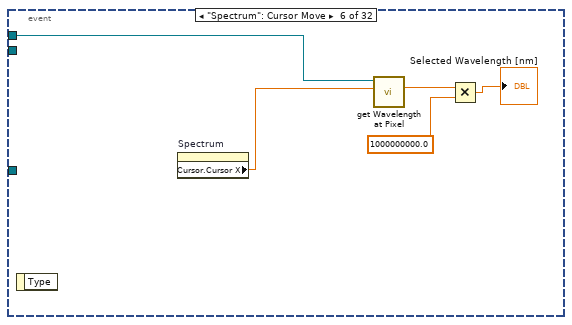
[diagram p15: hidden frame]
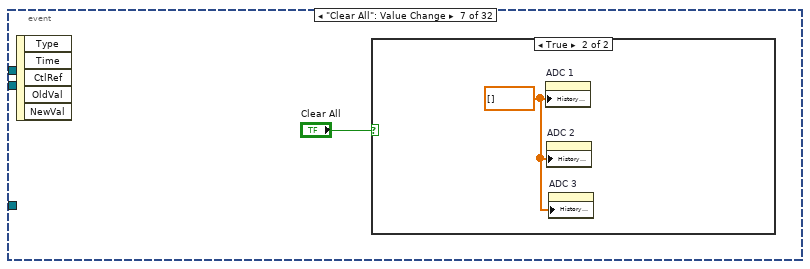
[diagram p16: hidden frame]
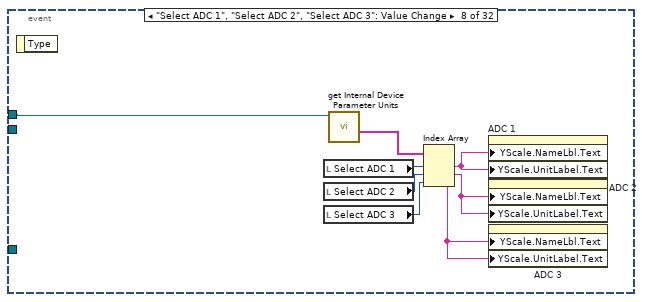
[diagram p18: hidden frame]
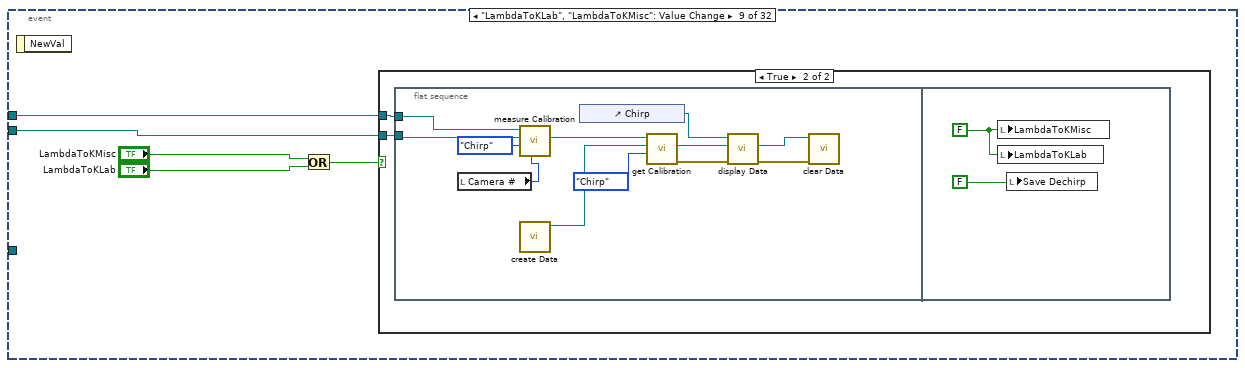
[diagram p19: hidden frame]
diagram:
  n1 = flat-sequence {
    tunnel: [w46] -> w7
    tunnel: [w51] -> w5
    tunnel: [w46] -> w4
    tunnel: [w62] -> w3
    tunnel: [w81] -> w1
    tunnel: w7 -> [w115]
    tunnel: [w114] -> w6
    tunnel: w5 -> [w113]
    tunnel: w4 -> [w112]
    tunnel: w3 -> [w111]
    tunnel: w1 -> [w110]
    tunnel: w6 -> [w1028]
    tunnel: [w1028] -> w2
    tunnel: w2 -> [w1033]
    frame #0 {
      w8 = T21 4 items=["Grayscale (U8)", "Grayscale (I16)", "Grayscale (SGL)", "Complex (CSG)", "RGB (U32)", "HSL (U32)", "RGB (U64)", "Grayscale (U16)"] ("Image Type")
      w13 = T21 4 items=["Grayscale (U8)", "Grayscale (I16)", "Grayscale (SGL)", "Complex (CSG)", "RGB (U32)", "HSL (U32)", "RGB (U64)", "Grayscale (U16)"] ("Image Type")
      w18 = T21 4 items=["Grayscale (U8)", "Grayscale (I16)", "Grayscale (SGL)", "Complex (CSG)", "RGB (U32)", "HSL (U32)", "RGB (U64)", "Grayscale (U16)"] ("Image Type")
      w26 = T21 4 items=["Grayscale (U8)", "Grayscale (I16)", "Grayscale (SGL)", "Complex (CSG)", "RGB (U32)", "HSL (U32)", "RGB (U64)", "Grayscale (U16)"] ("Image Type")
      w33 = u32 0
      w21 = TRUE ("Save Calibration")
      w38 = TRUE ("Offset Error")
      w22 = FALSE ("Start\nMeasurement")
      n2 = property on="Contrast" class="WFGraph (strict)"("YScale.Minimum"=0.0 ("y-Achse.Bereich:Minimum"), "YScale.Maximum"=100.0 ("y-Achse.Bereich:Maximum")) -> ()  [unwired: 2 in, 2 out]
      n3 = local write "Offset Error"(w38) -> ()
      n4 = local write "Apodization"(w38) -> ()
      n5 = local write "Dechirp"(w38) -> ()
      n6 = local write "Extended"(w38) -> ()
      n7 = call "IMAQ Create"("Border Size"=0, "Image Name"="OverlayVideo", "Image Type"=w18) -> ("New Image"=→"OverlayImage":T3)  [unwired: 2 in, 1 out]
      n8 = call "IMAQ Create"("Border Size"=0, "Image Name"="CalibrationImage", "Image Type"=w13) -> ("New Image"=→"Calibration Image":T3)  [unwired: 2 in, 1 out]
      n9 = call "IMAQ Create"("Border Size"=0, "Image Name"="Video", "Image Type"=w26) -> ("New Image"=→"Image":T3)  [unwired: 2 in, 1 out]
      n10 = Bundle(u32 12369084, u32 0) -> (w30:cluster{u32, u32})  [unwired: 1 in]
      n11 = Bundle(u32 9868950, w33) -> (w31:cluster{u32, u32})  [unwired: 1 in]
      n12 = property on="Spectrum" class="WFGraph (strict)"("AutoscaleDelay"=sgl 2.0 ("Autoskalierung verzögern")) -> ()  [unwired: 2 in, 2 out]
      n13 = property on="SpectrumWithOffsetRemoved" class="WFGraph (strict)"("AutoscaleDelay"=sgl 2.0 ("Autoskalierung verzögern")) -> ()  [unwired: 2 in, 2 out]
      n14 = property on="Apodized Spectrum" class="WFGraph (strict)"("AutoscaleDelay"=sgl 2.0 ("Autoskalierung verzögern")) -> ()  [unwired: 2 in, 2 out]
      n15 = call "IMAQ Create"("Border Size"=0, "Image Name"="TestImage", "Image Type"=w8) -> ("New Image"=→"OverlayImage 2":T3)  [unwired: 2 in, 1 out]
      n16 = Build Array(w30, w31) -> (w32:cluster{u32, u32}[])
      n17 = local write "Zero Padding"(1 ("Zero Padding")) -> ()
      n18 = local write "Tab Control"(T4."Signals" ("Tab Control")) -> ()
      n19 = local write "Save Dechirp"(w21) -> ()
      n20 = local write "Save Dispersion"(w21) -> ()
      n21 = local write "Scan Benchmark"(w22) -> ()
      n22 = local write "Calibrate Surface"(w22) -> ()
      n23 = local write "Start Measurement"(w22) -> ()
      n24 = local write "Meas. Indicator"(w22) -> ()
      n25 = local write "QuitApp"(FALSE ("Hauptereignisschleife")) -> ()
      n26 = property on="QuitApp" class="Bool (strict)"("Colors [4]"=w32, "BoolText.TextColor"=w33) -> ()  [unwired: 2 in, 2 out]
    }
    frame #1 {
      (unwired) u32 2 ("y")
      w87 = 0.0 ("x-Achse.Bereich:Minimum")
      w48 = FALSE ("Licht an (true) / aus (false)")
      n27 = call "set Required SLD On Time.vi"("Numeric Control"=0) -> ("error out"=w43:errorcluster)  [unwired: 1 in]
      n28 = call "init Device.vi"("error in (no error)"=w43) -> ("error out"=w67:errorcluster, "OCTDevice"=w71:refnum<class "OCT Device.lvclass">)  [unwired: 5 in]
      n29 = call "get Internal Device Parameters.vi"("OCTDevice"=w71) -> ("error out"=w99:errorcluster, "ADCs"=w101:string[])  [unwired: 3 in, 2 out]
      n30 = property on="Spectrum" class="WFGraph (strict)" props=["XScale", "MarkerVals[]"]() -> ()  [unwired: 2 in, 3 out]
      n31 = call "get Internal Device Parameter Units.vi"("error in (no error)"=w99, "OCTDevice"=w71) -> ("Units"=w100:string[])  [unwired: 2 in, 3 out]
      n32 = call "create Colored Data.vi"() -> ("Colored Data"=→"Colored Data":refnum<class "Colored Data.lvclass">)  [unwired: 6 in, 1 out]
      n33 = property on="Select ADC 1" class="Ring (strict)"(error in=w99, "Strings []"=w101) -> (error out=w90:errorcluster)  [unwired: 1 in, 1 out]
      n34 = property on="Select ADC 2" class="Ring (strict)"(error in=w99, "Strings []"=w101) -> (error out=w89:errorcluster)  [unwired: 1 in, 1 out]
      n35 = property on="Select ADC 3" class="Ring (strict)"(error in=w99, "Strings []"=w101) -> (error out=w88:errorcluster)  [unwired: 1 in, 1 out]
      n36 = call "get Device Property Float.vi"("Device Property Float Selection"=T8."z Spacing", "OCTDevice"=w71) -> ("Value"=w97:dbl)  [unwired: 3 in, 2 out]
      "Spacing Z [mm]" <- w97
      n37 = call "init Probe.vi"("error in (no error)"=w67, "OCT Device"=w71) -> ("error out"=w45:errorcluster, "GalvoControl"=w44:refnum<class "Probe.lvclass">)  [unwired: 4 in]
      "Probe" <- w44
      n38 = call "get Device Property Float.vi"("Device Property Float Selection"=T8."Dynamic Range Max [dB]", "OCTDevice"=w71) -> ("Value"=w93:dbl)  [unwired: 3 in, 2 out]
      n39 = call "get Device Property Float.vi"("Device Property Float Selection"=T8."Dynamc Range Min [dB]", "OCTDevice"=w71) -> ("Value"=w94:dbl)  [unwired: 3 in, 2 out]
      n40 = call "get Device Property Float.vi"("Device Property Float Selection"=Device_Property_Float_Selection."Full Well Capacity", "OCTDevice"=w71) -> ("Value"=w83:dbl)  [unwired: 3 in, 2 out]
      n41 = call "get Device Property Float.vi"("Device Property Float Selection"=T8."Dynamc Range Min [dB]", "OCTDevice"=w71) -> ("Value"=w77:dbl)  [unwired: 3 in, 2 out]
      n42 = call "get Device Property Float.vi"("Device Property Float Selection"=T8."Dynamic Range Max [dB]", "OCTDevice"=w71) -> ("Value"=w76:dbl)  [unwired: 3 in, 2 out]
      n43 = call "get Device Property Float.vi"("Device Property Float Selection"=T8."Dynamic Range High [dB]", "OCTDevice"=w71) -> ("Value"=w80:dbl)  [unwired: 3 in, 2 out]
      n44 = call "get Device Property Float.vi"("Device Property Float Selection"=T8."Dynamic Range Low [dB]", "OCTDevice"=w71) -> ("Value"=w79:dbl)  [unwired: 3 in, 2 out]
      n45 = property on="AScan" class="WFGraph (strict)"("x-Achse.Offset und Faktor:Faktor"=w97) -> ()  [unwired: 2 in, 2 out]
      n46 = flat-sequence {
        tunnel: w100 -> [w106]
        tunnel: w90 -> [_]
        tunnel: w89 -> [_]
        tunnel: w88 -> [_]
        frame #0 {
          w103 = 2 ("index")
          w104 = 1 ("index")
          w105 = 0 ("index")
          n47 = local write "Select ADC 1"(w105) -> ()
          n48 = local write "Select ADC 2"(w104) -> ()
          n49 = local write "Select ADC 3"(w103) -> ()
          n50 = Index Array(array=w106, index #1=w105, index #2=w104, index #3=w103) -> (element #1=w109:string, element #2=w108:string, element #3=w107:string)
          n51 = property on="ADC 1" class="WFChart (strict)"("YScale.NameLbl.Text"=w109, "YScale.UnitLabel.Text"=w109) -> ()  [unwired: 2 in, 2 out]
          n52 = property on="ADC 2" class="WFChart (strict)"("YScale.NameLbl.Text"=w108, "YScale.UnitLabel.Text"=w108) -> ()  [unwired: 2 in, 2 out]
          n53 = property on="ADC 3" class="WFChart (strict)"("YScale.NameLbl.Text"=w107, "YScale.UnitLabel.Text"=w107) -> ()  [unwired: 2 in, 2 out]
        }
      }
      n54 = Bundle("Value"=w79, "Value"=w80) -> (w78:cluster{"Value":dbl, "Value":dbl})  [unwired: 1 in]
      n55 = property on="Spectrum" class="WFGraph (strict)"("YScale.Maximum"=w83) -> ()  [unwired: 2 in, 2 out]
      n56 = property on="AScan" class="WFGraph (strict)"("ActYScl"=0 ("Aktive y-Achse"), "YScale.Minimum"=w94, "YScale.Maximum"=w93) -> ()  [unwired: 2 in, 2 out]
      n57 = call "get Device Property Int.vi"("error in (no error)"=w67, "Device Property Int Selection"=Device_Property_Int_Selection."Spectrum Elements", "OCTDevice"=w71) -> ("error out"=w66:errorcluster, "Value"=w86:i32)  [unwired: 2 in, 1 out]
      n58 = property on="dB" class="Slide (strict)"("Scale.Minimum"=w77, "Scale.Maximum"=w76, "Value"=w78) -> ()  [unwired: 2 in, 2 out]
      n59 = Decrement(x=w86) -> (x-1=w64:i32)
      n60 = Merge Errors(w45, w66) -> (w98:errorcluster)
      n61 = Divide(x=w64, y=2) -> (x/y=w65:dbl)
      n62 = property on="Spectrum" class="WFGraph (strict)"("Cursor.Cursor X"=w65) -> ()  [unwired: 2 in, 2 out]
      n63 = property on="Spectrum" class="WFGraph (strict)"("XScale.Minimum"=w87, "XScale.Maximum"=w64) -> ()  [unwired: 2 in, 2 out]
      n64 = property on="SpectrumWithOffsetRemoved" class="WFGraph (strict)"("XScale.Minimum"=w87, "XScale.Maximum"=w64) -> ()  [unwired: 2 in, 2 out]
      n65 = property on="Apodized Spectrum" class="WFGraph (strict)"("XScale.Minimum"=w87, "XScale.Maximum"=w64) -> ()  [unwired: 2 in, 2 out]
      n66 = property on="Contrast" class="WFGraph (strict)"("XScale.Minimum"=w87, "XScale.Maximum"=w64) -> ()  [unwired: 2 in, 2 out]
      n67 = call "create Processing for Device.vi"("error in (no error)"=w98, "OCTDevice"=w71) -> ("error out"=w47:errorcluster, "Processing"=w70:refnum<class "Processing.lvclass">, "OCTDevice"=w46:refnum<class "OCT Device.lvclass">)  [unwired: 3 in]
      n68 = local write "SLD"(w48) -> ()
      n69 = call "set Device Flag.vi"("error in (no error)"=w47, "Boolean"=w48, "Device Property Flag Selection"=T5."SLD Status", "OCTDevice"=w46) -> ()  [unwired: 6 in, 2 out]
      n70 = local read "Extended"() -> (w60:bool)
      n71 = call "set Processing Flag.vi"("Flag"=FALSE, "Processing Flag Selection"=Processing_Flag_Selection."Use Scan For Apodization", "Processing"=w70) -> ("error out"=w56:errorcluster, "Processing"=w51:refnum<class "Processing.lvclass">)  [unwired: 3 in]
      n72 = call "get Apodization Window.vi"("error in (no error)"=w56, "Processing in"=w51) -> ("error out"=w55:errorcluster, "Apodization Window"=w57:T22, "Processing out"=w59:refnum<class "Processing.lvclass">)  [unwired: 1 in]
      n73 = call "set Apodization Window.vi"("error in (no error)"=w55, "Window"=w57, "Processing"=w59) -> ("error out"=w54:errorcluster, "Processing"=w58:refnum<class "Processing.lvclass">)  [unwired: 3 in]
      n74 = call "set Processing Flag.vi"("error in (no error)"=w54, "Flag"=w60, "Processing Flag Selection"=Processing_Flag_Selection."Use Extended Adjust", "Processing"=w58) -> ("error out"=w50:errorcluster, "Processing"=w62:refnum<class "Processing.lvclass">)  [unwired: 2 in]
      "Processing" <- w62
      n75 = call "create Coloring.vi"("Color Byte Order"=Coloring_Byteorder."RGBA32", "Color Table Selection"=Colorscheme_Selection."Black And White") -> ("Coloring"=w81:refnum<class "Coloring.lvclass">)  [unwired: 4 in, 1 out]
      n76 = local write "Window"(w57) -> ()
      n77 = call "set Device Preset.vi"("Numeric"=0, "error in (no error)"=w50, "Probe"=w44, "Processing"=w51, "OCTDevice"=w46) -> ()  [unwired: 1 in, 4 out]
      "SLDIndicator" <- w48
    }
    frame #2 {
      n78 = while "Programmloop" {
        tunnel: w115 -> [w905]
        tunnel: [w907] -> w114
        tunnel: w113 -> [w906]
        stop <- "QuitApp" stop-if-true
        n79 = case shown="True" "Start Measurement" {
          tunnel: w905 -> [w909 w912]
          tunnel: [w909 w910] -> w907
          tunnel: w906 -> [_ w911]
          frame False {
          }
          frame True {
            n80 = while "Measure" {
              tunnel: w912 -> [w914]
              tunnel: w911 -> [w975]
              tunnel: [w948] -> w910
              stop <- w1019 continue-if-true
              w964 = 150 ("index")
              # "Contrast"
              # "AScan"
              # "After Apo"
              # "After Offset"
              # "Spectrum"
              n81 = call "set Processing Parameter Int.vi"("Value"="Binning", "Processing Paramter Int Selection"=Processing_Parameter_Int_Selection."Spectrum Averaging", "Processing in"=w975) -> ("error out"=w971:errorcluster, "Processing out"=w974:refnum<class "Processing.lvclass">)  [unwired: 3 in]
              n82 = call "create Data.vi"() -> ("Data"=w1013:refnum<class "Data.lvclass">)  [unwired: 6 in, 1 out]
              n83 = call "create Data.vi"() -> ("Data"=w984:refnum<class "Data.lvclass">)  [unwired: 6 in, 1 out]
              n84 = call "create Data.vi"() -> ("Data"=w982:refnum<class "Data.lvclass">)  [unwired: 6 in, 1 out]
              n85 = call "create Data.vi"() -> ("Data"=w978:refnum<class "Data.lvclass">)  [unwired: 6 in, 1 out]
              n86 = call "set Processing Parameter Int.vi"("error in (no error)"=w971, "Value"="Averaging", "Processing Paramter Int Selection"=Processing_Parameter_Int_Selection."A-Scan Averaging", "Processing in"=w974) -> ("error out"=w970:errorcluster, "Processing out"=w973:refnum<class "Processing.lvclass">)  [unwired: 2 in]
              n87 = Multiply(x="Binning", y="Averaging") -> (x*y=w967:i32)
              n88 = call "create Raw Data.vi"() -> ("error out"=w1014:errorcluster, "Raw Data"=w1018:refnum<class "Raw Data.lvclass">)  [unwired: 6 in]
              n89 = call-poly "set Processing Output.vi"("error in (no error)"=w970, "Data"=w1013, "Processing"=w973) -> ("error out"=w985:errorcluster, "Data"=w1011:refnum<class "Data.lvclass">)  [unwired: 2 in, 1 out]
              n90 = call-poly "set Processing Output.vi"("error in (no error)"=w985, "Data"=w984, "Processing"=w973) -> ("error out"=w981:errorcluster, "Data"=w983:refnum<class "Data.lvclass">)  [unwired: 2 in, 1 out]
              n91 = call-poly "set Processing Output.vi"("error in (no error)"=w981, "Data"=w982, "Processing"=w973) -> ("error out"=w980:errorcluster, "Data"=w977:refnum<class "Data.lvclass">)  [unwired: 2 in, 1 out]
              n92 = call-poly "set Processing Output.vi"("error in (no error)"=w980, "Data"=w978, "Processing"=w973) -> ("error out"=w936:errorcluster, "Data"=w979:refnum<class "Data.lvclass">)  [unwired: 2 in, 1 out]
              n93 = call "measure Spectra.vi"("Camera #"="Camera #", "error in (no error)"=w1014, "NumberOfSpectra"=w967, "Raw Data"=w1018, "OCTDevice"=w914) -> ("error out"=w937:errorcluster, "Raw Data"=w1017:refnum<class "Raw Data.lvclass">, "OCTDevice"=w949:refnum<class "OCT Device.lvclass">)  [unwired: 1 in]
              n94 = control-ref of="Spectrum"() -> (w1016:refnum<vi>)
              n95 = control-ref of="SpectrumWithOffsetRemoved"() -> (w1015:refnum<vi>)
              n96 = control-ref of="Apodized Spectrum"() -> (w1008:refnum<vi>)
              n97 = control-ref of="AScan"() -> (w1007:refnum<vi>)
              n98 = Merge Errors(w937, w936) -> (w935:errorcluster)
              n99 = call "execute Processing.vi"("error in (no error)"=w935, "Raw Data"=w1017, "Processing"=w973) -> ("error out"=w1010:errorcluster, "Raw Data"=w1012:refnum<class "Raw Data.lvclass">)  [unwired: 2 in, 1 out]
              n100 = call "clear Raw Data.vi"("Raw Data"=w1012) -> ()  [unwired: 6 in, 1 out]
              n101 = call-poly "display Data.vi"("error in (no error)"=w1010, "Data in"=w1011, "WFGraph Refnum"=w1016) -> ("error out"=w1006:errorcluster, "Data out"=w1009:refnum<class "Data.lvclass">)  [unwired: 2 in, 1 out]
              n102 = call-poly "display Data.vi"("error in (no error)"=w1010, "Data in"=w983, "WFGraph Refnum"=w1015) -> ("error out"=w946:errorcluster, "Data out"=w947:refnum<class "Data.lvclass">, "Data Content"=w951:sgl[])  [unwired: 2 in]
              n103 = call-poly "display Data.vi"("error in (no error)"=w1010, "Data in"=w977, "WFGraph Refnum"=w1008) -> ("error out"=w933:errorcluster, "Data out"=w1005:refnum<class "Data.lvclass">)  [unwired: 2 in, 1 out]
              n104 = call-poly "display Data.vi"("error in (no error)"=w1010, "Data in"=w979, "WFGraph Refnum"=w1007) -> ("Data out"=w925:refnum<class "Data.lvclass">)  [unwired: 2 in, 2 out]
              n105 = call "clear Data.vi"("error in (no error)"=w1006, "Data"=w1009) -> ()  [unwired: 5 in, 1 out]
              n106 = call "create Data.vi"() -> ("error out"=w934:errorcluster, "Data"=w1004:refnum<class "Data.lvclass">)  [unwired: 6 in]
              n107 = control-ref of="Contrast"() -> (w1000:refnum<vi>)
              n108 = Divide(x="Power in Spectrometer [µW]", y=1000000.0) -> (x/y=w942:dbl)
              n109 = call "calc Interference Contrast.vi"("error in (no error)"=w934, "Contrast Handle"=w1004, "Apodized Spectrum Handle"=w1005) -> ("error out"=w998:errorcluster, "Contrast Handle"=w1001:refnum<class "Data.lvclass">, "Apodized Spectrum Handle"=w999:refnum<class "Data.lvclass">)
              n110 = call-poly <vilib>:"RMS.vi"("X"=w951) -> ("rms value"=→"RMS":dbl)  [unwired: 1 out]
              n111 = call-poly "display Data.vi"("error in (no error)"=w998, "Data in"=w1001, "WFGraph Refnum"=w1000) -> ("error out"=w1003:errorcluster, "Data out"=w1002:refnum<class "Data.lvclass">, "Data Content"=w966:sgl[])  [unwired: 2 in]
              n112 = call "Quantum Efficiency.vi"("Data in (Spectrum [e-])"=w947, "error in (no error)"=w946, "Power into Spectrometer [W]"=w942, "Center Wavelength [nm]"="Center Wavelength [nm]", "OCT Device in"=w949) -> ("error out"=w945:errorcluster, "Quantum Efficiency"=w940:dbl, "OCT Device out"=w948:refnum<class "OCT Device.lvclass">)  [unwired: 1 in, 1 out]
              n113 = call "analyze Data.vi"("error in (no error)"=w945, "Data Analyzation Selection"=Data_Analyzation_Selection."Min", "Data"=w947) -> ("error out"=w988:errorcluster, "Property Value"=→"Min Intensity":dbl, "Data out"=w986:refnum<class "Data.lvclass">)  [unwired: 2 in]
              n114 = call "analyze Data.vi"("error in (no error)"=w988, "Data Analyzation Selection"=Data_Analyzation_Selection."Max", "Data"=w947) -> ("error out"=w987:errorcluster, "Property Value"=→"Max Intensity":dbl)  [unwired: 2 in, 1 out]
              n115 = call "clear Data.vi"("error in (no error)"=w933, "Data"=w999) -> ()  [unwired: 5 in, 1 out]
              n116 = call "clear Data.vi"("error in (no error)"=w1003, "Data"=w1002) -> ()  [unwired: 5 in, 1 out]
              n117 = Array Size(array=w966) -> (size(s)=w965:i32)
              n118 = Multiply(x=100.0, y=w940) -> (x*y=→"Quantum eff. [%]":dbl)
              n119 = Subtract(x=w965, y=w964) -> (x-y=w963:i32)
              n120 = Array Subset(array=w966, index=w964, length=w963) -> (w962:sgl[])
              n121 = call "clear Data.vi"("error in (no error)"=w987, "Data"=w986) -> ("error out"=w932:errorcluster)  [unwired: 5 in]
              n122 = Array Max & Min(array=w962) -> (min value=→"Min Contrast [%]":sgl)  [unwired: 3 out]
              n123 = call-poly <vilib>:"Mean.vi"("X"=w962) -> ("mean"=→"Mean Contrast [%]":dbl)  [unwired: 1 out]
              n124 = call <vilib>:"Simple Error Handler.vi"("error in (no error)"=w932) -> ("error?"=w931:bool)  [unwired: 4 in, 4 out]
              n125 = case shown="True" w931 {
                frame False {
                }
                frame True {
                  n126 = local write "Start Measurement"(FALSE ("Start Measurement")) -> ()
                }
              }
              n127 = call "analyze A-Scan.vi"("AScan Analysis Selection"=A-Scan_Analysis_Selection."Noise [dB]", "Data"=w925) -> ("Property Value"=→"Noise [dB]":dbl, "Data out"=w924:refnum<class "Data.lvclass">)  [unwired: 3 in, 1 out]
              n128 = call "analyze A-Scan.vi"("AScan Analysis Selection"=A-Scan_Analysis_Selection."Noise [e-]", "Data"=w924) -> ("Property Value"=→"Noise [e]":dbl, "Data out"=w930:refnum<class "Data.lvclass">)  [unwired: 3 in, 1 out]
              n129 = call "analyze A-Scan.vi"("AScan Analysis Selection"=A-Scan_Analysis_Selection."Peak Pos [Pixel]", "Data"=w930) -> ("Property Value"=w993:dbl, "Data out"=w929:refnum<class "Data.lvclass">)  [unwired: 3 in, 1 out]
              "Peak Pos. [Pixel]" <- w993
              n130 = call "analyze A-Scan.vi"("AScan Analysis Selection"=A-Scan_Analysis_Selection."Peak Height [dB]", "Data"=w929) -> ("Property Value"=→"Peak [dB]":dbl, "Data out"=w928:refnum<class "Data.lvclass">)  [unwired: 3 in, 1 out]
              n131 = call "analyze A-Scan.vi"("AScan Analysis Selection"=A-Scan_Analysis_Selection."Peak Width -6dB [Pixel]", "Data"=w928) -> ("Property Value"=w958:dbl, "Data out"=w927:refnum<class "Data.lvclass">)  [unwired: 3 in, 1 out]
              n132 = call "analyze A-Scan.vi"("AScan Analysis Selection"=A-Scan_Analysis_Selection."Peak Width -20dB [Pixel]", "Data"=w927) -> ("Property Value"=w956:dbl, "Data out"=w926:refnum<class "Data.lvclass">)  [unwired: 3 in, 1 out]
              n133 = call "analyze A-Scan.vi"("AScan Analysis Selection"=A-Scan_Analysis_Selection."Peak Width -40 dB [Pixel]", "Data"=w926) -> ("Property Value"=w996:dbl, "Data out"=w915:refnum<class "Data.lvclass">)  [unwired: 3 in, 1 out]
              n134 = local read "Spacing Z [mm]"() -> (w953:dbl)
              n135 = call "clear Data.vi"("Data"=w915) -> ()  [unwired: 6 in, 1 out]
              n136 = Multiply(x=w953, y=1000.0) -> (x*y=w954:dbl)
              n137 = case shown="True" "z-Calibration" {
                tunnel: w993 -> [_ w1024]
                frame False {
                }
                frame True {
                  n138 = Divide(x="Thickness Sample", y=w1024) -> (x/y=w1026:dbl)
                  n139 = local write "Spacing Z [mm]"(w1026) -> ()
                }
              }
              n140 = local read "Start Measurement"() -> (w1021:bool)
              n141 = local read "QuitApp"() -> (w1022:bool)
              n142 = Multiply(x=w958, y=w954) -> (x*y=→"-6 dB [µm]":dbl)
              n143 = Multiply(x=w956, y=w954) -> (x*y=→"-20 dB [µm]":dbl)
              n144 = Multiply(x=w996, y=w954) -> (x*y=→"-40 dB [µm]":dbl)
              n145 = Not(x=w1022) -> (.not. x?=w1020:bool)
              n146 = Compound Arithmetic op=AND(w1021, w1020) -> (w1019:bool)
            }
          }
        }
        "Meas. Indicator" <- "Start Measurement"
      }
      n147 = while {
        tunnel: w112 -> [w121]
        tunnel: w111 -> [w120]
        tunnel: w110 -> [w116]
        stop <- w119 stop-if-true
        n148 = case shown="\"Signals\", Default" "Tab Control" {
          tunnel: [1000 0 5 0] -> w117
          frame "Signals", Default {
          }
          frame "SLD" {
          }
          frame "Galvo Calibration" {
          }
          frame "Misc." {
          }
        }
        n149 = event shown="[24] \"Calibrate Surface\": Value Change" {
          selector: _ -> [_ _ _ _ _ _ _ _ _ _ _ _ _ _ _ _ _ _ _ _ _ _ _ _ _ _ _ _ _ _ _ _]
          dyn-events: _ -> [_ _ _ _ _ _ _ _ _ _ _ _ _ _ _ _ _ _ _ _ _ _ _ _ _ _ _ _ _ _ _ _]
          timeout: w117 -> [_ _ _ _ _ _ _ _ _ _ _ _ _ _ _ _ _ _ _ _ _ _ _ _ _ _ _ _ _ _ _ _]
          tunnel: w121 -> [w127 w145 w178 _ w219 w273 _ w276 w285 _ w351 _ _ _ w370 _ w378 w447 _ _ _ w506 w686 _ w792 _ w865 w870 _ _ w895 w903]
          tunnel: w120 -> [_ _ _ _ _ _ _ _ w284 w327 w350 w360 w365 _ w369 w376 _ _ _ _ _ w505 w687 _ w791 _ _ w869 _ _ w894 _]
          tunnel: w116 -> [_ _ _ _ _ _ _ _ _ _ _ _ _ _ _ _ _ _ _ w449 _ _ _ _ _ _ _ _ _ _ _ _]
          event Timeout {
            n150 = event-data() -> ()  [unwired: 1 in, 1 out]
            n151 = local read "Tab Control"() -> (w126:T1)
            n152 = case shown="\"Misc.\"" w126 {
              tunnel: w127 -> [_ w128 w142]
              frame "Signals", Default {
              }
              frame "SLD" {
                n153 = property on="Select ADC 2" class="Ring (strict)"() -> ("RingText.Text"=w134:string)  [unwired: 2 in, 2 out]
                n154 = property on="Select ADC 1" class="Ring (strict)"() -> ("RingText.Text"=w136:string)  [unwired: 2 in, 2 out]
                n155 = property on="Select ADC 3" class="Ring (strict)"() -> ("RingText.Text"=w133:string)  [unwired: 2 in, 2 out]
                n156 = call "get Internal Device Parameter by Name.vi"("Identifier"=w136, "OCTDevice"=w128) -> ("error out"=w130:errorcluster, "Result"=→"ADC 1":dbl)  [unwired: 3 in, 1 out]
                n157 = call "get Internal Device Parameter by Name.vi"("error in (no error)"=w130, "Identifier"=w134, "OCTDevice"=w128) -> ("error out"=w129:errorcluster, "Result"=→"ADC 2":dbl)  [unwired: 2 in, 1 out]
                n158 = call "get Internal Device Parameter by Name.vi"("error in (no error)"=w129, "Identifier"=w133, "OCTDevice"=w128) -> ("Result"=→"ADC 3":dbl)  [unwired: 2 in, 2 out]
              }
              frame "Misc." {
                w137 = T23 0 items=["no dialog", "OK message", "continue or stop message", "OK message + warnings", "continue/stop + warnings"] ("type of dialog (OK msg:1)")
                n159 = local read "Colored Data"() -> (w141:refnum<class "Colored Data.lvclass">)
                n160 = call "get Camera Image.vi"("Colored Data in"=w141, "OCTDevice in"=w142) -> ("error out"=w144:errorcluster, "Colored Data out"=w143:refnum<class "Colored Data.lvclass">)  [unwired: 5 in, 1 out]
                n161 = local read "Image"() -> (w140:T3)
                n162 = call "update Colored Data IMAQ Image.vi"("error in (no error)"=w144, "Image in"=w140, "Colored Data"=w143) -> ("error out"=w138:errorcluster, "Image out"=w139:T3)  [unwired: 2 in, 1 out]
                n163 = local write "Image"(w139) -> ()
                n164 = call <vilib>:"Simple Error Handler.vi"("type of dialog (OK msg:1)"=w137, "error in (no error)"=w138) -> ()  [unwired: 3 in, 5 out]
              }
            }
          }
          event "Log Button": Value Change {
            n165 = event-data() -> ()  [unwired: 1 in, 1 out]
            n166 = case shown="True" "Log Button" {
              tunnel: w145 -> [_ w154]
              frame False {
              }
              frame True {
                n167 = call "File Dialog"() -> ("selected path"=w155:path)  [unwired: 12 in, 3 out]
                n168 = call "get Internal Device Parameters.vi"("OCTDevice"=w154) -> ("ADCs"=w149:string[], "OCTDevice"=w147:refnum<class "OCT Device.lvclass">)  [unwired: 3 in, 2 out]
                n169 = for {
                  tunnel: [w157] -> w148 mode=indexing
                  tunnel: w149 -> [w158] mode=indexing
                  n170 = call <vilib>:"Space Constant.vi"() -> ("String"=w156:string)
                  n171 = Concatenate Strings(w158, w156) -> (w157:string)
                }
                n172 = Concatenate Strings("Date Time Milliseconds " ("string"), w148, "\r") -> (w152:string)
                n173 = Write to Text File(file (use dialog)=w155, text=w152) -> (refnum out=w153:refnum<file>)  [unwired: 2 in, 2 out]
                n174 = while {
                  tunnel: w147 -> [w171]
                  tunnel: w149 -> [w172]
                  tunnel: w153 -> [w170]
                  stop <- w173 continue-if-true
                  n175 = for {
                    tunnel: w172 -> [w176] mode=indexing
                    tunnel: w171 -> [w175]
                    tunnel: w170 -> [_]
                    tunnel: [w174] -> w165 mode=indexing
                    n176 = call "get Internal Device Parameter by Name.vi"("Identifier"=w176, "OCTDevice"=w175) -> ("Result"=w174:dbl)  [unwired: 3 in, 2 out]
                  }
                  n177 = Wait For Front Panel Activity(1:15000 ("timeout ms (-1 never timeout)")) -> (0:w167:u32)  [unwired: 2 in]
                  n178 = Number To Decimal String(number=w167) -> (decimal integer string=w166:string)  [unwired: 1 in]
                  n179 = call <vilib>:"Space Constant.vi"() -> ("String"=w159:string)
                  n180 = Array To Spreadsheet String(delimiter (Tab)=w159, array=w165, 3:"%f" ("format string")) -> (spreadsheet string=w161:string)
                  n181 = Format Date/Time String() -> (date/time string=w163:string)  [unwired: 3 in]
                  n182 = call <vilib>:"Space Constant.vi"() -> ("String"=w160:string)
                  n183 = call <vilib>:"Space Constant.vi"() -> ("String"=w162:string)
                  n184 = local read "Log Button"() -> (w173:bool)
                  n185 = Concatenate Strings(w163, w162, w166, w160, w161) -> (w169:string)
                  n186 = Write to Text File(file (use dialog)=w170, text=w169) -> ()  [unwired: 2 in, 3 out]
                }
              }
            }
          }
          event "Ring Light Intensity [%]": Value Change {
            n187 = event-data() -> ()  [unwired: 1 in, 5 out]
            n188 = call "set Output Device Value by Name.vi"("Value"="Ring Light Intensity [%]", "Identifier"="ring light", "OCTDevice"=w178) -> ()  [unwired: 3 in, 2 out]
          }
          event "Save calibration": Value Change {
            n189 = event-data() -> ()  [unwired: 1 in, 5 out]
            n190 = case shown="True" "Save calibration" {
              frame False {
              }
              frame True {
                n191 = local read "Probe"() -> (w199:refnum<class "Probe.lvclass">)
                n192 = local read "FactorY"() -> (w188:sgl)
                n193 = local read "OffsetY"() -> (w190:sgl)
                n194 = local read "FactorX"() -> (w189:sgl)
                n195 = local read "OffsetX"() -> (w191:sgl)
                n196 = call "set Probe Parameter Float.vi"("Value"=w189, "Probe Parameter Float"=Probe_Parameter_Float_Selection."Factor X", "Probe"=w199) -> ("error out"=w207:errorcluster, "Probe"=w198:refnum<class "Probe.lvclass">)  [unwired: 3 in]
                n197 = call "set Probe Parameter Float.vi"("error in (no error)"=w207, "Value"=w188, "Probe Parameter Float"=Probe_Parameter_Float_Selection."Factor Y", "Probe"=w199) -> ("error out"=w206:errorcluster, "Probe"=w197:refnum<class "Probe.lvclass">)  [unwired: 2 in]
                n198 = call "set Probe Parameter Float.vi"("error in (no error)"=w206, "Value"=w191, "Probe Parameter Float"=Probe_Parameter_Float_Selection."Offset X", "Probe"=w199) -> ("error out"=w205:errorcluster, "Probe"=w196:refnum<class "Probe.lvclass">)  [unwired: 2 in]
                n199 = call "set Probe Parameter Float.vi"("error in (no error)"=w205, "Value"=w190, "Probe Parameter Float"=Probe_Parameter_Float_Selection."Offset Y", "Probe"=w199) -> ("error out"=w204:errorcluster, "Probe"=w195:refnum<class "Probe.lvclass">)  [unwired: 2 in]
                n200 = local read "Camera Scaling Y"() -> (w186:sgl)
                n201 = local read "Camera Scaling X"() -> (w187:sgl)
                n202 = local read "Camera Offset X"() -> (w185:sgl)
                n203 = local read "Camera Offset Y"() -> (w184:sgl)
                n204 = call "set Probe Parameter Float.vi"("error in (no error)"=w204, "Value"=w187, "Probe Parameter Float"=Probe_Parameter_Float_Selection."Camera Scaling X", "Probe"=w198) -> ("error out"=w203:errorcluster, "Probe"=w193:refnum<class "Probe.lvclass">)  [unwired: 2 in]
                n205 = call "set Probe Parameter Float.vi"("error in (no error)"=w203, "Value"=w186, "Probe Parameter Float"=Probe_Parameter_Float_Selection."Camera Scaling Y", "Probe"=w197) -> ("error out"=w202:errorcluster)  [unwired: 2 in, 1 out]
                n206 = call "set Probe Parameter Float.vi"("error in (no error)"=w202, "Value"=w185, "Probe Parameter Float"=Probe_Parameter_Float_Selection."Camera Offset X", "Probe"=w196) -> ("error out"=w201:errorcluster)  [unwired: 2 in, 1 out]
                n207 = call "set Probe Parameter Float.vi"("error in (no error)"=w201, "Value"=w184, "Probe Parameter Float"=Probe_Parameter_Float_Selection."Camera Offset Y", "Probe"=w195) -> ("error out"=w200:errorcluster)  [unwired: 2 in, 1 out]
                n208 = local read "Camera Angle"() -> (w182:sgl)
                n209 = call "set Probe Parameter Float.vi"("error in (no error)"=w200, "Value"=w182, "Probe Parameter Float"=Probe_Parameter_Float_Selection."Angle", "Probe"=w193) -> ("error out"=w216:errorcluster, "Probe"=w192:refnum<class "Probe.lvclass">)  [unwired: 2 in]
                n210 = call "save Probe.vi"("error in (no error)"=w216, "Name"="Probe", "Probe in"=w192) -> ("error out"=w183:errorcluster)  [unwired: 3 in, 1 out]
                n211 = call <vilib>:"Simple Error Handler.vi"("error in (no error)"=w183) -> ()  [unwired: 4 in, 5 out]
              }
            }
            n212 = local write "Save calibration"(FALSE ("Save calibration")) -> ()
          }
          event "Scan Benchmark": Value Change {
            n213 = event-data() -> ()  [unwired: 1 in, 1 out]
            n214 = local read "Scan Benchmark"() -> (w218:bool)
            n215 = case shown="True" w218 {
              tunnel: w219 -> [_ w249]
              frame False {
              }
              frame True {
                w233 = 1024 ("AScans")
                w234 = 2.0 ("Range")
                n216 = local read "Probe"() -> (w232:refnum<class "Probe.lvclass">)
                n217 = Divide(x="Angle [°]", y=180.0) -> (x/y=w239:dbl)
                n218 = call "create B-Scan Pattern.vi"("AScans"=w233, "Range"=w234, "Probe"=w232) -> ("error out"=w220:errorcluster, "Scan Pattern"=w242:refnum<class "Scan Pattern.lvclass">)  [unwired: 3 in, 1 out]
                n219 = call "create Ideal B-Scan Pattern.vi"("AScans"=w233, "Range"=w234, "Probe"=w232) -> ("error out"=w231:errorcluster, "Scan Pattern"=w230:refnum<class "Scan Pattern.lvclass">)  [unwired: 2 in, 1 out]
                n220 = Multiply(x=3.141592653589793, y=w239) -> (x*y=w229:dbl)
                n221 = call "rotate Scan Pattern.vi"("error in (no error)"=w220, "Angle"=w229, "ScanPattern"=w242) -> ("error out"=w221:errorcluster, "ScanPattern"=w241:refnum<class "Scan Pattern.lvclass">)  [unwired: 3 in]
                n222 = call "rotate Scan Pattern.vi"("error in (no error)"=w231, "Angle"=w229, "ScanPattern"=w230) -> ("error out"=w222:errorcluster, "ScanPattern"=w228:refnum<class "Scan Pattern.lvclass">)  [unwired: 3 in]
                n223 = call "get Scan Pattern LUT.vi"("error in (no error)"=w221, "Scan Pattern in"=w241) -> ("error out"=w243:errorcluster, "Values Y (mm)"=w247:dbl[], "Values X (mm)"=w248:dbl[], "Scan Pattern out"=w244:refnum<class "Scan Pattern.lvclass">)  [unwired: 2 in]
                n224 = Reciprocal(x="Scan Rate [Hz]") -> (1/x=w235:dbl)
                n225 = call "get Scan Pattern LUT.vi"("error in (no error)"=w222, "Scan Pattern in"=w228) -> ("Values Y (mm)"=w225:dbl[], "Values X (mm)"=w226:dbl[], "Scan Pattern out"=w227:refnum<class "Scan Pattern.lvclass">)  [unwired: 2 in, 1 out]
                n226 = call "clear Scan Pattern.vi"("error in (no error)"=w243, "Scan Pattern in"=w244) -> ()  [unwired: 5 in, 1 out]
                n227 = property on="X" class="WFGraph (strict)"("XScale.Multiplier"=w235) -> ()  [unwired: 2 in, 2 out]
                n228 = property on="Y" class="WFGraph (strict)"("XScale.Multiplier"=w235) -> ()  [unwired: 2 in, 2 out]
                n229 = call "clear Scan Pattern.vi"("Scan Pattern in"=w227) -> ()  [unwired: 6 in, 1 out]
                n230 = call "start Scan Benchmark.vi"("Rate Hz"="Scan Rate [Hz]", "error in (no error)"=w243, "Raw Y"=w247, "Raw X"=w248, "OCT Device in"=w249) -> ("error out"=w224:errorcluster, "OCT Device out"=w246:refnum<class "OCT Device.lvclass">)  [unwired: 3 in]
                n231 = while {
                  tunnel: w248 -> [w266]
                  tunnel: w247 -> [w262]
                  tunnel: w226 -> [w260]
                  tunnel: w225 -> [w259]
                  tunnel: w224 -> [w258]
                  tunnel: [w257] -> w223
                  shift-right: [w264] -> w245
                  shift-left: w246 -> [w268]
                  stop <- w250 continue-if-true
                  n232 = call "get Scan Feedback.vi"("error in (no error)"=w258, "OCT Device in"=w268) -> ("error out"=w257:errorcluster, "Values Y"=w263:dbl[], "Values X"=w267:dbl[], "OCT Device out"=w264:refnum<class "OCT Device.lvclass">)  [unwired: 2 in]
                  n233 = Build Array(w267, w266, w260) -> (→"X":dbl[][])
                  n234 = Build Array(w263, w262, w259) -> (→"Y":dbl[][])
                  n235 = local read "Tab Control"() -> (w253:T1)
                  n236 = local read "QuitApp"() -> (w255:bool)
                  n237 = Equal?(x=w253, y=T1."Galvo") -> (x = y?=w251:bool)
                  n238 = Not(x=w255) -> (.not. x?=w254:bool)
                  n239 = Compound Arithmetic op=AND(w251, w254, "Scan Benchmark") -> (w250:bool)
                }
                n240 = call "stop Scan Benchmark.vi"("error in (no error)"=w223, "OCT Device in"=w245) -> ()  [unwired: 4 in, 2 out]
              }
            }
          }
          event "Spectrum": Cursor Move {
            n241 = event-data() -> ()  [unwired: 1 in, 1 out]
            n242 = property on="Spectrum" class="WFGraph (strict)"() -> ("Cursor.Cursor X"=w272:dbl)  [unwired: 2 in, 2 out]
            n243 = call "get Wavelength at Pixel.vi"("Pixel"=w272, "OCTDevice"=w273) -> ("Wavelength [nm]"=w271:dbl)  [unwired: 3 in, 2 out]
            n244 = Multiply(x=w271, y=1000000000.0) -> (x*y=→"Selected Wavelength [nm]":dbl)
          }
          event "Clear All": Value Change {
            n245 = event-data() -> ()  [unwired: 1 in, 5 out]
            n246 = case shown="True" "Clear All" {
              frame False {
              }
              frame True {
                w275 = dbl[] [] ("History Data")
                n247 = property on="ADC 1" class="WFChart (strict)"("History Data"=w275) -> ()  [unwired: 2 in, 2 out]
                n248 = property on="ADC 2" class="WFChart (strict)"("History Data"=w275) -> ()  [unwired: 2 in, 2 out]
                n249 = property on="ADC 3" class="WFChart (strict)"("History Data"=w275) -> ()  [unwired: 2 in, 2 out]
              }
            }
          }
          event "Select ADC 1", "Select ADC 2", "Select ADC 3": Value Change {
            n250 = event-data() -> ()  [unwired: 1 in, 1 out]
            n251 = local read "Select ADC 1"() -> (w278:u16)
            n252 = local read "Select ADC 2"() -> (w279:u16)
            n253 = local read "Select ADC 3"() -> (w280:u16)
            n254 = call "get Internal Device Parameter Units.vi"("OCTDevice"=w276) -> ("Units"=w277:string[])  [unwired: 3 in, 3 out]
            n255 = Index Array(array=w277, index #1=w278, index #2=w279, index #3=w280) -> (element #1=w281:string, element #2=w282:string, element #3=w283:string)
            n256 = property on="ADC 1" class="WFChart (strict)"("YScale.NameLbl.Text"=w281, "YScale.UnitLabel.Text"=w281) -> ()  [unwired: 2 in, 2 out]
            n257 = property on="ADC 2" class="WFChart (strict)"("YScale.NameLbl.Text"=w282, "YScale.UnitLabel.Text"=w282) -> ()  [unwired: 2 in, 2 out]
            n258 = property on="ADC 3" class="WFChart (strict)"("YScale.NameLbl.Text"=w283, "YScale.UnitLabel.Text"=w283) -> ()  [unwired: 2 in, 2 out]
          }
          event "LambdaToKLab", "LambdaToKMisc": Value Change {
            n259 = event-data() -> ()  [unwired: 1 in, 1 out]
            n260 = Or(x="LambdaToKMisc", y="LambdaToKLab") -> (x .or. y?=w288:bool)
            n261 = case shown="True" w288 {
              tunnel: w285 -> [_ w290]
              tunnel: w284 -> [_ w289]
              frame False {
              }
              frame True {
                n262 = flat-sequence {
                  tunnel: w290 -> [w301]
                  tunnel: w289 -> [w302]
                  frame #0 {
                    n263 = local read "Camera #"() -> (w291:i32)
                    n264 = call "measure Calibration.vi"("Camera Index"=w291, "Calibration Data"=Calibration_Selection."Chirp", "Processing"=w302, "OCTDevice"=w301) -> ("Processing"=w299:refnum<class "Processing.lvclass">)  [unwired: 2 in, 2 out]
                    n265 = call "create Data.vi"() -> ("Data"=w298:refnum<class "Data.lvclass">)  [unwired: 6 in, 1 out]
                    n266 = control-ref of="Chirp"() -> (w295:refnum<vi>)
                    n267 = call "get Calibration.vi"("Calibration Data"=Calibration_Selection."Chirp", "Data"=w298, "Processing"=w299) -> ("error out"=w297:errorcluster, "Data"=w296:refnum<class "Data.lvclass">)  [unwired: 2 in, 1 out]
                    n268 = call-poly "display Data.vi"("error in (no error)"=w297, "Data in"=w296, "WFGraph Refnum"=w295) -> ("error out"=w292:errorcluster, "Data out"=w294:refnum<class "Data.lvclass">)  [unwired: 2 in, 1 out]
                    n269 = call "clear Data.vi"("error in (no error)"=w292, "Data"=w294) -> ()  [unwired: 5 in, 1 out]
                  }
                  frame #1 {
                    w304 = FALSE ("DeChirp")
                    n270 = local write "LambdaToKMisc"(w304) -> ()
                    n271 = local write "LambdaToKLab"(w304) -> ()
                    n272 = local write "Save Dechirp"(FALSE ("Save Calibration")) -> ()
                  }
                }
              }
            }
          }
          event "Offset Error", "Dechirp", "Apodization", "Extended", "Dispersion Comp.", "Filter Undersampl.", "Remove DC Spectrum", "FullRange": Value Change {
            n273 = event-data() -> ()  [unwired: 1 in, 6 out]
            n274 = call "set Processing Flag.vi"("Flag"="Offset Error", "Processing Flag Selection"=Processing_Flag_Selection."Use Offset Errors", "Processing"=w327) -> ("Processing"=w309:refnum<class "Processing.lvclass">)  [unwired: 3 in, 1 out]
            n275 = case shown="\"True\"" "Remove DC Spectrum" {
              tunnel: w309 -> [w334 w341 w348]
              tunnel: [w330 w337 w344] -> w308
              frame "False", Default {
                n276 = call "set Processing Flag.vi"("Flag"=FALSE, "Processing Flag Selection"=Processing_Flag_Selection."Remove DC Spectrum", "Processing"=w334) -> ("Processing"=w333:refnum<class "Processing.lvclass">)  [unwired: 3 in, 1 out]
                n277 = call "set Processing Flag.vi"("Flag"=FALSE, "Processing Flag Selection"=Processing_Flag_Selection."Remove Advanced DC Spectrum", "Processing"=w333) -> ("Processing"=w330:refnum<class "Processing.lvclass">)  [unwired: 3 in, 1 out]
              }
              frame "True" {
                n278 = call "set Processing Flag.vi"("Flag"=TRUE, "Processing Flag Selection"=Processing_Flag_Selection."Remove DC Spectrum", "Processing"=w341) -> ("Processing"=w340:refnum<class "Processing.lvclass">)  [unwired: 3 in, 1 out]
                n279 = call "set Processing Flag.vi"("Flag"=TRUE, "Processing Flag Selection"=Processing_Flag_Selection."Remove Advanced DC Spectrum", "Processing"=w340) -> ("Processing"=w337:refnum<class "Processing.lvclass">)  [unwired: 3 in, 1 out]
              }
              frame "Mixed" {
                n280 = call "set Processing Flag.vi"("Flag"=TRUE, "Processing Flag Selection"=Processing_Flag_Selection."Remove DC Spectrum", "Processing"=w348) -> ("Processing"=w347:refnum<class "Processing.lvclass">)  [unwired: 3 in, 1 out]
                n281 = call "set Processing Flag.vi"("Flag"=FALSE, "Processing Flag Selection"=Processing_Flag_Selection."Remove Advanced DC Spectrum", "Processing"=w347) -> ("Processing"=w344:refnum<class "Processing.lvclass">)  [unwired: 3 in, 1 out]
              }
            }
            n282 = call "set Processing Flag.vi"("Flag"="Apodization", "Processing Flag Selection"=Processing_Flag_Selection."Use Apodization", "Processing"=w308) -> ("Processing"=w313:refnum<class "Processing.lvclass">)  [unwired: 3 in, 1 out]
            n283 = call "set Processing Flag.vi"("Flag"="Filter Undersampl.", "Processing Flag Selection"=Processing_Flag_Selection."Filter Undersampled Signals", "Processing"=w313) -> ("Processing"=w314:refnum<class "Processing.lvclass">)  [unwired: 3 in, 1 out]
            n284 = call "set Processing Flag.vi"("Flag"="Dechirp", "Processing Flag Selection"=Processing_Flag_Selection."Use Dechirp", "Processing"=w314) -> ("Processing"=w326:refnum<class "Processing.lvclass">)  [unwired: 3 in, 1 out]
            n285 = call "set Processing Flag.vi"("Flag"="Extended", "Processing Flag Selection"=Processing_Flag_Selection."Use Extended Adjust", "Processing"=w326) -> ("Processing"=w316:refnum<class "Processing.lvclass">)  [unwired: 3 in, 1 out]
            n286 = call "set Processing Flag.vi"("Flag"="Dispersion Comp.", "Processing Flag Selection"=Processing_Flag_Selection."Use Dispersion Compensation", "Processing"=w316) -> ("Processing"=w307:refnum<class "Processing.lvclass">)  [unwired: 3 in, 1 out]
            n287 = call "set Processing Flag.vi"("Flag"="FullRange", "Processing Flag Selection"=Processing_Flag_Selection."Full Range Output", "Processing"=w307) -> ()  [unwired: 3 in, 2 out]
          }
          event "Repeated LambdaToK": Value Change {
            n288 = event-data() -> ()  [unwired: 1 in, 1 out]
            n289 = case shown="True" "Repeated LambdaToK" {
              tunnel: w351 -> [_ w353]
              tunnel: w350 -> [_ w352]
              frame False {
              }
              frame True {
                n290 = while {
                  tunnel: w353 -> [_]
                  tunnel: w352 -> [_]
                  stop <- w356 continue-if-true
                  (unwired) FALSE ("Ask?")
                  n291 = local read "Repeated LambdaToK"() -> (w355:bool)
                  n292 = local read "Tab Control"() -> (w358:T1)
                  n293 = Equal?(x=w358, y=T14."Misc.") -> (x = y?=w354:bool)
                  n294 = And(x=w355, y=w354) -> (x .and. y?=w356:bool)
                }
              }
            }
          }
          event "Save Dechirp": Value Change {
            n295 = event-data() -> ()  [unwired: 1 in, 1 out]
            n296 = case shown="False" "Save Dechirp" {
              tunnel: w360 -> [_ w363]
              frame False {
                n297 = local write "Save Dechirp"(TRUE ("Save Calibration")) -> ()
              }
              frame True {
                n298 = call "save Calibration Default.vi"("Calibration Data"=Calibration_Selection."Chirp", "Processing"=w363) -> ()  [unwired: 4 in, 2 out]
              }
            }
          }
          event "Save Dispersion": Value Change {
            n299 = event-data() -> ()  [unwired: 1 in, 1 out]
            n300 = case shown="False" "Save Dispersion" {
              tunnel: w365 -> [_ w368]
              frame False {
                n301 = local write "Save Dispersion"(TRUE ("Save Calibration")) -> ()
              }
              frame True {
                n302 = call "save Calibration Default.vi"("Calibration Data"=Calibration_Selection."Dispersion", "Processing"=w368) -> ()  [unwired: 4 in, 2 out]
              }
            }
          }
          event "Zero Padding", "Spacing Z [mm]": Value Change {
            n303 = event-data() -> ()  [unwired: 1 in, 6 out]
          }
          event "Apodization": Value Change {
            n304 = event-data() -> ()  [unwired: 1 in, 1 out]
            n305 = case shown="True" "Apodization" {
              tunnel: w370 -> [_ w375]
              tunnel: w369 -> [_ w374]
              frame False {
              }
              frame True {
                n306 = local read "Camera #"() -> (w372:i32)
                n307 = call "measure Calibration.vi"("Camera Index"=w372, "Calibration Data"=Calibration_Selection."Apodization Vector", "Processing"=w374, "OCTDevice"=w375) -> ()  [unwired: 2 in, 3 out]
              }
            }
          }
          event "Window": Value Change {
            n308 = event-data() -> ()  [unwired: 1 in, 1 out]
            n309 = call "set Apodization Window.vi"("Window"="Window", "Processing"=w376) -> ()  [unwired: 4 in, 2 out]
          }
          event "Load.ini": Value Change {
            n310 = event-data() -> ("NewVal"=w380:bool)  [unwired: 1 in]
            n311 = local read "Probe"() -> (w379:refnum<class "Probe.lvclass">)
            n312 = case shown="True" w380 {
              tunnel: w379 -> [_ w400]
              tunnel: w378 -> [_ w391]
              frame False {
              }
              frame True {
                n313 = call "close Probe.vi"("GalvoControl"=w400) -> ("error out"=w383:errorcluster)  [unwired: 6 in]
                n314 = local read "System"() -> (w402:enum16{"Probe", "Handheld", "Microscope"})
                n315 = case shown="\"Microscope\"" w402 {
                  tunnel: ["Probe" ("filename") "HandHeld" ("filename") "Microscope" ("filename")] -> w399
                  tunnel: w383 -> [_ _ _]
                  frame "Probe", Default {
                  }
                  frame "Handheld" {
                  }
                  frame "Microscope" {
                  }
                }
                n316 = call "init Probe.vi"("Probe"=w399, "OCT Device"=w391) -> ("error out"=w381:errorcluster, "GalvoControl"=w390:refnum<class "Probe.lvclass">)  [unwired: 4 in]
                n317 = call "get Probe Parameter Float.vi"("error in (no error)"=w381, "Probe Parameter Float"=Probe_Parameter_Float_Selection."Factor X", "GalvoControl"=w390) -> ("Value"=w401:dbl)  [unwired: 2 in, 2 out]
                n318 = call "get Probe Parameter Float.vi"("error in (no error)"=w381, "Probe Parameter Float"=Probe_Parameter_Float_Selection."Offset X", "GalvoControl"=w390) -> ("Value"=w397:dbl)  [unwired: 2 in, 2 out]
                n319 = call "get Probe Parameter Float.vi"("error in (no error)"=w381, "Probe Parameter Float"=Probe_Parameter_Float_Selection."Factor Y", "GalvoControl"=w390) -> ("Value"=w392:dbl)  [unwired: 2 in, 2 out]
                n320 = call "get Probe Parameter Float.vi"("error in (no error)"=w381, "Probe Parameter Float"=Probe_Parameter_Float_Selection."Offset Y", "GalvoControl"=w390) -> ("Value"=w393:dbl)  [unwired: 2 in, 2 out]
                n321 = call "get Probe Parameter Float.vi"("error in (no error)"=w381, "Probe Parameter Float"=Probe_Parameter_Float_Selection."Flyback Time [s]", "GalvoControl"=w390) -> ("Value"=w386:dbl)  [unwired: 2 in, 2 out]
                n322 = call "get Probe Parameter Float.vi"("error in (no error)"=w381, "Probe Parameter Float"=Probe_Parameter_Float_Selection."Rotation Time [s]", "GalvoControl"=w390) -> ("Value"=w385:dbl)  [unwired: 2 in, 2 out]
                n323 = call "get Probe Parameter Float.vi"("error in (no error)"=w381, "Probe Parameter Float"=Probe_Parameter_Float_Selection."Expansion Time [s]", "GalvoControl"=w390) -> ("Value"=w384:dbl, "GalvoControl"=w382:refnum<class "Probe.lvclass">)  [unwired: 2 in, 1 out]
                n324 = local write "Calibration Factor X [V/mm]"(w401) -> ()
                n325 = local write "Offset X [V]"(w397) -> ()
                n326 = local write "Calibration Factor Y [V/mm]"(w392) -> ()
                n327 = local write "Offset Y [V]"(w393) -> ()
                n328 = local write "Flyback Time [s]"(w386) -> ()
                n329 = local write "Rotation Time [s]"(w385) -> ()
                n330 = local write "Expansion Time [s]"(w384) -> ()
                n331 = local write "Probe"(w382) -> ()
              }
            }
          }
          event "Set Position X [mm]", "Set Position Y [mm]", "Offset X [V]", "Offset Y [V]", "Calibration Factor X [V/mm]", "Calibration Factor Y [V/mm]", "Flyback Time [s]", "Rotation Time [s]", "Expansion Time [s]", "Scan Rate [Hz]": Value Change {
            w427 = u16 1 items=["X-Achse", "Y-Achse"] ("Achse")
            w431 = u16 0 items=["X-Achse", "Y-Achse"] ("Achse")
            n332 = event-data() -> ()  [unwired: 1 in, 6 out]
            n333 = property on="Tab Control" class="TabCtl (strict)" props=["Wert"]() -> ()  [unwired: 2 in, 3 out]
            n334 = local read "Scan Rate [Hz]"() -> (w411:dbl)
            n335 = local read "Probe"() -> (w407:refnum<class "Probe.lvclass">)
            n336 = call "set Probe Parameter Float.vi"("Value"=w411, "Probe Parameter Float"=Probe_Parameter_Float_Selection."Expected Scan Rate [Hz]", "Probe"=w407) -> ("error out"=w409:errorcluster, "Probe"=w408:refnum<class "Probe.lvclass">)  [unwired: 3 in]
            n337 = call "set Probe Parameter Float.vi"("error in (no error)"=w409, "Value"="Calibration Factor X [V/mm]", "Probe Parameter Float"=Probe_Parameter_Float_Selection."Factor X", "Probe"=w408) -> ("error out"=w435:errorcluster, "Probe"=w444:refnum<class "Probe.lvclass">)  [unwired: 2 in]
            n338 = call "set Probe Parameter Float.vi"("error in (no error)"=w435, "Value"="Offset X [V]", "Probe Parameter Float"=Probe_Parameter_Float_Selection."Offset X", "Probe"=w444) -> ("error out"=w434:errorcluster, "Probe"=w441:refnum<class "Probe.lvclass">)  [unwired: 2 in]
            n339 = call "set Probe Parameter Float.vi"("error in (no error)"=w434, "Value"="Calibration Factor Y [V/mm]", "Probe Parameter Float"=Probe_Parameter_Float_Selection."Factor Y", "Probe"=w441) -> ("error out"=w433:errorcluster, "Probe"=w438:refnum<class "Probe.lvclass">)  [unwired: 2 in]
            n340 = call "set Probe Parameter Float.vi"("error in (no error)"=w433, "Value"="Offset Y [V]", "Probe Parameter Float"=Probe_Parameter_Float_Selection."Offset Y", "Probe"=w438) -> ("error out"=w424:errorcluster, "Probe"=w432:refnum<class "Probe.lvclass">)  [unwired: 2 in]
            n341 = call "move Scanner.vi"("Axis"=w431, "error in (no error)"=w424, "Position"="Set Position X [mm]", "GalvoControl"=w432, "OCTDevice"=w447) -> ("error out"=w425:errorcluster, "GalvoControl"=w429:refnum<class "Probe.lvclass">, "OCTDevice"=w428:refnum<class "OCT Device.lvclass">)  [unwired: 2 in]
            n342 = call "move Scanner.vi"("Axis"=w427, "error in (no error)"=w425, "Position"="Set Position Y [mm]", "GalvoControl"=w429, "OCTDevice"=w428) -> ("error out"=w420:errorcluster, "GalvoControl"=w423:refnum<class "Probe.lvclass">)  [unwired: 2 in, 1 out]
            n343 = call "set Probe Parameter Float.vi"("error in (no error)"=w420, "Value"="Flyback Time [s]", "Probe Parameter Float"=Probe_Parameter_Float_Selection."Flyback Time [s]", "Probe"=w423) -> ("error out"=w418:errorcluster, "Probe"=w419:refnum<class "Probe.lvclass">)  [unwired: 2 in]
            n344 = call "set Probe Parameter Float.vi"("error in (no error)"=w418, "Value"="Rotation Time [s]", "Probe Parameter Float"=Probe_Parameter_Float_Selection."Rotation Time [s]", "Probe"=w419) -> ("error out"=w412:errorcluster, "Probe"=w415:refnum<class "Probe.lvclass">)  [unwired: 2 in]
            n345 = call "set Probe Parameter Float.vi"("error in (no error)"=w412, "Value"="Expansion Time [s]", "Probe Parameter Float"=Probe_Parameter_Float_Selection."Expansion Time [s]", "Probe"=w415) -> ("error out"=w406:errorcluster)  [unwired: 2 in, 1 out]
            n346 = call <vilib>:"Simple Error Handler.vi"("error in (no error)"=w406) -> ()  [unwired: 4 in, 5 out]
          }
          event "Write Config": Value Change {
            n347 = event-data() -> ()  [unwired: 1 in, 6 out]
            n348 = case shown="True" "Write Config" {
              frame False {
              }
              frame True {
                n349 = call "copy Config to Device.vi"() -> ()  [unwired: 12 in]
              }
            }
          }
          event "Show Scan", "Scaling [px/mm]", "Rotation [deg]", "Scan Contrast", "Offset Y", "Offset X", "dB": Value Change {
            n350 = event-data() -> ()  [unwired: 1 in, 1 out]
            n351 = local read "Show Scan"() -> (w450:bool)
            n352 = local read "En face"() -> (w453:refnum<class "Data.lvclass">)
            n353 = call "is Data valid.vi"("Data"=w453) -> ("valid?"=w452:bool)
            n354 = And(x=w452, y=w450) -> (x .and. y?=w451:bool)
            n355 = case shown="True" w451 {
              tunnel: w449 -> [_ w473]
              frame False {
              }
              frame True {
                n356 = local read "Probe"() -> (w488:refnum<class "Probe.lvclass">)
                n357 = local read "Scaling [px/mm]"() -> (w483:sgl)
                n358 = call "set Probe Parameter Float.vi"("Value"=w483, "Probe Parameter Float"=Probe_Parameter_Float_Selection."Camera Scaling X", "Probe"=w488) -> ("error out"=w485:errorcluster, "Probe"=w486:refnum<class "Probe.lvclass">)  [unwired: 3 in]
                n359 = call "set Probe Parameter Float.vi"("error in (no error)"=w485, "Value"=w483, "Probe Parameter Float"=Probe_Parameter_Float_Selection."Camera Scaling Y", "Probe"=w486) -> ("error out"=w479:errorcluster, "Probe"=w482:refnum<class "Probe.lvclass">)  [unwired: 2 in]
                n360 = local read "Offset X"() -> (w480:i32)
                n361 = call "set Probe Parameter Float.vi"("error in (no error)"=w479, "Value"=w480, "Probe Parameter Float"=Probe_Parameter_Float_Selection."Camera Offset X", "Probe"=w482) -> ("error out"=w478:errorcluster, "Probe"=w477:refnum<class "Probe.lvclass">)  [unwired: 2 in]
                n362 = local read "Offset Y"() -> (w475:i32)
                n363 = call "set Probe Parameter Float.vi"("error in (no error)"=w478, "Value"=w475, "Probe Parameter Float"=Probe_Parameter_Float_Selection."Camera Offset Y", "Probe"=w477) -> ("error out"=w455:errorcluster, "Probe"=w458:refnum<class "Probe.lvclass">)  [unwired: 2 in]
                n364 = local read "Rotation [deg]"() -> (w454:sgl)
                n365 = local read "En face"() -> (w463:refnum<class "Data.lvclass">)
                n366 = Unbundle("dB") -> (w466:sgl, w465:sgl)
                n367 = call "create Colored Data.vi"() -> ("Colored Data"=w471:refnum<class "Colored Data.lvclass">)  [unwired: 6 in, 1 out]
                n368 = call "set Coloring Boundaries.vi"("Danymic Range High [dB]"=w465, "Dynamic Range Low [dB]"=w466, "Coloring in"=w473) -> ("Coloring out"=w472:refnum<class "Coloring.lvclass">)  [unwired: 3 in, 1 out]
                n369 = call "set Probe Parameter Float.vi"("error in (no error)"=w455, "Value"=w454, "Probe Parameter Float"=Probe_Parameter_Float_Selection."Angle", "Probe"=w458) -> ("Probe"=w457:refnum<class "Probe.lvclass">)  [unwired: 2 in, 1 out]
                n370 = local read "Camera Image"() -> (w462:refnum<class "Colored Data.lvclass">)
                n371 = call "colorize Data.vi"("Colored Data"=w471, "Data"=w463, "Coloring in"=w472) -> ("Colored Data"=w470:refnum<class "Colored Data.lvclass">)  [unwired: 1 in, 3 out]
                n372 = call "create Colored Data.vi"() -> ("Colored Data"=w461:refnum<class "Colored Data.lvclass">)  [unwired: 6 in, 1 out]
                n373 = call "copy Colored Data.vi"("ColoredData Destination"=w461, "ColoredData Source"=w462) -> ("ColoredData Destination"=w459:refnum<class "Colored Data.lvclass">)  [unwired: 3 in, 2 out]
                n374 = local read "Scan Contrast"() -> (w464:sgl)
                n375 = disable-structure shown="Enabled" {
                  disable-tunnel: w470 -> [w489 w493 w496]
                  disable-tunnel: w457 -> [_ _ _]
                  disable-tunnel: _ -> [_ w494 w495]
                  disable-tunnel: [_ w494 w496] -> w469
                  disable-tunnel: w464 -> [_ _ _]
                  disable-tunnel: w459 -> [_ _ _]
                  frame Enabled {
                    (unwired) FALSE ("Dense View")
                    n376 = local read "OverlayImage 2"() -> (w491:T3)
                    n377 = call "update Colored Data IMAQ Image.vi"("Image in"=w491, "Colored Data"=w489) -> ("Image out"=w490:T3, "Colored Data"=w492:refnum<class "Colored Data.lvclass">)  [unwired: 3 in, 1 out]
                    n378 = local write "OverlayImage 2"(w490) -> ()
                    n379 = call "clear Colored Data.vi"("Colored Data"=w492) -> ()  [unwired: 6 in, 1 out]
                  }
                  frame Disabled {
                    n380 = call "clear Colored Data.vi"("Colored Data"=w493) -> ()  [unwired: 1 in, 1 out]
                  }
                  frame Disabled {
                    n381 = call "clear Colored Data.vi"("Colored Data"=w495) -> ()  [unwired: 1 in, 1 out]
                  }
                }
                n382 = local read "OverlayImage"() -> (w468:T3)
                n383 = call "update Colored Data IMAQ Image.vi"("Image in"=w468, "Colored Data"=w469) -> ("Image out"=w467:T3, "Colored Data"=w460:refnum<class "Colored Data.lvclass">)  [unwired: 3 in, 1 out]
                n384 = local write "OverlayImage"(w467) -> ()
                n385 = call "clear Colored Data.vi"("Colored Data"=w460) -> ()  [unwired: 6 in, 1 out]
              }
            }
          }
          event "Save Handheld": Value Change {
            n386 = event-data() -> ()  [unwired: 1 in, 6 out]
            n387 = case shown="True" "Save Handheld" {
              frame False {
              }
              frame True {
                n388 = case shown="\"Probe\"" "Probe" {
                  tunnel: ["Probe" ("filename") "HandHeld" ("filename") "Microscope" ("filename")] -> w498
                  frame "Probe" {
                  }
                  frame "Handheld", Default {
                  }
                  frame "Microscope" {
                  }
                }
                n389 = local read "Probe"() -> (w500:refnum<class "Probe.lvclass">)
                n390 = call "save Probe.vi"("Name"=w498, "Probe in"=w500) -> ()  [unwired: 4 in, 2 out]
              }
            }
          }
          event "Dispersion": Value Change {
            n391 = event-data() -> ()  [unwired: 1 in, 1 out]
            n392 = case shown="True" "Dispersion" {
              tunnel: w506 -> [_ w508]
              tunnel: w505 -> [_ w540]
              tunnel: 50 ("Value") -> [_ w525]
              frame False {
              }
              frame True {
                n393 = call "create Raw Data.vi"() -> ("error out"=w541:errorcluster, "Raw Data"=w542:refnum<class "Raw Data.lvclass">)  [unwired: 6 in]
                n394 = flat-sequence {
                  tunnel: w540 -> [w553]
                  tunnel: w541 -> [w554]
                  tunnel: w542 -> [w555]
                  tunnel: [w543] -> w520
                  tunnel: [w555] -> w518
                  tunnel: [w554] -> w516
                  tunnel: [w553] -> w514
                  tunnel: w525 -> [w546]
                  tunnel: [w546] -> w512
                  tunnel: [w544] -> w510
                  tunnel: w508 -> [w543]
                  tunnel: w520 -> [w561]
                  tunnel: [w561] -> w519
                  tunnel: w518 -> [w560]
                  tunnel: [w560] -> w517
                  tunnel: w516 -> [w559]
                  tunnel: [w559] -> w515
                  tunnel: w514 -> [w558]
                  tunnel: [w558] -> w513
                  tunnel: w512 -> [w557]
                  tunnel: [w557] -> w511
                  tunnel: w510 -> [w556]
                  tunnel: [w556] -> w509
                  tunnel: [w579] -> w527
                  tunnel: w519 -> [w572]
                  tunnel: w517 -> [w581]
                  tunnel: w515 -> [w578]
                  tunnel: w513 -> [w575]
                  tunnel: w511 -> [w574]
                  tunnel: [w580] -> w524
                  tunnel: [w577] -> w523
                  tunnel: [w576] -> w522
                  tunnel: w509 -> [w569]
                  tunnel: [w616] -> w538
                  tunnel: [w615] -> w536
                  tunnel: [w614] -> w534
                  tunnel: [w611] -> w532
                  tunnel: [w613] -> w531
                  tunnel: w527 -> [w621]
                  tunnel: w524 -> [w604]
                  tunnel: w523 -> [w610]
                  tunnel: w522 -> [w611]
                  tunnel: [w603] -> w521
                  tunnel: [w628] -> w539
                  tunnel: w538 -> [w632]
                  tunnel: [w630] -> w537
                  tunnel: w536 -> [w635]
                  tunnel: [w627] -> w535
                  tunnel: w534 -> [w633]
                  tunnel: [w629] -> w533
                  tunnel: w532 -> [w634]
                  tunnel: w531 -> [w631]
                  tunnel: [w631] -> w526
                  tunnel: w521 -> [w624]
                  tunnel: w539 -> [w664]
                  tunnel: w537 -> [w663]
                  tunnel: w535 -> [w661]
                  tunnel: w533 -> [w660]
                  tunnel: [w654] -> w530
                  tunnel: [w656] -> w529
                  tunnel: [w655] -> w528
                  tunnel: w526 -> [w654]
                  tunnel: w530 -> [w684]
                  tunnel: w529 -> [w683]
                  tunnel: w528 -> [w673]
                  frame #0 {
                    n395 = local write "Start Measurement"(FALSE ("Start Measurement")) -> ()
                    n396 = local write "Tmp"(FALSE ("Tmp")) -> ()
                    n397 = call "get Device Property Float.vi"("Device Property Float Selection"=Device_Property_Float_Selection."z Range", "OCTDevice"=w543) -> ("Value"=w550:dbl)  [unwired: 3 in, 2 out]
                    n398 = Multiply(x=w550, y=0.2) -> (x*y=w547:dbl)
                    n399 = Number To Fractional String(number=w547, precision (6)=i16 2) -> (F-format string=w544:string)  [unwired: 2 in]
                  }
                  frame #1 {
                    n400 = while {
                      stop <- w562 continue-if-true
                      n401 = local read "Meas. Indicator"() -> (w562:bool)
                    }
                  }
                  frame #2 {
                    n402 = call "set Processing Parameter Int.vi"("Value"=w574, "Processing Paramter Int Selection"=Processing_Parameter_Int_Selection."Spectrum Averaging", "Processing in"=w575) -> ("Processing out"=w566:refnum<class "Processing.lvclass">)  [unwired: 3 in, 1 out]
                    n403 = call "set Processing Parameter Int.vi"("Value"=1, "Processing Paramter Int Selection"=Processing_Parameter_Int_Selection."A-Scan Averaging", "Processing in"=w566) -> ("Processing out"=w563:refnum<class "Processing.lvclass">)  [unwired: 3 in, 1 out]
                    n404 = while {
                      tunnel: w572 -> [w601]
                      tunnel: w563 -> [w600]
                      tunnel: [w595] -> w580
                      tunnel: [w586] -> w576
                      tunnel: [w594] -> w579
                      tunnel: [w593] -> w577
                      tunnel: w581 -> [w587]
                      tunnel: w574 -> [w586]
                      tunnel: w578 -> [w585]
                      stop <- w596 stop-if-true
                      n405 = call "create Data.vi"() -> ("Data"=w599:refnum<class "Data.lvclass">)  [unwired: 6 in, 1 out]
                      n406 = call "measure Spectra.vi"("Camera #"=0, "error in (no error)"=w585, "NumberOfSpectra"=w586, "Raw Data"=w587, "OCTDevice"=w601) -> ("error out"=w584:errorcluster, "Raw Data"=w597:refnum<class "Raw Data.lvclass">, "OCTDevice"=w595:refnum<class "OCT Device.lvclass">)  [unwired: 1 in]
                      n407 = control-ref of="AScan"() -> (w588:refnum<vi>)
                      n408 = call-poly "set Processing Output.vi"("error in (no error)"=w584, "Data"=w599, "Processing"=w600) -> ("error out"=w583:errorcluster, "Data"=w591:refnum<class "Data.lvclass">, "Processing"=w598:refnum<class "Processing.lvclass">)  [unwired: 2 in]
                      n409 = call "execute Processing.vi"("error in (no error)"=w583, "Raw Data"=w597, "Processing"=w598) -> ("error out"=w589:errorcluster, "Raw Data"=w594:refnum<class "Raw Data.lvclass">, "Processing"=w593:refnum<class "Processing.lvclass">)  [unwired: 2 in]
                      n410 = local read "Tmp"() -> (w596:bool)
                      n411 = call-poly "display Data.vi"("error in (no error)"=w589, "Data in"=w591, "WFGraph Refnum"=w588) -> ("error out"=w592:errorcluster, "Data out"=w590:refnum<class "Data.lvclass">)  [unwired: 2 in, 1 out]
                      n412 = call "clear Data.vi"("error in (no error)"=w592, "Data"=w590) -> ()  [unwired: 5 in, 1 out]
                    }
                    n413 = Concatenate Strings("Determining Dispersion\ncompensation will also set\nyour Chirp to a dispersion \nindependent version.\n\nPlease move the signal peak\nto approx. position " ("message"), w569, " mm and press \"Okay\"." ("string")) -> (w567:string)
                    n414 = One Button Dialog(message=w567) -> (true=w571:bool)  [unwired: 1 in]
                    n415 = local write "Tmp"(w571) -> ()
                  }
                  frame #3 {
                    n416 = call "create Data.vi"() -> ("Data"=w620:refnum<class "Data.lvclass">)  [unwired: 6 in, 1 out]
                    n417 = call "measure Spectra.vi"("Camera #"=0, "NumberOfSpectra"=w611, "Raw Data"=w621, "OCTDevice"=w604) -> ("Raw Data"=w618:refnum<class "Raw Data.lvclass">, "OCTDevice"=w615:refnum<class "OCT Device.lvclass">)  [unwired: 2 in, 1 out]
                    n418 = call-poly "set Processing Output.vi"("Data"=w620, "Processing"=w610) -> ("error out"=w617:errorcluster, "Data"=w613:refnum<class "Data.lvclass">, "Processing"=w619:refnum<class "Processing.lvclass">)  [unwired: 3 in]
                    n419 = call "get Device Property Float.vi"("Device Property Float Selection"=Device_Property_Float_Selection."z Range", "OCTDevice"=w604) -> ("Value"=w606:dbl)  [unwired: 3 in, 2 out]
                    n420 = Multiply(x=w606, y=0.3) -> (x*y=w609:dbl)
                    n421 = local write "Tmp"(FALSE ("Tmp")) -> ()
                    n422 = Number To Fractional String(number=w609, precision (6)=i16 2) -> (F-format string=w603:string)  [unwired: 2 in]
                    n423 = call "execute Processing.vi"("error in (no error)"=w617, "Raw Data"=w618, "Processing"=w619) -> ("Raw Data"=w616:refnum<class "Raw Data.lvclass">, "Processing"=w614:refnum<class "Processing.lvclass">)  [unwired: 2 in, 1 out]
                  }
                  frame #4 {
                    n424 = while {
                      tunnel: w635 -> [w652]
                      tunnel: w634 -> [w644]
                      tunnel: w633 -> [w651]
                      tunnel: w632 -> [w648]
                      tunnel: [w645] -> w630
                      tunnel: [w644] -> w629
                      tunnel: [w643] -> w628
                      tunnel: [w642] -> w627
                      stop <- w646 stop-if-true
                      n425 = call "create Data.vi"() -> ("Data"=w650:refnum<class "Data.lvclass">)  [unwired: 6 in, 1 out]
                      n426 = call "measure Spectra.vi"("Camera #"=0, "NumberOfSpectra"=w644, "Raw Data"=w648, "OCTDevice"=w652) -> ("Raw Data"=w647:refnum<class "Raw Data.lvclass">, "OCTDevice"=w645:refnum<class "OCT Device.lvclass">)  [unwired: 2 in, 1 out]
                      n427 = control-ref of="AScan"() -> (w637:refnum<vi>)
                      n428 = call-poly "set Processing Output.vi"("Data"=w650, "Processing"=w651) -> ("Data"=w640:refnum<class "Data.lvclass">, "Processing"=w649:refnum<class "Processing.lvclass">)  [unwired: 3 in, 1 out]
                      n429 = call "execute Processing.vi"("Raw Data"=w647, "Processing"=w649) -> ("error out"=w638:errorcluster, "Raw Data"=w643:refnum<class "Raw Data.lvclass">, "Processing"=w642:refnum<class "Processing.lvclass">)  [unwired: 3 in]
                      n430 = local read "Tmp"() -> (w646:bool)
                      n431 = call-poly "display Data.vi"("error in (no error)"=w638, "Data in"=w640, "WFGraph Refnum"=w637) -> ("error out"=w641:errorcluster, "Data out"=w639:refnum<class "Data.lvclass">)  [unwired: 2 in, 1 out]
                      n432 = call "clear Data.vi"("error in (no error)"=w641, "Data"=w639) -> ()  [unwired: 5 in, 1 out]
                    }
                    n433 = Concatenate Strings("Please move the sample \nmirror to approx. position " ("message"), w624, " mm and press \"Okay\"." ("string")) -> (w623:string)
                    n434 = One Button Dialog(message=w623) -> (true=→"Tmp":bool)  [unwired: 1 in]
                  }
                  frame #5 {
                    n435 = call "create Data.vi"() -> ("Data"=w662:refnum<class "Data.lvclass">)  [unwired: 6 in, 1 out]
                    n436 = call "measure Spectra.vi"("Camera #"=0, "NumberOfSpectra"=w660, "Raw Data"=w664, "OCTDevice"=w663) -> ("Raw Data"=w658:refnum<class "Raw Data.lvclass">)  [unwired: 2 in, 2 out]
                    n437 = call-poly "set Processing Output.vi"("Data"=w662, "Processing"=w661) -> ("Data"=w656:refnum<class "Data.lvclass">, "Processing"=w659:refnum<class "Processing.lvclass">)  [unwired: 3 in, 1 out]
                    n438 = call "execute Processing.vi"("Raw Data"=w658, "Processing"=w659) -> ("Raw Data"=w657:refnum<class "Raw Data.lvclass">, "Processing"=w655:refnum<class "Processing.lvclass">)  [unwired: 3 in, 1 out]
                    n439 = call "clear Raw Data.vi"("Raw Data"=w657) -> ()  [unwired: 6 in, 1 out]
                  }
                  frame #6 {
                    w665 = FALSE ("Save Calibration")
                    n440 = call "create Data.vi"() -> ("Data"=w674:refnum<class "Data.lvclass">)  [unwired: 6 in, 1 out]
                    n441 = call "create Data.vi"() -> ("Data"=w681:refnum<class "Data.lvclass">)  [unwired: 6 in, 1 out]
                    n442 = call "compute Dispersion.vi"("Dispersion"=w674, "Chirp"=w681, "Apodized Spectrum 2"=w683, "Apodized Spectrum 1"=w684) -> ("Dispersion"=w672:refnum<class "Data.lvclass">, "Chirp"=w682:refnum<class "Data.lvclass">, "Apodized Spectrum 2"=w679:refnum<class "Data.lvclass">, "Apodized Spectrum 1"=w680:refnum<class "Data.lvclass">)
                    n443 = local write "Save Dispersion"(w665) -> ()
                    n444 = local write "Save Dechirp"(w665) -> ()
                    n445 = control-ref of="Dispersion"() -> (w668:refnum<vi>)
                    n446 = call "set Calibration.vi"("Calibration Data"=Calibration_Selection."Chirp", "Data"=w682, "Processing"=w673) -> ("Data"=w677:refnum<class "Data.lvclass">)  [unwired: 2 in, 2 out]
                    n447 = call "set Calibration.vi"("Calibration Data"=Calibration_Selection."Dispersion", "Data"=w672, "Processing"=w673) -> ("Data"=w669:refnum<class "Data.lvclass">)  [unwired: 2 in, 2 out]
                    n448 = call "clear Data.vi"("Data"=w680) -> ()  [unwired: 6 in, 1 out]
                    n449 = call "clear Data.vi"("Data"=w679) -> ()  [unwired: 6 in, 1 out]
                    n450 = control-ref of="Chirp"() -> (w678:refnum<vi>)
                    n451 = call-poly "display Data.vi"("Data in"=w677, "WFGraph Refnum"=w678) -> ("error out"=w676:errorcluster, "Data out"=w675:refnum<class "Data.lvclass">)  [unwired: 3 in, 1 out]
                    n452 = call-poly "display Data.vi"("Data in"=w669, "WFGraph Refnum"=w668) -> ("error out"=w667:errorcluster, "Data out"=w666:refnum<class "Data.lvclass">)  [unwired: 3 in, 1 out]
                    n453 = call "clear Data.vi"("error in (no error)"=w667, "Data"=w666) -> ()  [unwired: 5 in, 1 out]
                    n454 = call "clear Data.vi"("error in (no error)"=w676, "Data"=w675) -> ()  [unwired: 5 in, 1 out]
                  }
                }
              }
            }
          }
          event "Scan": Value Change {
            n455 = event-data() -> ()  [unwired: 1 in, 2 out]
            n456 = case shown="True" "Scan" {
              tunnel: w687 -> [_ w692]
              tunnel: w686 -> [_ w698]
              frame False {
              }
              frame True {
                w697 = T24."Disabled and Grayed Out" ("Disabled")
                n457 = property on="Scans X" class="DigNum (strict)"("DisabledEnum"=w697) -> ()  [unwired: 2 in, 2 out]
                n458 = property on="Scans Y" class="DigNum (strict)"("DisabledEnum"=w697) -> ()  [unwired: 2 in, 2 out]
                n459 = property on="Range X [mm]" class="DigNum (strict)"("DisabledEnum"=w697) -> ()  [unwired: 2 in, 2 out]
                n460 = property on="Range Y [mm]" class="DigNum (strict)"("DisabledEnum"=w697) -> ()  [unwired: 2 in, 2 out]
                n461 = property on="Scan" class="Bool (strict)"("DisabledEnum"=w697) -> ()  [unwired: 2 in, 2 out]
                n462 = flat-sequence {
                  tunnel: w698 -> [w709]
                  tunnel: [w711] -> w696
                  tunnel: [w707] -> w695
                  tunnel: [w706] -> w694
                  tunnel: [w705] -> w693
                  tunnel: w692 -> [w704]
                  tunnel: [w704] -> w691
                  tunnel: w696 -> [w723]
                  tunnel: w695 -> [w719]
                  tunnel: w694 -> [w725]
                  tunnel: w693 -> [w722]
                  tunnel: w691 -> [w724]
                  tunnel: [w721] -> w690
                  tunnel: [w720] -> w689
                  tunnel: [w717] -> w688
                  tunnel: w690 -> [w751]
                  tunnel: w689 -> [w752]
                  tunnel: w688 -> [w753]
                  frame #0 {
                    n463 = local read "Scans Y"() -> (w707:i32)
                    n464 = local read "Volume"() -> (w702:refnum<class "Data.lvclass">)
                    n465 = local read "Range X [mm]"() -> (w713:dbl)
                    n466 = local read "Range Y [mm]"() -> (w712:dbl)
                    n467 = local read "Probe"() -> (w714:refnum<class "Probe.lvclass">)
                    n468 = local read "Scans X"() -> (w703:i32)
                    n469 = call "clear Data.vi"("Data"=w702) -> ()  [unwired: 6 in, 1 out]
                    n470 = call "create Data.vi"() -> ("Data"=w710:refnum<class "Data.lvclass">)  [unwired: 6 in, 1 out]
                    n471 = call "get Device Property Int.vi"("Device Property Int Selection"=Device_Property_Int_Selection."Spectrum Elements", "OCTDevice"=w709) -> ("Value"=w708:i32, "OCTDevice"=w705:refnum<class "OCT Device.lvclass">)  [unwired: 3 in, 1 out]
                    n472 = call "create B-Scan Stack Pattern.vi"("Size Y"=w707, "Size X"=w703, "Range Y"=w712, "Range X"=w713, "Probe"=w714) -> ("Scan Pattern"=w711:refnum<class "Scan Pattern.lvclass">)  [unwired: 2 in, 2 out]
                    n473 = Divide(x=w708, y=2) -> (x/y=w701:dbl)
                    n474 = call "reserve Data.vi"("Size 3"=w707, "Size 2"=w703, "Size 1"=w701, "Data in"=w710) -> ("Data out"=w706:refnum<class "Data.lvclass">)  [unwired: 4 in, 1 out]
                  }
                  frame #1 {
                    n475 = local read "Camera Image"() -> (w718:refnum<class "Colored Data.lvclass">)
                    n476 = local read "En face"() -> (w716:refnum<class "Data.lvclass">)
                    n477 = call "start Measurement.vi"("Acquisition Type"=T16."Asynchronous Finite", "Scan Pattern"=w723, "OCTDevice"=w722) -> ("Scan Pattern"=w720:refnum<class "Scan Pattern.lvclass">, "OCTDevice"=w715:refnum<class "OCT Device.lvclass">)  [unwired: 2 in, 1 out]
                    n478 = call "create Data.vi"() -> ("Data"=w729:refnum<class "Data.lvclass">)  [unwired: 6 in, 1 out]
                    n479 = call "clear Data.vi"("Data"=w716) -> ()  [unwired: 6 in, 1 out]
                    n480 = call "create Raw Data.vi"() -> ("error out"=w727:errorcluster, "Raw Data"=w728:refnum<class "Raw Data.lvclass">)  [unwired: 6 in]
                    n481 = call "clear Colored Data.vi"("Colored Data"=w718) -> ()  [unwired: 6 in, 1 out]
                    n482 = for {
                      N: w719 -> [_]
                      tunnel: w727 -> [w744]
                      tunnel: w728 -> [w743]
                      tunnel: w715 -> [w742]
                      tunnel: w729 -> [w741]
                      tunnel: w725 -> [w735]
                      tunnel: [w734] -> w717
                      tunnel: w724 -> [w733]
                      tunnel: [w732] -> w721
                      n483 = call-poly "set Processing Output.vi"("Data"=w741, "Processing"=w733) -> ("Data"=w736:refnum<class "Data.lvclass">, "Processing"=w740:refnum<class "Processing.lvclass">)  [unwired: 3 in, 1 out]
                      n484 = call "get Raw Data.vi"("error in (no error)"=w744, "Camera Index"=0, "RawData in"=w743, "OCTDevice in"=w742) -> ("error out"=w738:errorcluster, "RawData out"=w739:refnum<class "Raw Data.lvclass">, "OCTDevice out"=w732:refnum<class "OCT Device.lvclass">)  [unwired: 1 in]
                      n485 = call "execute Processing.vi"("error in (no error)"=w738, "Raw Data"=w739, "Processing"=w740) -> ("error out"=w731:errorcluster)  [unwired: 2 in, 2 out]
                      n486 = call "append Data.vi"("error in (no error)"=w731, "Normal Direction"=Normal_Direction_Selection."Direction 3", "Data to append in"=w736, "Data in"=w735) -> ("Data out"=w734:refnum<class "Data.lvclass">)  [unwired: 1 in, 2 out]
                    }
                  }
                  frame #2 {
                    # "FIXME: Repeated execution will not clear scan pattern."
                    n487 = disable-structure shown="USE_SURFACE==1, Default" {
                      disable-tunnel: w753 -> [w764 w778]
                      disable-tunnel: [w763 w777] -> w749
                      disable-tunnel: [w759 w773] -> w748
                      disable-tunnel: [w758 w772] -> w746
                      disable-tunnel: [w757 w771] -> w745
                      frame condition #0 {
                        n488 = call "get Data Slice Analyzed.vi"("Normal Direction"=Normal_Direction_Selection."Direction 1", "Data Analyzation Selection"=Data_Analyzation_Selection."Mean", "Data"=w764) -> (2:"Slice"=w760:refnum<class "Data.lvclass">, "Data"=w763:refnum<class "Data.lvclass">, 8:"Slice"=w765:refnum<class "Data.lvclass">)  [unwired: 3 in, 1 out]
                        n489 = call "determine Dynamic Range.vi"("Data in"=w760) -> ("High"=w762:sgl, "Low"=w761:sgl, "Data out"=w759:refnum<class "Data.lvclass">)  [unwired: 3 in, 1 out]
                        n490 = Decrement(x=w761) -> (x-1=w758:sgl)
                        n491 = Increment(x=w762) -> (x+1=w757:sgl)
                      }
                      frame condition #1 (active) {
                        n492 = call "create Data.vi"() -> ("Data"=w770:refnum<class "Data.lvclass">)  [unwired: 6 in, 1 out]
                        n493 = call "determine Surface.vi"("Surface Data in"=w770, "Data in"=w778) -> ("Surface Data out"=w768:refnum<class "Data.lvclass">, "Data out"=w777:refnum<class "Data.lvclass">)  [unwired: 3 in, 1 out]
                        n494 = control-ref of="3D Surface"() -> (w769:refnum<vi>)
                        n495 = call "analyze Data.vi"("Data Analyzation Selection"=Data_Analyzation_Selection."Min", "Data"=w768) -> ("Property Value"=w772:dbl, "Data out"=w775:refnum<class "Data.lvclass">)  [unwired: 3 in, 1 out]
                        n496 = call-poly "display Data.vi"("Data in"=w768, "3D Surface Refnum"=w769) -> ()  [unwired: 3 in, 3 out]
                        n497 = call "analyze Data.vi"("Data Analyzation Selection"=Data_Analyzation_Selection."Max", "Data"=w775) -> ("Property Value"=w771:dbl, "Data out"=w773:refnum<class "Data.lvclass">)  [unwired: 3 in, 1 out]
                      }
                    }
                    "Volume" <- w749
                    "En face" <- w748
                    n498 = call "stop Measurement.vi"("OCTDevice"=w751) -> ("OCTDevice"=w750:refnum<class "OCT Device.lvclass">)  [unwired: 5 in, 1 out]
                    n499 = call "create Colored Data.vi"() -> ("error out"=w756:errorcluster, "Colored Data"=w755:refnum<class "Colored Data.lvclass">)  [unwired: 6 in]
                    n500 = call "get Camera Image.vi"("error in (no error)"=w756, "Colored Data in"=w755, "OCTDevice in"=w750) -> ("Colored Data out"=→"Camera Image":refnum<class "Colored Data.lvclass">)  [unwired: 4 in, 2 out]
                    n501 = Bundle("Property Value"=w746, "Property Value"=w745) -> (w747:T25)  [unwired: 1 in]
                    n502 = local write "dB"(w747) -> ()
                    "Scan Pattern" <- w752
                  }
                  frame #3 {
                    w781 = T24."Enabled" ("Disabled")
                    n503 = local write "Scan"(FALSE ("Scan")) -> ()
                    n504 = property on="Scan" class="Bool (strict)"("DisabledEnum"=w781) -> ()  [unwired: 2 in, 2 out]
                    n505 = property on="Scans X" class="DigNum (strict)"("DisabledEnum"=w781) -> ()  [unwired: 2 in, 2 out]
                    n506 = property on="Scans Y" class="DigNum (strict)"("DisabledEnum"=w781) -> ()  [unwired: 2 in, 2 out]
                    n507 = property on="Range X [mm]" class="DigNum (strict)"("DisabledEnum"=w781) -> ()  [unwired: 2 in, 2 out]
                    n508 = property on="Range Y [mm]" class="DigNum (strict)"("DisabledEnum"=w781) -> ()  [unwired: 2 in, 2 out]
                    n509 = property on="Show Scan" class="Bool (strict)"("DisabledEnum"=w781, "Val(Sgnl)"=TRUE ("Show Scan")) -> ()  [unwired: 2 in, 2 out]
                  }
                }
              }
            }
          }
          event "Tab Control": Value Change {
            n510 = event-data() -> ()  [unwired: 1 in, 6 out]
            n511 = local read "Tab Control"() -> (w784:T1)
            n512 = Not Equal?(x=w784, y=T19."Lab Version") -> (x != y?=w786:bool)
            n513 = Not Equal?(x=w784, y=T1."Galvo") -> (x != y?=w782:bool)
            n514 = case shown="True" w782 {
              frame False {
              }
              frame True {
                n515 = local write "Scan Benchmark"(FALSE ("Scan Benchmark")) -> ()
              }
            }
            n516 = case shown="True" w786 {
              frame False {
              }
              frame True {
                n517 = local write "Start Measurement"(FALSE ("Start\nMeasurement")) -> ()
              }
            }
          }
          event "Calibrate Surface": Value Change {
            n518 = event-data() -> ()  [unwired: 1 in, 1 out]
            n519 = case shown="True" "Calibrate Surface" {
              tunnel: w792 -> [_ w798]
              tunnel: w791 -> [_ w815]
              tunnel: [_ FALSE ("Calibrate Surface")] -> w789
              frame False {
              }
              frame True {
                w799 = TRUE ("Licht an (true) / aus (false)")
                n520 = local read "Probe"() -> (w804:refnum<class "Probe.lvclass">)
                n521 = call "create B-Scan Stack Pattern.vi"("Size Y"="Number Scans Y", "Size X"="Number Scans X", "Range Y"="RangeY [mm]", "Range X"="RangeX [mm]", "Probe"=w804) -> ("Scan Pattern"=w796:refnum<class "Scan Pattern.lvclass">)  [unwired: 2 in, 2 out]
                n522 = local write "SLD"(w799) -> ()
                n523 = local write "SLDIndicator"(w799) -> ()
                n524 = call "set Device Flag.vi"("Boolean"=w799, "Device Property Flag Selection"=T5."SLD Status", "OCTDevice"=w798) -> ("OCTDevice 2"=w797:refnum<class "OCT Device.lvclass">)  [unwired: 7 in, 1 out]
                n525 = call "start Measurement.vi"("Acquisition Type"=T16."Asynchronous Finite", "Scan Pattern"=w796, "OCTDevice"=w797) -> ("OCTDevice"=w816:refnum<class "OCT Device.lvclass">)  [unwired: 2 in, 2 out]
                n526 = call "create Raw Data.vi"() -> ("Raw Data"=w817:refnum<class "Raw Data.lvclass">)  [unwired: 6 in, 1 out]
                n527 = call "create Data.vi"() -> ("Data"=w814:refnum<class "Data.lvclass">)  [unwired: 6 in, 1 out]
                n528 = call "create Data.vi"() -> ("Data"=w813:refnum<class "Data.lvclass">)  [unwired: 6 in, 1 out]
                n529 = call "create Data.vi"() -> ("Data"=w812:refnum<class "Data.lvclass">)  [unwired: 6 in, 1 out]
                n530 = for {
                  N: "Number Scans Y" -> [_]
                  tunnel: w817 -> [w846]
                  tunnel: w816 -> [w845]
                  tunnel: w815 -> [w844]
                  tunnel: w814 -> [w843]
                  tunnel: w813 -> [w836]
                  tunnel: w812 -> [w834]
                  tunnel: [w833] -> w811
                  tunnel: [w831] -> w807
                  tunnel: [w830] -> w810
                  tunnel: [w829] -> w809
                  tunnel: [w827] -> w808
                  tunnel: [w826] -> w805
                  n531 = call "get Raw Data.vi"("Camera Index"=0, "RawData in"=w846, "OCTDevice in"=w845) -> ("error out"=w839:errorcluster, "RawData out"=w841:refnum<class "Raw Data.lvclass">, "OCTDevice out"=w829:refnum<class "OCT Device.lvclass">)  [unwired: 2 in]
                  n532 = call-poly "set Processing Output.vi"("error in (no error)"=w839, "Data"=w843, "Processing"=w844) -> ("error out"=w840:errorcluster, "Data"=w837:refnum<class "Data.lvclass">, "Processing"=w842:refnum<class "Processing.lvclass">)  [unwired: 2 in]
                  n533 = call "execute Processing.vi"("error in (no error)"=w840, "Raw Data"=w841, "Processing"=w842) -> ("error out"=w838:errorcluster, "Raw Data"=w827:refnum<class "Raw Data.lvclass">)  [unwired: 2 in, 1 out]
                  n534 = call "append Data.vi"("error in (no error)"=w838, "Normal Direction"=Normal_Direction_Selection."Direction 3", "Data to append in"=w837, "Data in"=w836) -> ("error out"=w832:errorcluster, "Data to append out"=w830:refnum<class "Data.lvclass">, "Data out"=w835:refnum<class "Data.lvclass">)  [unwired: 1 in]
                  n535 = control-ref of="3D Surface"() -> (w825:refnum<vi>)
                  n536 = call "determine Surface.vi"("error in (no error)"=w832, "Surface Data in"=w834, "Data in"=w835) -> ("error out"=w826:errorcluster, "Surface Data out"=w831:refnum<class "Data.lvclass">, "Data out"=w833:refnum<class "Data.lvclass">)  [unwired: 2 in]
                  n537 = call-poly "display Data.vi"("Data in"=w831, "3D Surface Refnum"=w825) -> ()  [unwired: 3 in, 3 out]
                }
                n538 = call "stop Measurement.vi"("OCTDevice"=w809) -> ()  [unwired: 5 in, 2 out]
                n539 = call "clear Data.vi"("Data"=w811) -> ()  [unwired: 6 in, 1 out]
                n540 = call "clear Data.vi"("Data"=w810) -> ()  [unwired: 6 in, 1 out]
                n541 = call "clear Raw Data.vi"("Raw Data"=w808) -> ()  [unwired: 6 in, 1 out]
                n542 = local read "Probe"() -> (w803:refnum<class "Probe.lvclass">)
                n543 = call "determine Image Field.vi"("error in (no error)"=w805, "Probe in"=w803, "Surface Data in"=w807, "Scan Pattern in"=w796) -> ("error out"=w794:errorcluster, "Probe out"=w802:refnum<class "Probe.lvclass">, "Surface Data out"=w806:refnum<class "Data.lvclass">, "Scan Pattern out"=w795:refnum<class "Scan Pattern.lvclass">)
                n544 = call "clear Scan Pattern.vi"("error in (no error)"=w794, "Scan Pattern in"=w795) -> ("error out"=w793:errorcluster)  [unwired: 5 in]
                n545 = call "clear Data.vi"("error in (no error)"=w793, "Data"=w806) -> ()  [unwired: 5 in, 1 out]
                n546 = call "save Probe.vi"("error in (no error)"=w794, "Name"="Probe" ("name or relative path"), "Probe in"=w802) -> ()  [unwired: 3 in, 2 out]
              }
            }
            n547 = local write "Calibrate Surface"(w789) -> ()
          }
          event "SaveSpacingZ": Value Change {
            n548 = event-data() -> ()  [unwired: 1 in, 1 out]
            n549 = case shown="True" "SaveSpacingZ" {
              frame False {
              }
              frame True {
                n550 = Two Button Dialog(message="Writing a false SpacingZ value to your SpectralRadar.ini may seriously harm your sytem.\nAre you sure you want to continue?" ("Nachricht"), 1:"No" ("F-Schaltflächenname (\"Abbrechen\")"), 2:"Yes" ("T-Schaltflächenname (\"OK\")")) -> (T button?=w849:bool)
                n551 = case shown="True" w849 {
                  frame False {
                  }
                  frame True {
                    n552 = call "get Config Path.vi"() -> ("Path"=w853:path)  [unwired: 1 in, 1 out]
                    n553 = local read "Spacing Z [mm]"() -> (w857:dbl)
                    n554 = Build Path(base path=w853, name or relative path="SpectralRadar.ini" ("Name oder relativer Pfad")) -> (appended path=w863:path)
                    n555 = call <vilib>:"Open Config Data (compatibility).vi"("create file if necessary (T)"=FALSE ("create file if necessary? (T)"), "configuration file path"=w863) -> ("error out"=w856:errorcluster, "refnum"=w861:T26)  [unwired: 7 in, 1 out]
                    n556 = call-poly <vilib>:"Write Key.vi"("section"="Measure", "error in (no error)"=w856, "value"=w857, "key"="SpacingZ", "refnum"=w861) -> ("error out"=w855:errorcluster, "refnum out"=w858:T26)  [unwired: 4 in, 1 out]
                    n557 = call <vilib>:"Close Config Data.vi"("error in (no error)"=w855, "refnum"=w858) -> ("error out"=w854:errorcluster)  [unwired: 8 in, 1 out]
                    n558 = call <vilib>:"Simple Error Handler.vi"("error in (no error)"=w854) -> ()  [unwired: 4 in, 5 out]
                  }
                }
                n559 = local write "SaveSpacingZ"(FALSE ("SaveSpacingZ")) -> ()
              }
            }
          }
          event "Intensity Ring Light": Value Change {
            n560 = event-data() -> ()  [unwired: 1 in, 1 out]
            n561 = disable-structure shown="Disabled" {
              frame Disabled {
                n562 = call "set Ring Light Intensity.vi"() -> ()  [unwired: 3 in, 2 out]
              }
              frame Enabled {
              }
            }
            n563 = call "set Output Device Value by Name.vi"("Value"="Intensity Ring Light", "Identifier"="ring light", "OCTDevice"=w865) -> ("error out"=w866:errorcluster)  [unwired: 3 in, 1 out]
            n564 = call <vilib>:"Simple Error Handler.vi"("error in (no error)"=w866) -> ()  [unwired: 4 in, 5 out]
          }
          event "Options": Value Change {
            n565 = event-data() -> ()  [unwired: 1 in, 1 out]
            n566 = case shown="True" "Options" {
              tunnel: w870 -> [_ w874]
              tunnel: w869 -> [_ w873]
              frame False {
              }
              frame True {
                n567 = local read "Probe"() -> (w872:refnum<class "Probe.lvclass">)
                n568 = call "Options Dialog.vi"("GalvoControl"=w872, "Processing"=w873, "OCT Device"=w874) -> ()  [unwired: 1 in]
              }
            }
          }
          event "QuitApp": Mouse Enter {
            n569 = event-data() -> ("Time"=w876:u32)  [unwired: 1 in]
            n570 = Tick Count (ms)() -> (millisecond timer value=w879:u32)
            n571 = Subtract(x=w879, y=w876) -> (x-y=w878:u32)
            n572 = Less?(x=w878, y=u32 500) -> (x < y?=w875:bool)
            n573 = case shown="True" w875 {
              frame False {
              }
              frame True {
                w880 = u32 16448250
                n574 = Bundle(u32 8978432, w880) -> (w882:cluster{u32, u32})  [unwired: 1 in]
                n575 = Bundle(u32 16711680, u32 16448250) -> (w883:cluster{u32, u32})  [unwired: 1 in]
                n576 = Build Array(w883, w882) -> (w881:cluster{u32, u32}[])
                n577 = property on="QuitApp" class="Bool (strict)"("Colors [4]"=w881, "BoolText.TextColor"=w880) -> ()  [unwired: 2 in, 2 out]
              }
            }
          }
          event "QuitApp": Mouse Leave {
            w887 = u32 0
            n578 = event-data() -> ()  [unwired: 1 in, 4 out]
            n579 = Bundle(u32 12369084, u32 0) -> (w890:cluster{u32, u32})  [unwired: 1 in]
            n580 = Bundle(u32 9868950, w887) -> (w889:cluster{u32, u32})  [unwired: 1 in]
            n581 = Build Array(w890, w889) -> (w888:cluster{u32, u32}[])
            n582 = property on="QuitApp" class="Bool (strict)"("Colors [4]"=w888, "BoolText.TextColor"=w887) -> ()  [unwired: 2 in, 2 out]
          }
          event "OffsetErrors": Value Change {
            n583 = event-data() -> ()  [unwired: 1 in, 1 out]
            n584 = case shown="True" "OffsetErrors" {
              tunnel: w895 -> [_ w900]
              tunnel: w894 -> [_ w899]
              frame False {
              }
              frame True {
                n585 = local read "Camera #"() -> (w897:i32)
                n586 = call "measure Calibration.vi"("Camera Index"=w897, "Calibration Data"=Calibration_Selection."Offset Errors", "Processing"=w899, "OCTDevice"=w900) -> ()  [unwired: 2 in, 3 out]
              }
            }
          }
          event "SLD": Value Change {
            n587 = event-data() -> ()  [unwired: 1 in, 1 out]
            n588 = local write "SLDIndicator"("SLD") -> ()
            n589 = call "set Device Flag.vi"("Boolean"="SLD", "Device Property Flag Selection"=T5."SLD Status", "OCTDevice"=w903) -> ()  [unwired: 7 in, 2 out]
          }
        }
        n590 = local read "QuitApp"() -> (w119:bool)
      }
    }
    frame #3 {
      n591 = local read "Colored Data"() -> (w1027:refnum<class "Colored Data.lvclass">)
      n592 = local read "Processing"() -> (w1029:refnum<class "Processing.lvclass">)
      n593 = local read "Probe"() -> (w1030:refnum<class "Probe.lvclass">)
      n594 = local write "SLDIndicator"(FALSE ("Licht an (true) / aus (false)")) -> ()
      n595 = call "IMAQ Dispose"("All Images? (No)"=TRUE) -> ()  [unwired: 5 in, 1 out]
      n596 = call "close Probe.vi"("GalvoControl"=w1030) -> ()  [unwired: 6 in, 1 out]
      n597 = call "clear Processing.vi"("Processing"=w1029) -> ()  [unwired: 6 in, 1 out]
      n598 = call "clear Colored Data.vi"("Colored Data"=w1027) -> ()  [unwired: 6 in, 1 out]
    }
    frame #4 {
      n599 = call "close Device.vi"("OCTDevice"=w1033) -> ()  [unwired: 6 in, 1 out]
    }
    frame #5 {
      n600 = Quit LabVIEW(quit? (T)=FALSE) -> ()
    }
  }
